vi "Omniax_MotorDrive_XYZR_20100915.vi"() -> ()   [LabVIEW 2009]
uses:
  <vilib>/Utility/file.llb/Read From Spreadsheet File (DBL).vi
  <vilib>/Utility/file.llb/Read From Spreadsheet File (string).vi
  <vilib>/Instr/_visa.llb/VISA Configure Serial Port (Instr).vi
  <vilib>/Utility/file.llb/Write To Spreadsheet File (string).vi
  <vilib>/Utility/file.llb/Write To Spreadsheet File (DBL).vi
panel:
  out "Scanning":bool
  out "HOMING REQ":bool
  out "Laser Shutter":bool
  in  "SHUTTER SYNC":bool
  in  "Laser Shutter":bool
  out "LOOP REQ":bool
  out "#th loop":dbl
  in  "# of loops":dbl
  in  "LOOP":bool
  out "OP":bool
  out "CL":bool
  out "Valve \nopend/closed":bool
  in  "OK Button":bool
  out "STATUS":string
  in  "Delete Button":bool
  in  "String":string
  in  "Add Button":bool
  in  "Set Button":bool
  in  "Preset positions":i32(ring) items=["ZERO", "Default", "CDOSE", "QMS", "test", "test2", "test3", "yag position", "Sample Long Edge  ", "SPUTTER POS"]
  out "Presets":i32[][](array[numeric])
  out "X MINPOS":i32=-94296
  out "X MAXPOS":i32=-34296
  out "Y MINPOS":i32=-94296
  out "Y MAXPOS":i32=-34296
  out "R MAXPOS":i32=-34296
  out "R MINPOS":i32=-94296
  out "Z MINPOS":i32=-94296
  out "Z MAXPOS":i32=-34296
  in  "HARDSTOP":bool
  in  "GO":bool
  out "XYZR VEL PV Array":i32[](array[numeric])
  out "XYZ in RANGE Array":bool[](array[boolean])
  out "STEP SP Array":i32[](array[numeric])
  out "RUNHOLDArray":i32[](array[numeric])
  out "ZCONSTArray":dbl[](array[numeric])
  out "RCONSTArray":dbl[](array[numeric])
  out "XCONSTArray":dbl[](array[numeric])
  out "YCONSTArray":dbl[](array[numeric])
  out "Error Array":errorcluster[](array[cluster])
  out "COM PORT Array":refnum<visa-resource-name>[](array[refnum])
  out "Z COM PORT":refnum<visa-resource-name>="COM6"
  in  "Tab Control 3":enum32{"Status", "Reset"}(tab)
  out "Y in Range":bool
  out "Y Scan":bool
  out "Y in Motion":bool
  out "Y Backlash corr":bool
  out "X  in Range":bool
  out "X Scan":bool
  out "X  in Motion":bool
  out "X Backlash corr":bool
  out "Z in Range":bool
  out "Z Scan":bool
  out "Z in Motion":bool
  out "Z Backlash corr":bool
  out "R in Range":bool
  out "R Scan":bool
  out "R in Motion":bool
  out "R Backlash corr":bool
  out "X Ready":bool
  out "Y Ready":bool
  out "Z Ready":bool
  out "R Ready":bool
  in  "Reset Y Position mm":dbl
  out "Reset Y Motor Steps":i32
  in  "Reset X Position mm":dbl
  out "Reset X Motor Steps":i32
  in  "Reset Z Position mm":dbl
  out "Reset Z Motor Steps":i32
  in  "Reset R Position deg":dbl
  out "Reset R Motor Steps":i32
  in  "Reset":bool
  in  "Tab Control 2":enum32{"mm", "step"}(tab)
  in  "X Scan Length SP mm":dbl
  in  "X Scan Velocity SP mm/sec":dbl
  in  "Y Scan Length SP mm":dbl
  in  "Y Scan Velocity SP mm/sec":dbl
  in  "Review Scan \nParameters":bool
  in  "Z Scan Length SP mm":dbl
  in  "Z Scan Velocity SP mm/sec":dbl
  in  "R Scan Length SP deg":dbl
  in  "R Scan Velocity SP deg/sec":dbl
  in  "Z as dominating length":bool
  in  "X Scan Velocity SP steps/sec":i32=1 min=1 max=102400 step=1
  in  "X Scan Length SP steps":i32 min=-2304000 max=2304000 step=100
  out "X Scan length MV mm":dbl
  out "X Scan velocity MV mm/sec":dbl format="%#_6f"
  in  "Y Scan Velocity SP steps/sec":i32=1 min=1 max=102400 step=1
  in  "Y Scan Length SP steps":i32 min=-2304000 max=2304000 step=100
  out "Y Scan length MV mm":dbl
  out "Y Scan velocity MV mm/sec":dbl format="%#_6f"
  in  "Z Scan Velocity SP steps/sec":i32=1 min=1 max=204800 step=1
  in  "Z Scan Length SP steps":i32 min=0 max=102400000 step=100
  out "Z Scan length MV mm":dbl
  out "Z Scan velocity MV mm/sec":dbl format="%#_6f"
  in  "R Scan Velocity SP steps/sec":i32=1 min=1 max=102400 step=1
  in  "R Scan Length SP steps":i32 min=-6144000 max=0 step=100
  out "R Scan length MV deg":dbl
  out "R Scan velocity MV deg/sec":dbl format="%#_6f"
  out "atan Y/Z":dbl
  in  "Tab Control":enum32{"mm", "step"}(tab)
  in  "X Position SP mm":dbl
  in  "X Velocity SP mm/sec":dbl
  in  "X Move Set":bool
  in  "Y Move Set":bool
  in  "Y Position SP mm":dbl
  in  "Y Velocity SP mm/sec":dbl
  in  "Z Position SP mm":dbl
  in  "Z Velocity SP mm/sec":dbl
  in  "Z Move Set":bool
  in  "R Position SP deg":dbl
  in  "R Velocity SP deg/sec":dbl
  in  "R Move Set":bool
  in  "X Velocity SP step/sec":i32 min=1 max=128000
  out "X Velocity MV mm/sec":dbl
  in  "Y Velocity SP step/sec":i32 min=1 max=128000
  out "Y Velocity MV mm/sec":dbl
  in  "Z Velocity SP step/sec":i32 min=1 max=204800
  out "Z Velocity MV mm/sec":dbl
  in  "R Velocity SP step/sec":i32 min=1 max=20000
  out "R Velocity MVdeg/sec":dbl
  in  "Y Step SP":i32=-20000 min=-2304000 max=2304000 step=500
  out "Y Position MV mm":dbl
  in  "X Step SP":i32=-20000 min=-2304000 max=2304000 step=500
  out "X Position MV mm":dbl
  in  "Z Step SP":i32=-20000 min=0 max=102400000 step=500
  out "Z Position MV mm":dbl
  in  "R Step SP":i32=-20000 min=-6144000 max=0 step=500
  out "R Position MV deg":dbl
  out "X Step PV":i32 max=2000
  out "Y Step PV":i32 max=2000
  out "Z Step PV":i32 max=2000
  out "R Step PV":i32 max=2000
  in  "Clear ZY":bool
  out "ZY Graph":cluster{dbl[], dbl[]}(graph)
  out "ZR Graph":cluster{"Y":dbl[], "Y":dbl[]}[](graph)
  out "XY Graph":cluster{"Y":dbl[], "Y":dbl[]}[](graph)
  out "X Scan Duration":dbl
  out "Y Scan Duration":dbl
  out "Z Scan Duration":dbl
  out "R Scan Duration":dbl
  out "R Backlash steps/sec":i32
  out "R Backlash":i32
  out "R Holding Current %":i32
  out "R Run Current %":i32
  out "R offset deg":dbl
  out "R deg/rev":dbl
  out "R steps/rev":u32
  out "R velocity PV step/sec":i32
  out "R COM PORT":refnum<visa-resource-name>="COM5"
  out "R Position deg PV":dbl
  out "Z Backlash steps/sec":i32
  out "Z Backlash":i32
  out "Z Holding Current %":i32
  out "Z Run Current %":i32
  out "Z offset mm":dbl
  out "Z mm/rev":dbl
  out "Z steps/rev":u32
  out "Z  velocity PV step/sec":i32
  out "Z Position mm PV":dbl
  out "X Position mm PV":dbl
  out "X velocity PV step/sec":i32
  in  "Set scan parameter":bool
  out "X Backlash steps/sec":i32
  out "X Backlash":i32
  out "X Holding Current %":i32
  out "X Run Current %":i32
  out "X offset mm":dbl
  out "X mm/rev":dbl
  out "X steps/rev":u32
  out "X COM PORT":refnum<visa-resource-name>="COM5"
  out "Y Backlash steps/sec":i32
  out "Y Backlash":i32
  out "Y Holding Current %":i32
  out "Y Run Current %":i32
  in  "Scan Cancel":bool
  out "Y Position mm PV":dbl
  out "Y offset mm":dbl
  out "Y mm/rev":dbl
  out "Y steps/rev":u32
  out "Y velocity PV step/sec":i32
  in  "Scan Go":bool
  in  "Stop":bool
  out "Y COM PORT":refnum<visa-resource-name>="COM5"
  # "MX"
  # "MY"
  # "MZ"
  # "MR"
  # "Indicators"
  # "L"
  # "M"
  # "B"
  # "S"
  # "R"
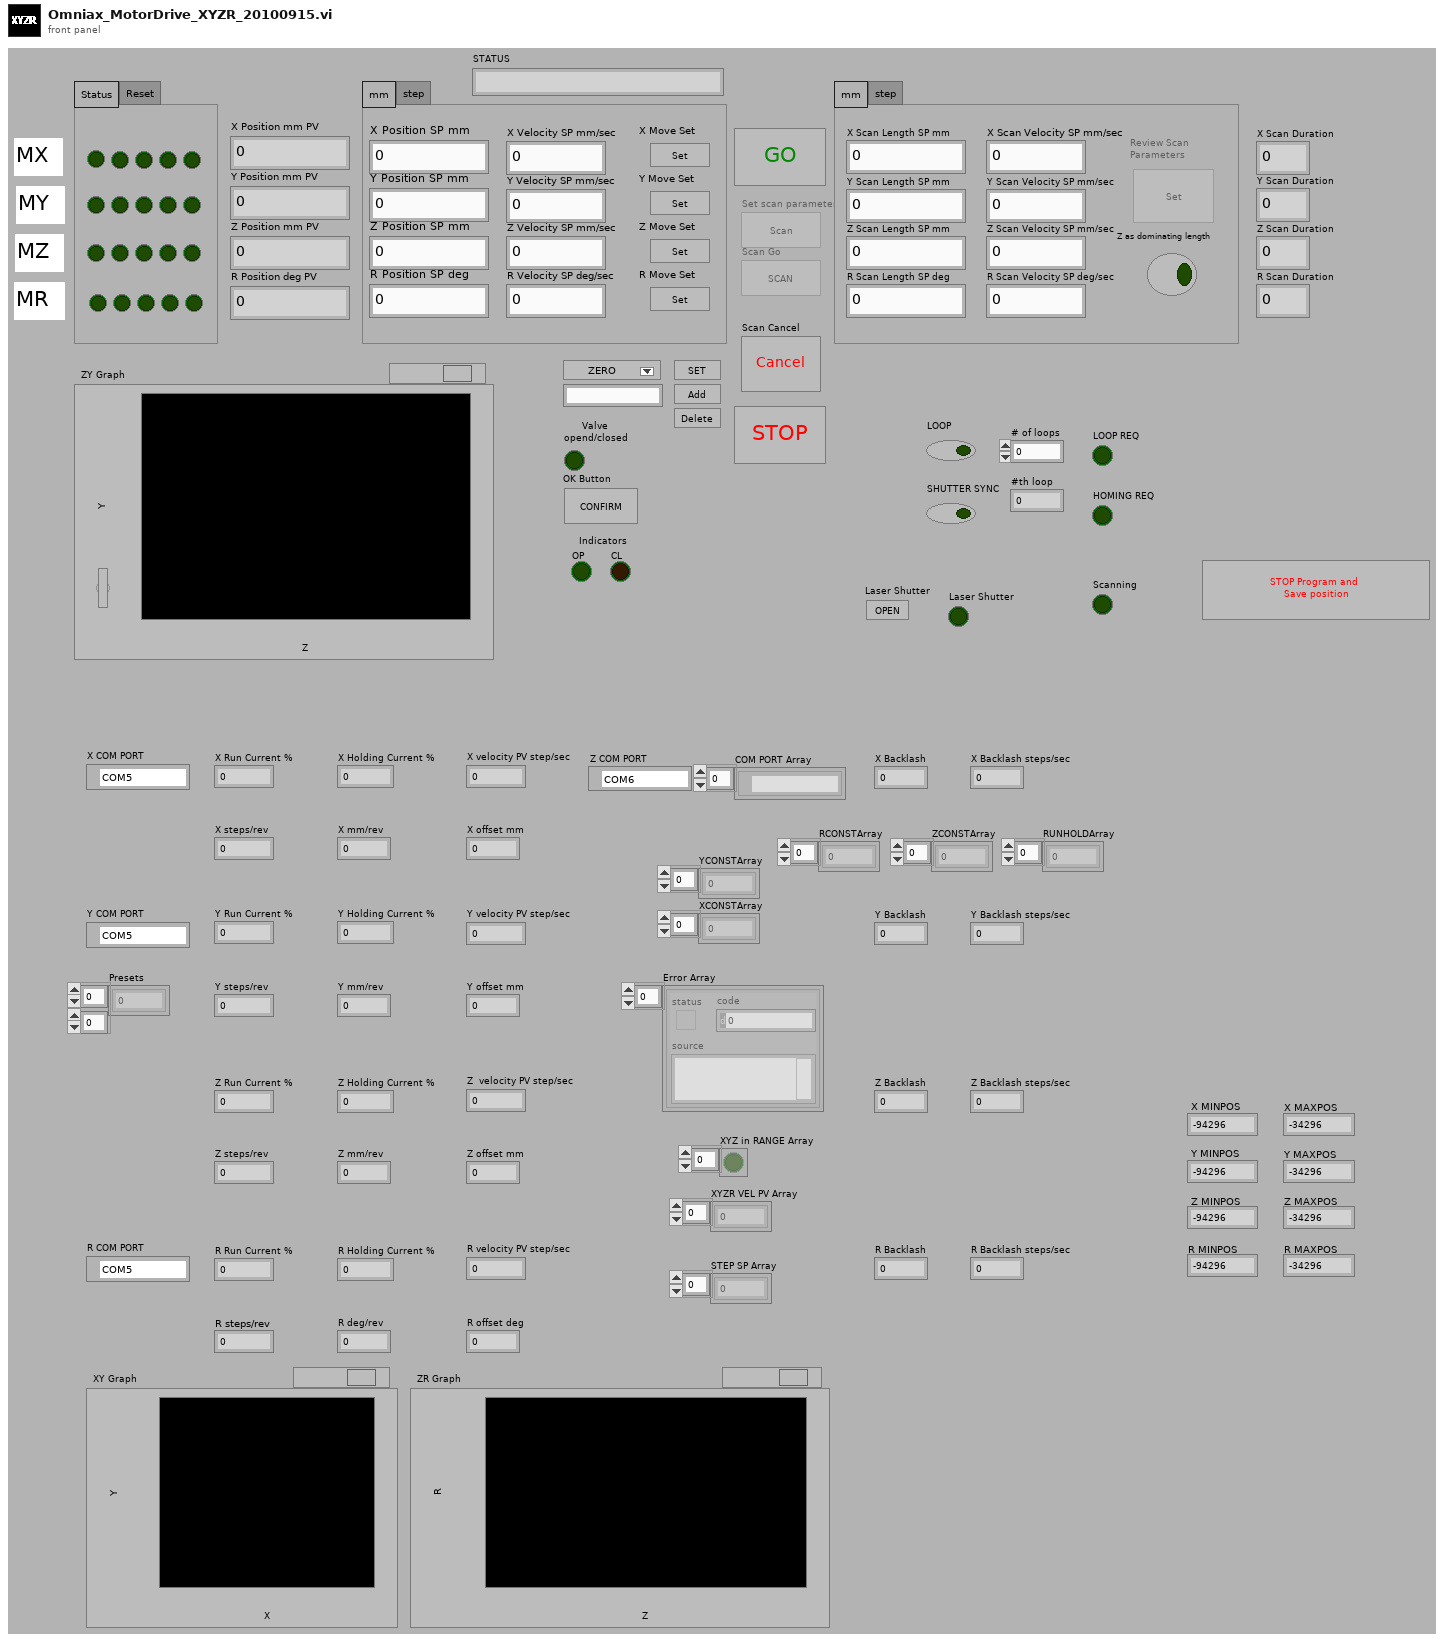
[diagram p1: front panel]
types:
  T1 = enum8{"Enabled", "Disabled", "Disabled and Grayed Out"}
  T2 = cluster{"[0]":i32, "[1]":i32, "[2]":i32, "[3]":i32, "[4]":i32, "[5]":i32, "[6]":i32, "[7]":i32, "[8]":i32}
  T3 = cluster{"XY Max Min array OUT[0]":dbl, "XY Max Min array OUT[1]":dbl, "XY Max Min array OUT[2]":dbl, "XY Max Min array OUT[3]":dbl, "XY Max Min array OUT[4]":dbl, "XY Max Min array OUT[5]":dbl, "XY Max Min array OUT[6]":dbl, "XY Max Min array OUT[7]":dbl, "XY Max Min array OUT[8]":dbl}
  T4 = cluster{"COM PORT Array OUT[0]":refnum<visa-resource-name>, "COM PORT Array OUT[1]":refnum<visa-resource-name>, "COM PORT Array OUT[2]":refnum<visa-resource-name>, "COM PORT Array OUT[3]":refnum<visa-resource-name>, "COM PORT Array OUT[4]":refnum<visa-resource-name>, "COM PORT Array OUT[5]":refnum<visa-resource-name>, "COM PORT Array OUT[6]":refnum<visa-resource-name>, "COM PORT Array OUT[7]":refnum<visa-resource-name>, "COM PORT Array OUT[8]":refnum<visa-resource-name>}
  T5 = cluster{"STEP SP Array OUT[0]":i32, "STEP SP Array OUT[1]":i32, "STEP SP Array OUT[2]":i32, "STEP SP Array OUT[3]":i32, "STEP SP Array OUT[4]":i32, "STEP SP Array OUT[5]":i32, "STEP SP Array OUT[6]":i32, "STEP SP Array OUT[7]":i32, "STEP SP Array OUT[8]":i32}
  T6 = cluster{"XYZ in RANGE Array OUT[0]":bool, "XYZ in RANGE Array OUT[1]":bool, "XYZ in RANGE Array OUT[2]":bool, "XYZ in RANGE Array OUT[3]":bool, "XYZ in RANGE Array OUT[4]":bool, "XYZ in RANGE Array OUT[5]":bool, "XYZ in RANGE Array OUT[6]":bool, "XYZ in RANGE Array OUT[7]":bool, "XYZ in RANGE Array OUT[8]":bool}
  T7 = cluster{"XYZR VEL PV Array OUT[0]":i32, "XYZR VEL PV Array OUT[1]":i32, "XYZR VEL PV Array OUT[2]":i32, "XYZR VEL PV Array OUT[3]":i32, "XYZR VEL PV Array OUT[4]":i32, "XYZR VEL PV Array OUT[5]":i32, "XYZR VEL PV Array OUT[6]":i32, "XYZR VEL PV Array OUT[7]":i32, "XYZR VEL PV Array OUT[8]":i32}
  T8 = cluster{"XYZR MAX MIN POS[0]":i32, "XYZR MAX MIN POS[1]":i32, "XYZR MAX MIN POS[2]":i32, "XYZR MAX MIN POS[3]":i32, "XYZR MAX MIN POS[4]":i32, "XYZR MAX MIN POS[5]":i32, "XYZR MAX MIN POS[6]":i32, "XYZR MAX MIN POS[7]":i32, "XYZR MAX MIN POS[8]":i32}
  T9 = cluster{"Error Array OUT[0]":errorcluster, "Error Array OUT[1]":errorcluster, "Error Array OUT[2]":errorcluster, "Error Array OUT[3]":errorcluster, "Error Array OUT[4]":errorcluster, "Error Array OUT[5]":errorcluster, "Error Array OUT[6]":errorcluster, "Error Array OUT[7]":errorcluster, "Error Array OUT[8]":errorcluster}
  T10 = enum16{"Stop", "Reset", "Run Current", "Holding Current", "Accel Rate", "Decel Rate", "Move to Relative Position", "Move to Absolute Position", "Echo Mode", "Print Parameter", "Send String", "Microstep Resolution", "Set Current Position", "Max Velocity"}
  T11 = cluster{"Presets[0]":i32, "Presets[1]":i32, "Presets[2]":i32, "Presets[3]":i32, "Presets[4]":i32, "Presets[5]":i32, "Presets[6]":i32, "Presets[7]":i32, "Presets[8]":i32}
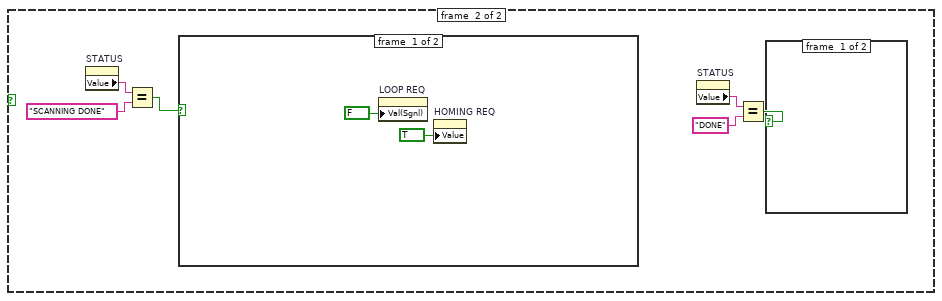
[diagram p4: hidden frame]
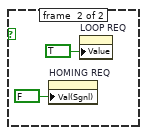
[diagram p5: hidden frame]
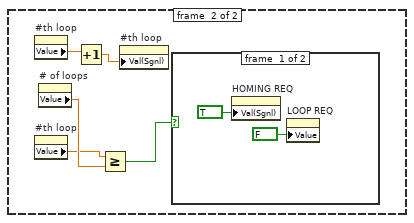
[diagram p6: hidden frame]
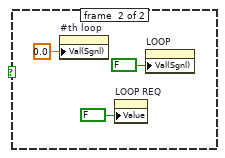
[diagram p7: hidden frame]
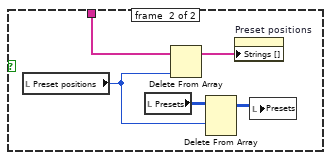
[diagram p8: hidden frame]
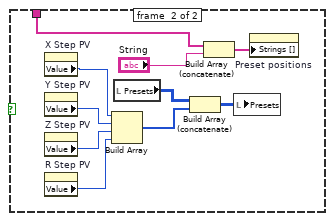
[diagram p9: hidden frame]
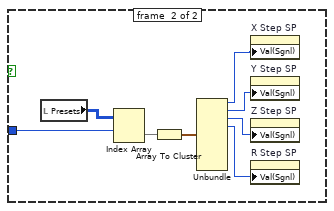
[diagram p10: hidden frame]
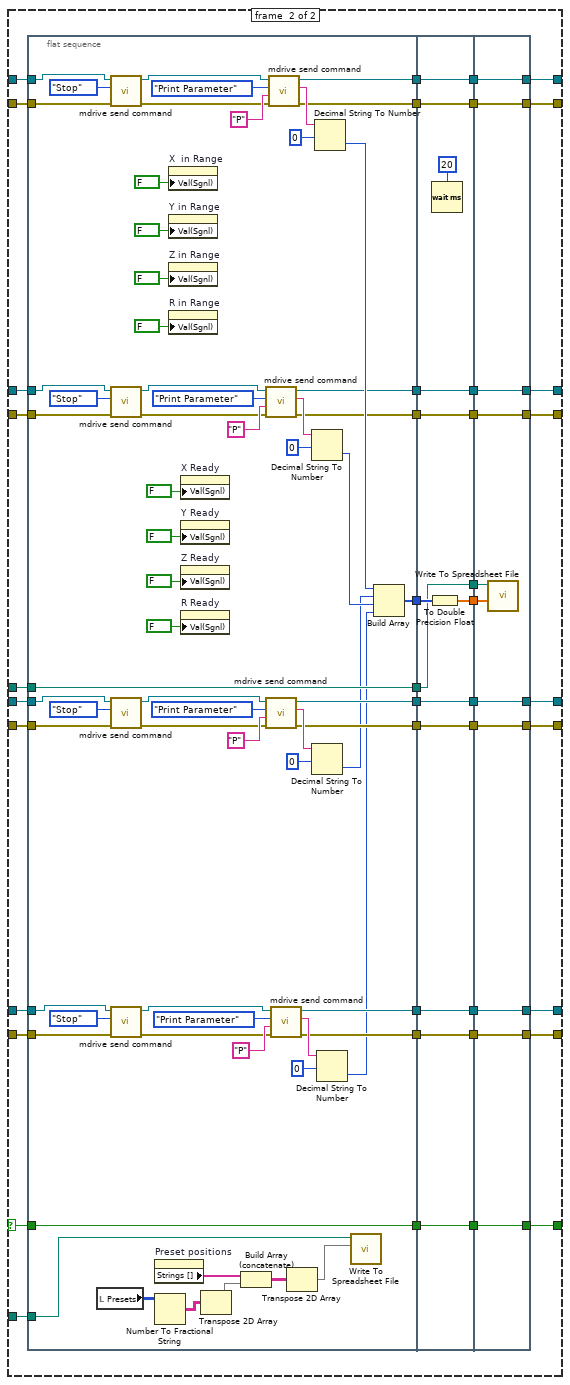
[diagram p11: hidden frame]
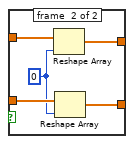
[diagram p12: hidden frame]
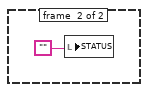
[diagram p14: hidden frame]
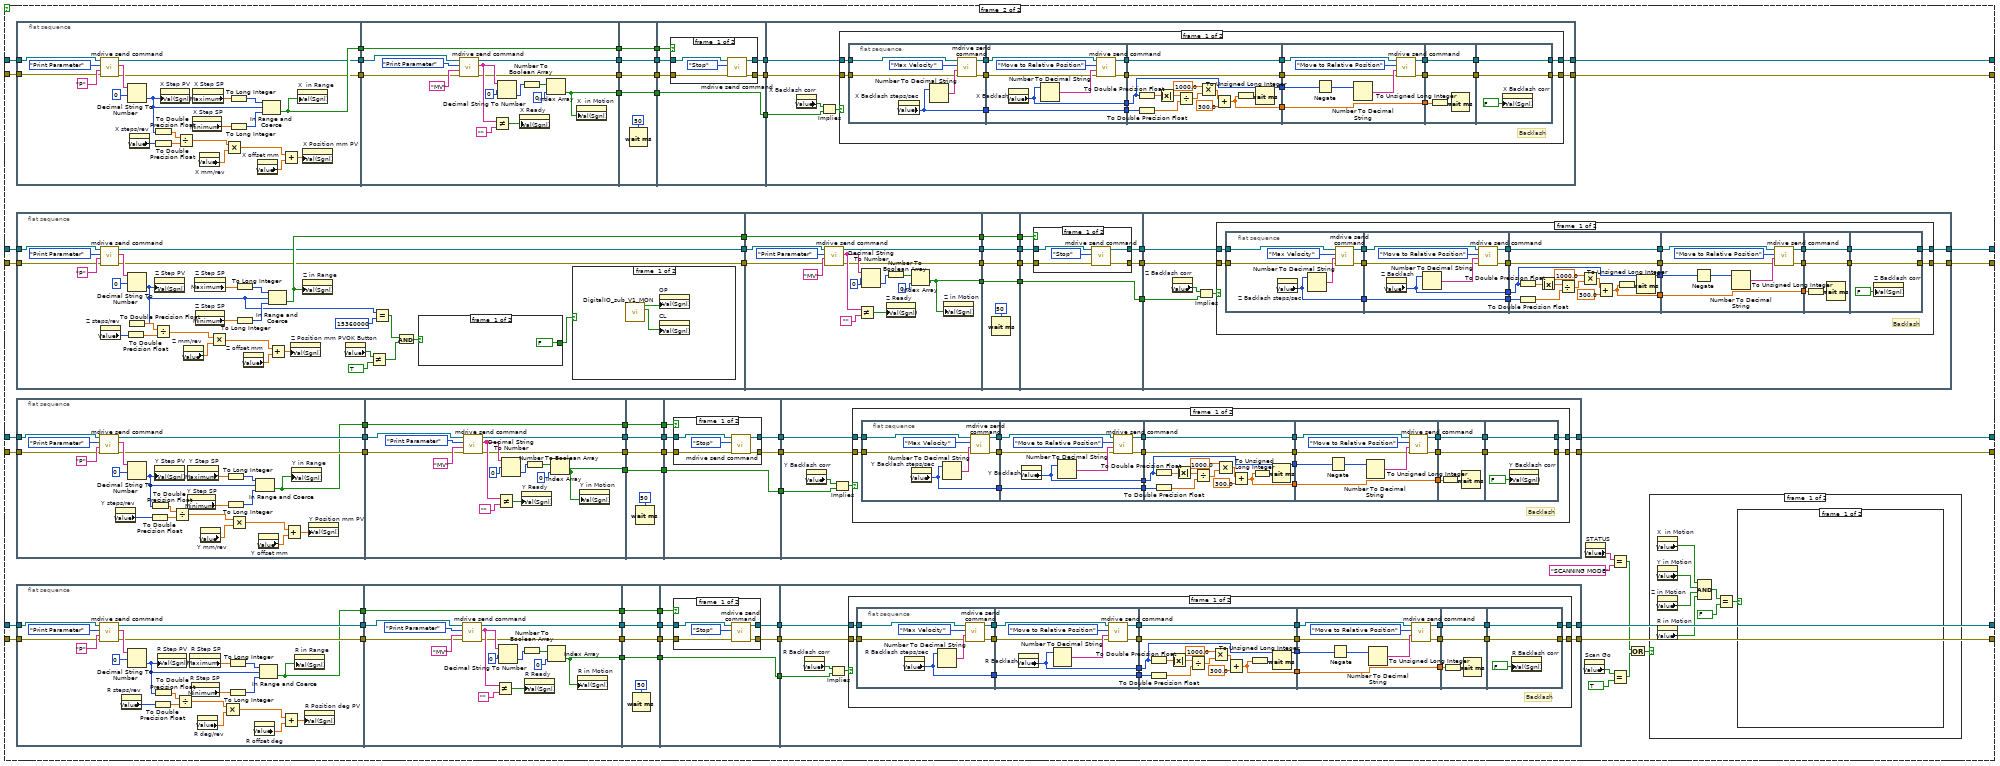
[diagram p15: hidden frame]
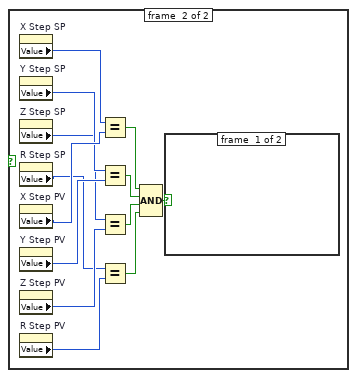
[diagram p16: hidden frame]
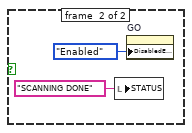
[diagram p17: hidden frame]
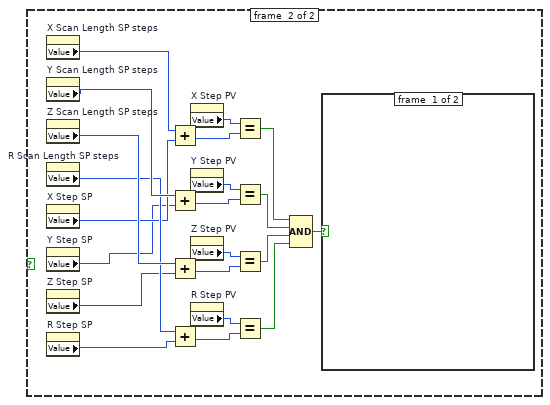
[diagram p18: hidden frame]
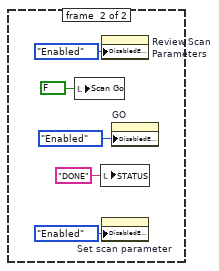
[diagram p19: hidden frame]
diagram:
  n1 = flat-sequence {
    tunnel: [w53] -> w36
    frame #0 {
      w51 = 0.2 ("MM/rev")
      w56 = u32 51200 ("step/rev")
      w58 = 128000 ("Value (Signaling)")
      w59 = 1.0 ("Data Entry Limits:Minimum")
      w52 = 0.0 ("offset")
      # "a=1000000"
      n2 = To Double Precision Float(number=w58) -> (double precision float=w50:dbl)
      n3 = To Double Precision Float(number=w56) -> (double precision float=w61:dbl)
      n4 = property on="X Velocity SP step/sec" class="DigNum (strict)"("Val(Sgnl)"=w58) -> ()  [unwired: 2 in, 2 out]
      n5 = property on="X Velocity SP step/sec" class="DigNum (strict)"("Minimum"=w59) -> ()  [unwired: 2 in, 2 out]
      n6 = Divide(x=w50, y=w61) -> (x/y=w60:dbl)
      n7 = property on="X Velocity SP step/sec" class="DigNum (strict)"("Maximum"=w50) -> ()  [unwired: 2 in, 2 out]
      n8 = Multiply(x=w60, y=w51) -> (x*y=w54:dbl)
      n9 = property on="X Velocity SP mm/sec" class="DigNum (strict)"("Val(Sgnl)"=w54) -> ()  [unwired: 2 in, 2 out]
      n10 = To Double Precision Float(number=w56) -> (double precision float=w55:dbl)
      n11 = To Double Precision Float(number=w58) -> (double precision float=w57:dbl)
      n12 = Build Array(w59, w57, w55, w54, w50, w51, w52) -> (w53:dbl[])
      "X offset mm" <- w52
      "X steps/rev" <- w56
      "X mm/rev" <- w51
    }
  }
  n13 = flat-sequence {
    tunnel: [w62] -> w35
    frame #0 {
      w71 = 1.0 ("Data Entry Limits:Minimum")
      w65 = 0.0 ("R offset deg")
      w66 = -3.0 ("R deg/rev")
      w69 = u32 51200 ("step/rev")
      w70 = 20000 ("Value (Signaling)")
      n14 = To Double Precision Float(number=w69) -> (double precision float=w72:dbl)
      n15 = To Double Precision Float(number=w70) -> (double precision float=w68:dbl)
      n16 = property on="R Velocity SP step/sec" class="DigNum (strict)"("Minimum"=w71) -> ()  [unwired: 2 in, 2 out]
      n17 = property on="R Velocity SP step/sec" class="DigNum (strict)"("Val(Sgnl)"=w70) -> ()  [unwired: 2 in, 2 out]
      n18 = Divide(x=w68, y=w72) -> (x/y=w74:dbl)
      n19 = property on="R Velocity SP step/sec" class="DigNum (strict)"("Maximum"=w68) -> ()  [unwired: 2 in, 2 out]
      n20 = Multiply(x=w74, y=w66) -> (x*y=w73:dbl)
      n21 = Absolute Value(x=w73) -> (abs(x)=w67:dbl)
      n22 = property on="R Velocity SP deg/sec" class="DigNum (strict)"("Val(Sgnl)"=w67) -> ()  [unwired: 2 in, 2 out]
      n23 = To Double Precision Float(number=w69) -> (double precision float=w63:dbl)
      n24 = To Double Precision Float(number=w70) -> (double precision float=w64:dbl)
      n25 = Build Array(w71, w64, w63, w68, w67, w66, w65) -> (w62:dbl[])
      "R offset deg" <- w65
      "R deg/rev" <- w66
      "R steps/rev" <- w69
    }
  }
  n26 = flat-sequence {
    tunnel: [w75] -> w34
    frame #0 {
      w77 = 0.2 ("Z mm/rev")
      w81 = u32 51200 ("step/rev")
      w83 = 204800 ("Value (Signaling)")
      w84 = 1.0 ("Data Entry Limits:Minimum")
      w76 = 0.0 ("Z offset mm")
      n27 = To Double Precision Float(number=w81) -> (double precision float=w86:dbl)
      n28 = To Double Precision Float(number=w83) -> (double precision float=w79:dbl)
      n29 = property on="Z Velocity SP step/sec" class="DigNum (strict)"("Minimum"=w84) -> ()  [unwired: 2 in, 2 out]
      n30 = property on="Z Velocity SP step/sec" class="DigNum (strict)"("Val(Sgnl)"=w83) -> ()  [unwired: 2 in, 2 out]
      n31 = Divide(x=w79, y=w86) -> (x/y=w85:dbl)
      n32 = property on="Z Velocity SP step/sec" class="DigNum (strict)"("Maximum"=w79) -> ()  [unwired: 2 in, 2 out]
      n33 = Multiply(x=w85, y=w77) -> (x*y=w78:dbl)
      n34 = property on="Z Velocity SP mm/sec" class="DigNum (strict)"("Val(Sgnl)"=w78) -> ()  [unwired: 2 in, 2 out]
      n35 = To Double Precision Float(number=w83) -> (double precision float=w82:dbl)
      n36 = To Double Precision Float(number=w81) -> (double precision float=w80:dbl)
      n37 = Build Array(w84, w82, w80, w79, w78, w77, w76) -> (w75:dbl[])
      "Z offset mm" <- w76
      "Z mm/rev" <- w77
      "Z steps/rev" <- w81
    }
  }
  n38 = flat-sequence {
    tunnel: [w90] -> w37
    frame #0 {
      w88 = 0.2 ("MM/rev")
      w93 = u32 51200 ("step/rev")
      w95 = 128000 ("Value (Signaling)")
      w96 = 1.0 ("Data Entry Limits:Minimum")
      w89 = 0.0 ("offset")
      n39 = To Double Precision Float(number=w95) -> (double precision float=w87:dbl)
      n40 = To Double Precision Float(number=w93) -> (double precision float=w98:dbl)
      n41 = property on="Y Velocity SP step/sec" class="DigNum (strict)"("Val(Sgnl)"=w95) -> ()  [unwired: 2 in, 2 out]
      n42 = property on="Y Velocity SP step/sec" class="DigNum (strict)"("Minimum"=w96) -> ()  [unwired: 2 in, 2 out]
      n43 = Divide(x=w87, y=w98) -> (x/y=w97:dbl)
      n44 = property on="Y Velocity SP step/sec" class="DigNum (strict)"("Maximum"=w87) -> ()  [unwired: 2 in, 2 out]
      n45 = Multiply(x=w97, y=w88) -> (x*y=w91:dbl)
      n46 = To Double Precision Float(number=w95) -> (double precision float=w94:dbl)
      n47 = property on="Y Velocity SP mm/sec" class="DigNum (strict)"("Val(Sgnl)"=w91) -> ()  [unwired: 2 in, 2 out]
      n48 = To Double Precision Float(number=w93) -> (double precision float=w92:dbl)
      n49 = Build Array(w96, w94, w92, w91, w87, w88, w89) -> (w90:dbl[])
      "Y offset mm" <- w89
      "Y steps/rev" <- w93
      "Y mm/rev" <- w88
    }
  }
  n50 = local read "Z  velocity PV step/sec"() -> (w17:i32)
  n51 = local read "R velocity PV step/sec"() -> (w19:i32)
  n52 = local read "X velocity PV step/sec"() -> (w20:i32)
  n53 = local read "Y velocity PV step/sec"() -> (w18:i32)
  n54 = local read "X  in Range"() -> (w24:bool)
  n55 = local read "R in Range"() -> (w21:bool)
  n56 = local read "Y in Range"() -> (w23:bool)
  n57 = local read "Z in Range"() -> (w22:bool)
  n58 = property on="LOOP REQ" class="Bool (strict)"("Value"=FALSE ("LOOP MODE")) -> ()  [unwired: 2 in, 2 out]
  n59 = Build Array(w20, w18, w17, w19) -> (→"XYZR VEL PV Array":i32[])
  n60 = Build Array(w24, w23, w22, w21) -> (→"XYZ in RANGE Array":bool[])
  n61 = flat-sequence {
    tunnel: [w99] -> w33
    frame #0 {
      w102 = 20 ("R Holding Current %")
      w101 = 100 ("R Run Current %")
      w104 = 20 ("Holding Current %")
      w103 = 40 ("Run Current %")
      w106 = 20 ("Holding Current %")
      w107 = 40 ("Run Current %")
      w105 = 40 ("Z Run Current %")
      w100 = 20 ("Z Holding Current %")
      n62 = Build Array(w107, w106, w105, w104, w103, w102, w101, w100) -> (w99:i32[])
      "Z Holding Current %" <- w100
      "Z Run Current %" <- w105
      "X Run Current %" <- w107
      "X Holding Current %" <- w106
      "Y Run Current %" <- w103
      "Y Holding Current %" <- w104
      "R Holding Current %" <- w102
      "R Run Current %" <- w101
    }
  }
  n63 = Build Array("X Step SP", "Y Step SP", "Z Step SP", "R Step SP", "X Velocity SP step/sec", "Y Velocity SP step/sec", "Z Velocity SP step/sec", "R Velocity SP step/sec") -> (→"STEP SP Array":i32[])
  n64 = flat-sequence {
    frame #0 {
      n65 = property on="Z Scan" class="Bool (strict)"("Val(Sgnl)"=FALSE ("Value (Signaling)")) -> ()  [unwired: 2 in, 2 out]
      n66 = property on="R Velocity SP deg/sec" class="DigNum (strict)"("Val(Sgnl)"=0.1 ("Value (Signaling)")) -> ()  [unwired: 2 in, 2 out]
      n67 = property on="Z Scan Velocity SP mm/sec" class="DigNum (strict)"("Val(Sgnl)"=0.1 ("Value (Signaling)")) -> ()  [unwired: 2 in, 2 out]
      n68 = property on="X Scan" class="Bool (strict)"("Val(Sgnl)"=FALSE ("Value (Signaling)")) -> ()  [unwired: 2 in, 2 out]
      n69 = property on="R Scan" class="Bool (strict)"("Val(Sgnl)"=FALSE ("Value (Signaling)")) -> ()  [unwired: 2 in, 2 out]
      n70 = property on="Y Scan Velocity SP mm/sec" class="DigNum (strict)"("Val(Sgnl)"=0.1 ("Value (Signaling)")) -> ()  [unwired: 2 in, 2 out]
      n71 = property on="Y Scan" class="Bool (strict)"("Val(Sgnl)"=FALSE ("Value (Signaling)")) -> ()  [unwired: 2 in, 2 out]
      n72 = property on="X Scan Velocity SP mm/sec" class="DigNum (strict)"("Val(Sgnl)"=0.1 ("Value (Signaling)")) -> ()  [unwired: 2 in, 2 out]
      n73 = property on="Scan Go" class="Bool (strict)"("DisabledEnum"=T1."Disabled and Grayed Out" ("Disabled")) -> ()  [unwired: 2 in, 2 out]
      n74 = property on="Z Scan Velocity SP steps/sec" class="DigNum (strict)"("Minimum"=1.0 ("Data Entry Limits:Maximum")) -> ()  [unwired: 2 in, 2 out]
      n75 = property on="Z Scan Velocity SP steps/sec" class="DigNum (strict)"("Maximum"=204800.0 ("Data Entry Limits:Maximum")) -> ()  [unwired: 2 in, 2 out]
    }
  }
  n76 = flat-sequence {
    frame #0 {
      n77 = property on="R Backlash corr" class="Bool (strict)"("Val(Sgnl)"=FALSE ("Value (Signaling)")) -> ()  [unwired: 2 in, 2 out]
      n78 = property on="Y Backlash corr" class="Bool (strict)"("Val(Sgnl)"=FALSE ("Value (Signaling)")) -> ()  [unwired: 2 in, 2 out]
      n79 = property on="Z Backlash corr" class="Bool (strict)"("Val(Sgnl)"=FALSE ("Value (Signaling)")) -> ()  [unwired: 2 in, 2 out]
      n80 = property on="X Backlash corr" class="Bool (strict)"("Val(Sgnl)"=FALSE ("Value (Signaling)")) -> ()  [unwired: 2 in, 2 out]
      "Z Backlash steps/sec" <- 25600 ("Z Backlash steps/sec")
      "Z Backlash" <- -12800 ("Z Backlash")
      "X Backlash steps/sec" <- 25600 ("Value (Signaling)")
      "X Backlash" <- 5120 ("Backlash2")
      "Y Backlash" <- -5120 ("Backlash2")
      "Y Backlash steps/sec" <- 25600 ("Value (Signaling)")
      "R Backlash steps/sec" <- 6400 ("R Backlash steps/sec")
      "R Backlash" <- -12800 ("R Backlash")
    }
  }
  n81 = flat-sequence {
    tunnel: [w225] -> w13
    tunnel: [w224] -> w12
    tunnel: [w223] -> w11
    tunnel: [w222] -> w10
    tunnel: [w221] -> w9
    tunnel: [w220] -> w8
    tunnel: [w219] -> w7
    tunnel: [w218] -> w6
    tunnel: [w215] -> w5
    tunnel: [w185] -> w4
    frame #0 {
      w185 = path "C:/Documents and Settings/b_ogasawara/Desktop/lv1/LV codes/IMS/PRESET.TXT"
      w183 = 0 ("element")
      w215 = path "C:/Documents and Settings/b_ogasawara/Desktop/lv1/LV codes/IMS/POS.TXT"
      w245 = refnum<visa-resource-name> "COM7" ("COM PORT")
      w246 = refnum<visa-resource-name> "COM5" ("COM PORT")
      w247 = refnum<visa-resource-name> "COM6" ("VISA resource name")
      w248 = refnum<visa-resource-name> "COM4" ("COM PORT")
      n82 = Build Array(w248, w247, w246, w245) -> (w243:refnum<visa-resource-name>[])
      n83 = for {
        N: 4 -> [_]
        tunnel: w243 -> [w251] mode=indexing
        tunnel: [w250] -> w241 mode=indexing
        tunnel: [w249] -> w242 mode=indexing
        w253 = u16 0 items=["None", "XON/XOFF", "RTS/CTS", "XON/XOFF & RTS/CTS", "DTR/DSR", "XON/XOFF & DTR/DSR"] ("flow control (0:none)")
        w254 = u16 10 items=["1.0"=10, "1.5"=15, "2.0"=20] ("stop bits (10: 1 bit)")
        # "Stop bits"
        n84 = call-poly "VISA Configure Serial Port"("VISA resource name"=w251, "timeout (10sec)"=u32 10000, "baud rate (9600)"=u32 9600, "data bits (8)"=u16 8, "parity (0:none)"=enum16{"None", "Odd", "Even", "Mark", "Space"}."None", "stop bits (10: 1 bit)"=w254, "flow control (0:none)"=w253) -> ("VISA resource name out"=w250:refnum<visa-resource-name>, "error out"=w249:errorcluster)  [unwired: 7 in]
      }
      "COM PORT Array" <- w241
      "Error Array" <- w242
      n85 = local write "STATUS"("INITIALIZING" ("STATUS")) -> ()
      n86 = call-poly <vilib>:"Read From Spreadsheet File.vi"("file path (dialog if empty)"=w215) -> ("first row"=w216:dbl[])  [unwired: 6 in, 4 out]
      n87 = call "DigitalIO_sub_V1_MON.vi"() -> ("CL"=w142:bool, "OP"=w143:bool)  [unwired: 8 in]
      n88 = To Long Integer(number=w216) -> (32bit integer=w182:i32[])
      n89 = property on="CL" class="Bool (strict)"("Val(Sgnl)"=w142) -> ()  [unwired: 2 in, 2 out]
      n90 = property on="OP" class="Bool (strict)"("Val(Sgnl)"=w143) -> ()  [unwired: 2 in, 2 out]
      n91 = Array To Cluster(array=w182) -> (cluster=w181:T2)
      n92 = property on="Z Step SP" class="DigNum (strict)"() -> ("Maximum"=w140:dbl)  [unwired: 2 in, 2 out]
      n93 = property on="R Step SP" class="DigNum (strict)"() -> ("Maximum"=w138:dbl)  [unwired: 2 in, 2 out]
      n94 = property on="R Step SP" class="DigNum (strict)"() -> ("Minimum"=w139:dbl)  [unwired: 2 in, 2 out]
      n95 = property on="Z Step SP" class="DigNum (strict)"() -> ("Minimum"=w141:dbl)  [unwired: 2 in, 2 out]
      n96 = Unbundle(w181) -> ("[0]"=w157:i32, "[1]"=w158:i32, "[2]"=w159:i32, "[3]"=w160:i32)  [unwired: 5 out]
      n97 = Build Array(w140, w141, w138, w139) -> (w137:dbl[])
      n98 = property on="Reset X Motor Steps" class="DigNum (strict)"("Val(Sgnl)"=w157) -> ()  [unwired: 2 in, 2 out]
      n99 = property on="Reset Y Motor Steps" class="DigNum (strict)"("Val(Sgnl)"=w158) -> ()  [unwired: 2 in, 2 out]
      n100 = property on="Reset Z Motor Steps" class="DigNum (strict)"("Val(Sgnl)"=w159) -> ()  [unwired: 2 in, 2 out]
      n101 = property on="Reset R Motor Steps" class="DigNum (strict)"("Val(Sgnl)"=w160) -> ()  [unwired: 2 in, 2 out]
      n102 = local read "XYZ in RANGE Array"() -> (w237:bool[])
      n103 = local read "XYZR VEL PV Array"() -> (w236:i32[])
      n104 = local read "RUNHOLDArray"() -> (w235:i32[])
      n105 = local read "STEP SP Array"() -> (w238:i32[])
      n106 = call-poly <vilib>:"Read From Spreadsheet File.vi"("file path (dialog if empty)"=w185) -> ("all rows"=w190:string[][])  [unwired: 6 in, 4 out]
      n107 = Transpose 2D Array(2D array=w190) -> (transposed array=w189:string[][])
      n108 = property on="R steps/rev" class="DigNum (strict)"() -> ("Value"=w153:u32)  [unwired: 2 in, 2 out]
      n109 = property on="X steps/rev" class="DigNum (strict)"() -> ("Value"=w156:u32)  [unwired: 2 in, 2 out]
      n110 = property on="Y steps/rev" class="DigNum (strict)"() -> ("Value"=w155:u32)  [unwired: 2 in, 2 out]
      n111 = property on="Z steps/rev" class="DigNum (strict)"() -> ("Value"=w154:u32)  [unwired: 2 in, 2 out]
      n112 = Delete From Array(array=w189, index (row)=0) -> (deleted portion=w184:string[], array with subset deleted=w187:string[][])  [unwired: 2 in]
      n113 = call "InitializeMotorsXYZR_V2.vi"("COM PORT Array IN"=w241, "STEP SP Array IN"=w238, "XYZ in RANGE Array IN"=w237, "XYZR VEL PV Array IN"=w236, "RUNHOLDArray IN"=w235, "Error Array IN"=w242, "ZR Max Min array"=w137) -> ("XY Max Min array OUT"=w136:dbl[], "COM PORT Array OUT"=w240:refnum<visa-resource-name>[], "STEP SP Array OUT"=w234:i32[], "XYZ in RANGE Array OUT"=w233:bool[], "XYZR VEL PV Array OUT"=w232:i32[], "XYZR MAX MIN POS"=w217:i32[], "Error Array OUT"=w239:errorcluster[])  [unwired: 6 in]
      n114 = Array To Cluster(array=w136) -> (cluster=w135:T3)
      n115 = Unbundle(w135) -> ("XY Max Min array OUT[0]"=w134:dbl, "XY Max Min array OUT[1]"=w132:dbl, "XY Max Min array OUT[2]"=w131:dbl, "XY Max Min array OUT[3]"=w133:dbl)  [unwired: 5 out]
      n116 = To Double Precision Float(number=w160) -> (double precision float=w166:dbl)
      n117 = To Double Precision Float(number=w153) -> (double precision float=w165:dbl)
      n118 = To Double Precision Float(number=w159) -> (double precision float=w170:dbl)
      n119 = To Double Precision Float(number=w154) -> (double precision float=w169:dbl)
      n120 = To Double Precision Float(number=w158) -> (double precision float=w174:dbl)
      n121 = To Double Precision Float(number=w155) -> (double precision float=w173:dbl)
      n122 = To Double Precision Float(number=w157) -> (double precision float=w178:dbl)
      n123 = To Double Precision Float(number=w156) -> (double precision float=w177:dbl)
      n124 = property on="R deg/rev" class="DigNum (strict)"() -> ("Value"=w149:dbl)  [unwired: 2 in, 2 out]
      n125 = property on="X Step SP" class="DigNum (strict)"("Maximum"=w134) -> ()  [unwired: 2 in, 2 out]
      n126 = property on="X Step SP" class="DigNum (strict)"("Minimum"=w132) -> ()  [unwired: 2 in, 2 out]
      n127 = property on="Y Step SP" class="DigNum (strict)"("Maximum"=w131) -> ()  [unwired: 2 in, 2 out]
      n128 = property on="Y Step SP" class="DigNum (strict)"("Minimum"=w133) -> ()  [unwired: 2 in, 2 out]
      n129 = property on="X mm/rev" class="DigNum (strict)"() -> ("Value"=w150:dbl)  [unwired: 2 in, 2 out]
      n130 = property on="Y mm/rev" class="DigNum (strict)"() -> ("Value"=w151:dbl)  [unwired: 2 in, 2 out]
      n131 = property on="Z mm/rev" class="DigNum (strict)"() -> ("Value"=w152:dbl)  [unwired: 2 in, 2 out]
      n132 = Transpose 2D Array(2D array=w187) -> (transposed array=w186:string[][])
      n133 = property on="Preset positions" class="Ring (strict)"("Strings []"=w184) -> ()  [unwired: 2 in, 2 out]
      n134 = Divide(x=w166, y=w165) -> (x/y=w168:dbl)
      n135 = Array To Cluster(array=w240) -> (cluster=w231:T4)
      n136 = Array To Cluster(array=w234) -> (cluster=w229:T5)
      n137 = Array To Cluster(array=w233) -> (cluster=w228:T6)
      n138 = Array To Cluster(array=w232) -> (cluster=w227:T7)
      n139 = Array To Cluster(array=w217) -> (cluster=w226:T8)
      n140 = Array To Cluster(array=w239) -> (cluster=w230:T9)
      n141 = Divide(x=w170, y=w169) -> (x/y=w172:dbl)
      n142 = Divide(x=w174, y=w173) -> (x/y=w176:dbl)
      n143 = Divide(x=w178, y=w177) -> (x/y=w180:dbl)
      n144 = property on="X offset mm" class="DigNum (strict)"() -> ("Value"=w145:dbl)  [unwired: 2 in, 2 out]
      n145 = property on="Y offset mm" class="DigNum (strict)"() -> ("Value"=w146:dbl)  [unwired: 2 in, 2 out]
      n146 = property on="Z offset mm" class="DigNum (strict)"() -> ("Value"=w147:dbl)  [unwired: 2 in, 2 out]
      n147 = property on="R offset deg" class="DigNum (strict)"() -> ("Value"=w148:dbl)  [unwired: 2 in, 2 out]
      n148 = Decimal String To Number(string=w186) -> (number=w188:i32[][])  [unwired: 2 in, 1 out]
      n149 = Multiply(x=w168, y=w149) -> (x*y=w167:dbl)
      n150 = Multiply(x=w172, y=w152) -> (x*y=w171:dbl)
      n151 = Multiply(x=w176, y=w151) -> (x*y=w175:dbl)
      n152 = Multiply(x=w180, y=w150) -> (x*y=w179:dbl)
      n153 = Add(x=w167, y=w148) -> (x+y=w164:dbl)
      n154 = Add(x=w171, y=w147) -> (x+y=w163:dbl)
      n155 = Add(x=w175, y=w146) -> (x+y=w162:dbl)
      n156 = Add(x=w179, y=w145) -> (x+y=w161:dbl)
      n157 = Unbundle(w231) -> ("COM PORT Array OUT[0]"=w225:refnum<visa-resource-name>, "COM PORT Array OUT[1]"=w224:refnum<visa-resource-name>, "COM PORT Array OUT[2]"=w223:refnum<visa-resource-name>, "COM PORT Array OUT[3]"=w222:refnum<visa-resource-name>)  [unwired: 5 out]
      n158 = Unbundle(w229) -> ("STEP SP Array OUT[0]"=w199:i32, "STEP SP Array OUT[1]"=w200:i32, "STEP SP Array OUT[2]"=w201:i32, "STEP SP Array OUT[3]"=w202:i32)  [unwired: 5 out]
      n159 = Unbundle(w228) -> ("XYZ in RANGE Array OUT[0]"=w214:bool, "XYZ in RANGE Array OUT[1]"=w213:bool, "XYZ in RANGE Array OUT[2]"=w212:bool, "XYZ in RANGE Array OUT[3]"=w211:bool)  [unwired: 5 out]
      n160 = Unbundle(w227) -> ("XYZR VEL PV Array OUT[0]"=w198:i32, "XYZR VEL PV Array OUT[1]"=w197:i32, "XYZR VEL PV Array OUT[2]"=w196:i32, "XYZR VEL PV Array OUT[3]"=w195:i32)  [unwired: 5 out]
      n161 = Unbundle(w226) -> ("XYZR MAX MIN POS[0]"=w210:i32, "XYZR MAX MIN POS[1]"=w209:i32, "XYZR MAX MIN POS[2]"=w208:i32, "XYZR MAX MIN POS[3]"=w207:i32, "XYZR MAX MIN POS[4]"=w206:i32, "XYZR MAX MIN POS[5]"=w205:i32, "XYZR MAX MIN POS[6]"=w204:i32, "XYZR MAX MIN POS[7]"=w203:i32)  [unwired: 1 out]
      n162 = Unbundle(w230) -> ("Error Array OUT[0]"=w221:errorcluster, "Error Array OUT[1]"=w220:errorcluster, "Error Array OUT[2]"=w219:errorcluster, "Error Array OUT[3]"=w218:errorcluster)  [unwired: 5 out]
      n163 = Initialize Array(w183, w183, 4 ("dimension size")) -> (w193:i32[][])
      n164 = property on="X velocity PV step/sec" class="DigNum (strict)"("Val(Sgnl)"=w198) -> ()  [unwired: 2 in, 2 out]
      n165 = property on="Y velocity PV step/sec" class="DigNum (strict)"("Val(Sgnl)"=w197) -> ()  [unwired: 2 in, 2 out]
      n166 = property on="Z  velocity PV step/sec" class="DigNum (strict)"("Val(Sgnl)"=w196) -> ()  [unwired: 2 in, 2 out]
      n167 = property on="R velocity PV step/sec" class="DigNum (strict)"("Val(Sgnl)"=w195) -> ()  [unwired: 2 in, 2 out]
      n168 = property on="X Step SP" class="DigNum (strict)"("Val(Sgnl)"=w199) -> ()  [unwired: 2 in, 2 out]
      n169 = property on="Y Step SP" class="DigNum (strict)"("Val(Sgnl)"=w200) -> ()  [unwired: 2 in, 2 out]
      n170 = property on="Z Step SP" class="DigNum (strict)"("Val(Sgnl)"=w201) -> ()  [unwired: 2 in, 2 out]
      n171 = property on="R Step SP" class="DigNum (strict)"("Val(Sgnl)"=w202) -> ()  [unwired: 2 in, 2 out]
      n172 = property on="X Position SP mm" class="DigNum (strict)"("Val(Sgnl)"=w161) -> ()  [unwired: 2 in, 2 out]
      n173 = property on="X Position mm PV" class="DigNum (strict)"("Val(Sgnl)"=w161) -> ()  [unwired: 2 in, 2 out]
      n174 = property on="Y Position SP mm" class="DigNum (strict)"("Val(Sgnl)"=w162) -> ()  [unwired: 2 in, 2 out]
      n175 = property on="Y Position mm PV" class="DigNum (strict)"("Val(Sgnl)"=w162) -> ()  [unwired: 2 in, 2 out]
      n176 = property on="Z Position SP mm" class="DigNum (strict)"("Val(Sgnl)"=w163) -> ()  [unwired: 2 in, 2 out]
      n177 = property on="Z Position mm PV" class="DigNum (strict)"("Val(Sgnl)"=w163) -> ()  [unwired: 2 in, 2 out]
      n178 = property on="R Position SP deg" class="DigNum (strict)"("Val(Sgnl)"=w164) -> ()  [unwired: 2 in, 2 out]
      n179 = property on="R Position deg PV" class="DigNum (strict)"("Val(Sgnl)"=w164) -> ()  [unwired: 2 in, 2 out]
      n180 = property on="X  in Range" class="Bool (strict)"("Val(Sgnl)"=w214) -> ()  [unwired: 2 in, 2 out]
      n181 = property on="Y in Range" class="Bool (strict)"("Val(Sgnl)"=w213) -> ()  [unwired: 2 in, 2 out]
      n182 = property on="Z in Range" class="Bool (strict)"("Val(Sgnl)"=w212) -> ()  [unwired: 2 in, 2 out]
      n183 = property on="R in Range" class="Bool (strict)"("Val(Sgnl)"=w211) -> ()  [unwired: 2 in, 2 out]
      n184 = Build Array (concatenate)(w193, w188) -> (→"Presets":i32[][])
      n185 = property on="X MAXPOS" class="DigNum (strict)"("Val(Sgnl)"=w210) -> ()  [unwired: 2 in, 2 out]
      n186 = property on="X MINPOS" class="DigNum (strict)"("Val(Sgnl)"=w209) -> ()  [unwired: 2 in, 2 out]
      n187 = property on="Y MAXPOS" class="DigNum (strict)"("Val(Sgnl)"=w208) -> ()  [unwired: 2 in, 2 out]
      n188 = property on="Y MINPOS" class="DigNum (strict)"("Val(Sgnl)"=w207) -> ()  [unwired: 2 in, 2 out]
      n189 = property on="Z MAXPOS" class="DigNum (strict)"("Val(Sgnl)"=w206) -> ()  [unwired: 2 in, 2 out]
      n190 = property on="Z MINPOS" class="DigNum (strict)"("Val(Sgnl)"=w205) -> ()  [unwired: 2 in, 2 out]
      n191 = property on="R MAXPOS" class="DigNum (strict)"("Val(Sgnl)"=w204) -> ()  [unwired: 2 in, 2 out]
      n192 = property on="R MINPOS" class="DigNum (strict)"("Val(Sgnl)"=w203) -> ()  [unwired: 2 in, 2 out]
      "X COM PORT" <- w248
      "Z COM PORT" <- w247
      "Y COM PORT" <- w246
      "R COM PORT" <- w245
    }
  }
  n193 = property on="Z Step SP" class="DigNum (strict)"("Maximum"=102400000.0 ("upper limit")) -> ()  [unwired: 2 in, 2 out]
  n194 = property on="Z Step SP" class="DigNum (strict)"("Minimum"=0.0 ("lower limit")) -> ()  [unwired: 2 in, 2 out]
  n195 = property on="R Step SP" class="DigNum (strict)"("Maximum"=0.0 ("Data Entry Limits:Maximum")) -> ()  [unwired: 2 in, 2 out]
  n196 = property on="R Step SP" class="DigNum (strict)"("Minimum"=-6144000.0 ("Data Entry Limits:Minimum")) -> ()  [unwired: 2 in, 2 out]
  n197 = while {
    tunnel: [w278] -> w40
    tunnel: [w281] -> w41
    tunnel: [w284] -> w49
    tunnel: [w277] -> w48
    tunnel: [w283] -> w43
    tunnel: [w282] -> w42
    tunnel: [w280] -> w39
    tunnel: [w279] -> w38
    tunnel: w13 -> [w300]
    tunnel: w12 -> [w298]
    tunnel: w11 -> [w296]
    tunnel: w10 -> [w294]
    tunnel: w9 -> [w299]
    tunnel: w8 -> [w297]
    tunnel: w7 -> [w295]
    tunnel: w6 -> [w293]
    tunnel: w5 -> [w274]
    tunnel: w4 -> [w273]
    shift-right: [w267] -> _
    shift-left: dbl[] [] -> [w265]
    shift-right: [w266] -> _
    shift-left: dbl[] [] -> [w264]
    stop <- w275 stop-if-true
    n198 = event shown="[0] Timeout" {
      selector: _ -> [_ _ _ _ _ _ _ _ _ _ _ _ _ _ _ _ _]
      dyn-events: _ -> [_ _ _ _ _ _ _ _ _ _ _ _ _ _ _ _ _]
      timeout: 100 -> [_ _ _ _ _ _ _ _ _ _ _ _ _ _ _ _ _]
      tunnel: [w524 w1261 w1297 w1614 w1740 w1784 w1862 w1952 w1981 w2009 w2039 w2068 w2192 w2363 w2433 w2667 w2716] -> w290
      tunnel: [w525 w1256 w1298 w1615 w1737 w1781 w1859 w1949 w1978 w2007 w2036 w2065 w2189 w2364 w2434 w2668 w2717] -> w289
      tunnel: [w543 w1258 w1306 w1605 w1735 w1779 w1857 w1947 w1976 w2005 w2034 w2063 w2216 w2357 w2426 w2672 w2711] -> w286
      tunnel: [w542 w1263 w1305 w1604 w1742 w1786 w1864 w1954 w1983 w2012 w2041 w2070 w2215 w2356 w2424 w2671 w2710] -> w285
      tunnel: [w527 w1257 w1302 w1603 w1736 w1780 w1858 w1948 w1977 w2006 w2035 w2064 w2176 w2353 w2432 w2670 w2715] -> w287
      tunnel: [w526 w1262 w1301 w1602 w1741 w1785 w1863 w1953 w1982 w2011 w2040 w2069 w2175 w2352 w2431 w2669 w2714] -> w288
      tunnel: [w521 w1259 w1294 w1613 w1738 w1782 w1860 w1950 w1979 w2008 w2037 w2066 w2162 w2349 w2429 w2666 w2713] -> w292
      tunnel: [w520 w1260 w1293 w1612 w1739 w1783 w1861 w1951 w1980 w2010 w2038 w2067 w2161 w2348 w2428 w2665 w2712] -> w291
      tunnel: w300 -> [w519 w1258 w1308 w1608 w1735 w1779 w1857 w1947 w1976 w2005 w2034 w2063 w2211 w2347 w2422 w2660 w2708]
      tunnel: w299 -> [w518 w1263 w1307 w1633 w1742 w1786 w1864 w1954 w1983 w2012 w2041 w2070 w2212 w2345 w2421 w2664 w2702]
      tunnel: w298 -> [w517 w1257 w1303 w1611 w1736 w1780 w1858 w1948 w1977 w2006 w2035 w2064 w2177 w2346 w2420 w2659 w2709]
      tunnel: w297 -> [w516 w1262 w1304 w1632 w1741 w1785 w1863 w1953 w1982 w2011 w2040 w2069 w2178 w2344 w2419 w2663 w2703]
      tunnel: w296 -> [w515 w1256 w1299 w1618 w1737 w1781 w1859 w1949 w1978 w2007 w2036 w2065 w2190 w2343 w2418 w2658 w2706]
      tunnel: w295 -> [w514 w1261 w1300 w1631 w1740 w1784 w1862 w1952 w1981 w2009 w2039 w2068 w2191 w2341 w2417 w2662 w2704]
      tunnel: w294 -> [w513 w1259 w1295 w1621 w1738 w1782 w1860 w1950 w1979 w2008 w2037 w2066 w2163 w2342 w2416 w2657 w2707]
      tunnel: w293 -> [w512 w1260 w1296 w1630 w1739 w1783 w1861 w1951 w1980 w2010 w2038 w2067 w2164 w2340 w2415 w2661 w2705]
      tunnel: [w495 _ _ _ _ _ _ _ _ _ _ _ _ _ _ _ _] -> w267
      tunnel: [w493 _ _ _ _ _ _ _ _ _ _ _ _ _ _ _ _] -> w266
      tunnel: w265 -> [w498 _ _ _ _ _ _ _ _ _ _ _ _ _ _ _ _]
      tunnel: w264 -> [w497 _ _ _ _ _ _ _ _ _ _ _ _ _ _ _ _]
      event #0 {
        n199 = event-data() -> ()  [unwired: 1 in, 2 out]
        n200 = property on="GO" class="Bool"() -> ("DisabledEnum"=w511:T1)  [unwired: 2 in, 2 out]
        n201 = property on="GO" class="Bool"() -> ("DisabledEnum"=w508:T1)  [unwired: 2 in, 2 out]
        n202 = property on="Scan Go" class="Bool (strict)"() -> ("DisabledEnum"=w505:T1)  [unwired: 2 in, 2 out]
        n203 = Equal?(x=w511, y=T1."Disabled and Grayed Out") -> (x = y?=w509:bool)
        n204 = case shown="True" w509 {
          tunnel: [w566 w613] -> w543
          tunnel: [w565 w612] -> w542
          tunnel: [w564 w611] -> w527
          tunnel: [w563 w610] -> w526
          tunnel: [w562 w609] -> w525
          tunnel: [w561 w608] -> w524
          tunnel: [w560 w607] -> w521
          tunnel: [w559 w606] -> w520
          tunnel: w519 -> [w574 w605]
          tunnel: w518 -> [w573 w604]
          tunnel: w517 -> [w572 w603]
          tunnel: w516 -> [w571 w602]
          tunnel: w515 -> [w570 w601]
          tunnel: w514 -> [w569 w600]
          tunnel: w513 -> [w568 w599]
          tunnel: w512 -> [w567 w598]
          frame #0 {
            n205 = call "DigitalIO_sub_V1_MON.vi"() -> ("CL"=w553:bool, "OP"=w554:bool)  [unwired: 8 in]
            n206 = property on="CL" class="Bool (strict)"("Val(Sgnl)"=w553) -> ()  [unwired: 2 in, 2 out]
            n207 = property on="OP" class="Bool (strict)"("Val(Sgnl)"=w554) -> ()  [unwired: 2 in, 2 out]
            n208 = call "mdrive send command.vi"("error in (no error)"=w567, "Extra"="MV", "Command"=T10."Print Parameter", "VISA resource name"=w568) -> ("error out"=w559:errorcluster, "read buffer"=w576:string, "VISA resource name out"=w560:refnum<visa-resource-name>)  [unwired: 3 in]
            n209 = call "mdrive send command.vi"("error in (no error)"=w569, "Extra"="MV", "Command"=T10."Print Parameter", "VISA resource name"=w570) -> ("error out"=w561:errorcluster, "read buffer"=w580:string, "VISA resource name out"=w562:refnum<visa-resource-name>)  [unwired: 3 in]
            n210 = call "mdrive send command.vi"("error in (no error)"=w571, "Extra"="MV", "Command"=T10."Print Parameter", "VISA resource name"=w572) -> ("error out"=w563:errorcluster, "read buffer"=w584:string, "VISA resource name out"=w564:refnum<visa-resource-name>)  [unwired: 3 in]
            n211 = call "mdrive send command.vi"("error in (no error)"=w573, "Extra"="MV", "Command"=T10."Print Parameter", "VISA resource name"=w574) -> ("error out"=w565:errorcluster, "read buffer"=w588:string, "VISA resource name out"=w566:refnum<visa-resource-name>)  [unwired: 3 in]
            n212 = Not Equal?(x=w576, y="") -> (x != y?=w555:bool)
            n213 = Not Equal?(x=w580, y="") -> (x != y?=w556:bool)
            n214 = Not Equal?(x=w584, y="") -> (x != y?=w557:bool)
            n215 = Not Equal?(x=w588, y="") -> (x != y?=w558:bool)
            n216 = property on="R Ready" class="Bool (strict)"("Val(Sgnl)"=w555) -> ()  [unwired: 2 in, 2 out]
            n217 = property on="Z Ready" class="Bool (strict)"("Val(Sgnl)"=w557) -> ()  [unwired: 2 in, 2 out]
            n218 = property on="Y Ready" class="Bool (strict)"("Val(Sgnl)"=w556) -> ()  [unwired: 2 in, 2 out]
            n219 = property on="X Ready" class="Bool (strict)"("Val(Sgnl)"=w558) -> ()  [unwired: 2 in, 2 out]
          }
          frame #1 {
            n220 = flat-sequence {
              tunnel: [w992] -> w655
              tunnel: [w983] -> w654
              tunnel: [w982] -> w653
              tunnel: w603 -> [w986]
              tunnel: w602 -> [w985]
              tunnel: [w1024] -> w652
              tunnel: [w1023] -> w651
              tunnel: [w1022] -> w650
              tunnel: [w1015] -> w649
              tunnel: w655 -> [w1022]
              tunnel: w654 -> [w1021]
              tunnel: w653 -> [w1020]
              tunnel: w652 -> [w1034]
              tunnel: [w1034] -> w648
              tunnel: w651 -> [w1033]
              tunnel: [w1033] -> w647
              tunnel: w650 -> [w1032]
              tunnel: [w1032] -> w646
              tunnel: w649 -> [w1031]
              tunnel: [w1031] -> w645
              tunnel: [w1038] -> w644
              tunnel: [w1039] -> w643
              tunnel: [w1035] -> w642
              tunnel: w645 -> [w1035]
              tunnel: w646 -> [w1036]
              tunnel: w647 -> [w1040]
              tunnel: w648 -> [w1037]
              tunnel: w644 -> [w1051]
              tunnel: w643 -> [w1052]
              tunnel: w642 -> [w1054]
              tunnel: [w1050] -> w610
              tunnel: [w1049] -> w611
              frame #0 {
                n221 = call "mdrive send command.vi"("error in (no error)"=w985, "Extra"="P", "Command"=T10."Print Parameter", "VISA resource name"=w986) -> ("error out"=w982:errorcluster, "read buffer"=w1002:string, "VISA resource name out"=w983:refnum<visa-resource-name>)  [unwired: 3 in]
                n222 = property on="Z steps/rev" class="DigNum (strict)"() -> ("Value"=w991:u32)  [unwired: 2 in, 2 out]
                n223 = To Double Precision Float(number=w991) -> (double precision float=w998:dbl)
                n224 = Decimal String To Number(string=w1002, offset=0) -> (number=w981:i32)  [unwired: 1 in, 1 out]
                n225 = To Double Precision Float(number=w981) -> (double precision float=w996:dbl)
                n226 = Divide(x=w996, y=w998) -> (x/y=w997:dbl)
                n227 = property on="Z Step PV" class="DigNum (strict)"("Val(Sgnl)"=w981) -> ()  [unwired: 2 in, 2 out]
                n228 = property on="Z mm/rev" class="DigNum (strict)"() -> ("Value"=w990:dbl)  [unwired: 2 in, 2 out]
                n229 = property on="Z Step SP" class="DigNum (strict)"() -> ("Maximum"=w993:dbl)  [unwired: 2 in, 2 out]
                n230 = property on="Z Step SP" class="DigNum (strict)"() -> ("Minimum"=w987:dbl)  [unwired: 2 in, 2 out]
                n231 = Multiply(x=w997, y=w990) -> (x*y=w984:dbl)
                n232 = To Long Integer(number=w993) -> (32bit integer=w999:i32)
                n233 = To Long Integer(number=w987) -> (32bit integer=w1000:i32)
                n234 = property on="Z offset mm" class="DigNum (strict)"() -> ("Value"=w989:dbl)  [unwired: 2 in, 2 out]
                n235 = In Range and Coerce(upper limit=w999, x=w981, lower limit=w1000) -> (In Range?=w992:bool)  [unwired: 1 out]
                n236 = Add(x=w984, y=w989) -> (x+y=w988:dbl)
                n237 = property on="Z Position mm PV" class="DigNum (strict)"("Val(Sgnl)"=w988) -> ()  [unwired: 2 in, 2 out]
                n238 = property on="Z in Range" class="Bool (strict)"("Val(Sgnl)"=w992) -> ()  [unwired: 2 in, 2 out]
                n239 = property on="OK Button" class="Bool (strict)"() -> ("Value"=w978:bool)  [unwired: 2 in, 2 out]
                n240 = Not Equal?(x=w978, y=TRUE) -> (x != y?=w976:bool)
                n241 = Equal?(x=w981, y=15360000) -> (x = y?=w975:bool)
                n242 = And(x=w975, y=w976) -> (x .and. y?=w974:bool)
                n243 = case shown="True" w974 {
                  tunnel: [FALSE ("true") w1013] -> w979
                  frame #0 {
                  }
                  frame #1 {
                    n244 = One Button Dialog(message="HAVE YOU OPEND THE VALVE???\nTHEN REWRITE YOUR POSITION\n AND PRESS GO!") -> (true=w1013:bool)  [unwired: 1 in]
                  }
                }
                n245 = case shown="True" w979 {
                  frame #0 {
                    n246 = call "DigitalIO_sub_V1_MON.vi"() -> ("CL"=w1003:bool, "OP"=w1004:bool)  [unwired: 8 in]
                    n247 = property on="OP" class="Bool (strict)"("Val(Sgnl)"=w1004) -> ()  [unwired: 2 in, 2 out]
                    n248 = property on="CL" class="Bool (strict)"("Val(Sgnl)"=w1003) -> ()  [unwired: 2 in, 2 out]
                  }
                  frame #1 {
                    n249 = while {
                      stop <- w1011 stop-if-true
                      n250 = property on="OK Button" class="Bool (strict)"() -> ("Value"=w1005:bool)  [unwired: 2 in, 2 out]
                      n251 = call "ValveConrtoller.vi"("OK Button"=w1005) -> ("OUTGOING SIGNAL"=w1006:bool, "CL"=w1007:bool, "OP"=w1008:bool, "VALVE\nopend/closed"=w1009:bool)  [unwired: 3 in]
                      n252 = property on="Valve \nopend/closed" class="Bool (strict)"("Val(Sgnl)"=w1009) -> ()  [unwired: 2 in, 2 out]
                      n253 = property on="CL" class="Bool (strict)"("Val(Sgnl)"=w1007) -> ()  [unwired: 2 in, 2 out]
                      n254 = Equal?(x=w1006, y=TRUE) -> (x = y?=w1011:bool)
                      n255 = property on="OP" class="Bool (strict)"("Val(Sgnl)"=w1008) -> ()  [unwired: 2 in, 2 out]
                    }
                  }
                }
              }
              frame #1 {
                n256 = call "mdrive send command.vi"("error in (no error)"=w1020, "Extra"="MV", "Command"=T10."Print Parameter", "VISA resource name"=w1021) -> ("error out"=w1023:errorcluster, "read buffer"=w1026:string, "VISA resource name out"=w1024:refnum<visa-resource-name>)  [unwired: 3 in]
                n257 = Not Equal?(x=w1026, y="") -> (x != y?=w1019:bool)
                n258 = Decimal String To Number(string=w1026, offset=0 ("offset (0)")) -> (number=w1016:i32)  [unwired: 1 in, 1 out]
                n259 = property on="Z Ready" class="Bool (strict)"("Val(Sgnl)"=w1019) -> ()  [unwired: 2 in, 2 out]
                n260 = Number To Boolean Array(number=w1016) -> (Boolean array=w1018:bool[])
                n261 = Index Array(array=w1018, index=0) -> (element=w1015:bool)
                n262 = property on="Z in Motion" class="Bool (strict)"("Val(Sgnl)"=w1015) -> ()  [unwired: 2 in, 2 out]
              }
              frame #2 {
                n263 = Wait (ms)(milliseconds to wait=u32 50) -> ()  [unwired: 1 out]
              }
              frame #3 {
                n264 = case shown="False" w1036 {
                  tunnel: w1037 -> [w1043 w1047]
                  tunnel: [w1044 w1047] -> w1038
                  tunnel: [w1045 w1046] -> w1039
                  tunnel: w1040 -> [w1042 w1046]
                  frame #0 {
                    n265 = call "mdrive send command.vi"("error in (no error)"=w1042, "Command"=T10."Stop", "VISA resource name"=w1043) -> ("error out"=w1045:errorcluster, "VISA resource name out"=w1044:refnum<visa-resource-name>)  [unwired: 4 in, 1 out]
                  }
                  frame #1 {
                  }
                }
              }
              frame #4 {
                n266 = property on="Z Backlash corr" class="Bool (strict)"() -> ("Value"=w1048:bool)  [unwired: 2 in, 2 out]
                n267 = Implies(1:w1054, 2:w1048) -> (0:w1053:bool)
                n268 = case shown="False" w1053 {
                  tunnel: w1052 -> [w1062 w1119]
                  tunnel: w1051 -> [w1061 w1120]
                  tunnel: [w1056 w1119] -> w1050
                  tunnel: [w1060 w1120] -> w1049
                  frame #0 {
                    # "Backlash"
                    n269 = flat-sequence {
                      tunnel: [w1075] -> w1074
                      tunnel: [w1079] -> w1073
                      tunnel: [w1078] -> w1072
                      tunnel: w1062 -> [w1077]
                      tunnel: w1061 -> [w1076]
                      tunnel: w1074 -> [w1087]
                      tunnel: [w1087] -> w1071
                      tunnel: w1073 -> [w1086]
                      tunnel: w1072 -> [w1085]
                      tunnel: [w1084] -> w1070
                      tunnel: [w1083] -> w1069
                      tunnel: [w1082] -> w1059
                      tunnel: w1071 -> [w1101]
                      tunnel: w1070 -> [w1092]
                      tunnel: w1069 -> [w1100]
                      tunnel: [w1092] -> w1068
                      tunnel: [w1100] -> w1067
                      tunnel: [w1091] -> w1064
                      tunnel: [w1099] -> w1063
                      tunnel: w1059 -> [w1099]
                      tunnel: w1068 -> [w1104]
                      tunnel: w1067 -> [w1105]
                      tunnel: [w1103] -> w1066
                      tunnel: [w1111] -> w1065
                      tunnel: w1064 -> [w1111]
                      tunnel: w1063 -> [w1107]
                      tunnel: [w1106] -> w1057
                      tunnel: w1066 -> [w1114]
                      tunnel: w1065 -> [w1113]
                      tunnel: [w1115] -> w1058
                      tunnel: w1057 -> [w1115]
                      tunnel: [w1114] -> w1055
                      tunnel: [w1118] -> w1060
                      tunnel: w1058 -> [w1118]
                      tunnel: [w1117] -> w1056
                      tunnel: w1055 -> [w1117]
                      frame #0 {
                        n270 = property on="Z Backlash steps/sec" class="DigNum (strict)"() -> ("Value"=w1075:i32)  [unwired: 2 in, 2 out]
                        n271 = Number To Decimal String(number=w1075) -> (decimal integer string=w1080:string)  [unwired: 1 in]
                        n272 = call "mdrive send command.vi"("error in (no error)"=w1077, "Extra"=w1080, "Command"=T10."Max Velocity", "VISA resource name"=w1076) -> ("error out"=w1078:errorcluster, "VISA resource name out"=w1079:refnum<visa-resource-name>)  [unwired: 3 in, 1 out]
                      }
                      frame #1 {
                        n273 = property on="Z Backlash" class="DigNum (strict)"() -> ("Value"=w1082:i32)  [unwired: 2 in, 2 out]
                        n274 = Number To Decimal String(number=w1082) -> (decimal integer string=w1088:string)  [unwired: 1 in]
                        n275 = call "mdrive send command.vi"("error in (no error)"=w1085, "Extra"=w1088, "Command"=T10."Move to Relative Position", "VISA resource name"=w1086) -> ("error out"=w1084:errorcluster, "VISA resource name out"=w1083:refnum<visa-resource-name>)  [unwired: 3 in, 1 out]
                      }
                      frame #2 {
                        n276 = To Double Precision Float(number=w1099) -> (double precision float=w1097:dbl)
                        n277 = To Double Precision Float(number=w1101) -> (double precision float=w1102:dbl)
                        n278 = Absolute Value(x=w1097) -> (abs(x)=w1098:dbl)
                        n279 = Divide(x=w1098, y=w1102) -> (x/y=w1095:dbl)
                        n280 = Multiply(x=1000.0, y=w1095) -> (x*y=w1093:dbl)
                        n281 = Add(x=w1093, y=300.0) -> (x+y=w1091:dbl)
                        n282 = To Unsigned Long Integer(number=w1091) -> (unsigned 32bit integer=w1090:u32)
                        n283 = Wait (ms)(milliseconds to wait=w1090) -> ()  [unwired: 1 out]
                      }
                      frame #3 {
                        n284 = Negate(x=w1107) -> (-x=w1108:i32)
                        n285 = Number To Decimal String(number=w1108) -> (decimal integer string=w1109:string)  [unwired: 1 in]
                        n286 = call "mdrive send command.vi"("error in (no error)"=w1104, "Extra"=w1109, "Command"=T10."Move to Relative Position", "VISA resource name"=w1105) -> ("error out"=w1103:errorcluster, "VISA resource name out"=w1106:refnum<visa-resource-name>)  [unwired: 3 in, 1 out]
                      }
                      frame #4 {
                        n287 = To Unsigned Long Integer(number=w1113) -> (unsigned 32bit integer=w1112:u32)
                        n288 = Wait (ms)(milliseconds to wait=w1112) -> ()  [unwired: 1 out]
                      }
                      frame #5 {
                        n289 = property on="Z Backlash corr" class="Bool (strict)"("Val(Sgnl)"=FALSE ("Value (Signaling)")) -> ()  [unwired: 2 in, 2 out]
                      }
                    }
                  }
                  frame #1 {
                  }
                }
              }
            }
            n290 = flat-sequence {
              tunnel: [w855] -> w641
              tunnel: [w857] -> w640
              tunnel: [w856] -> w639
              tunnel: w601 -> [w848]
              tunnel: w600 -> [w847]
              tunnel: [w877] -> w638
              tunnel: [w876] -> w637
              tunnel: [w875] -> w636
              tunnel: [w868] -> w635
              tunnel: w641 -> [w875]
              tunnel: w640 -> [w874]
              tunnel: w639 -> [w873]
              tunnel: w638 -> [w887]
              tunnel: [w887] -> w634
              tunnel: w637 -> [w886]
              tunnel: [w886] -> w633
              tunnel: w636 -> [w885]
              tunnel: [w885] -> w632
              tunnel: w635 -> [w884]
              tunnel: [w884] -> w631
              tunnel: [w891] -> w630
              tunnel: [w892] -> w629
              tunnel: [w888] -> w628
              tunnel: w631 -> [w888]
              tunnel: w632 -> [w889]
              tunnel: w633 -> [w893]
              tunnel: w634 -> [w890]
              tunnel: w630 -> [w904]
              tunnel: w629 -> [w905]
              tunnel: w628 -> [w907]
              tunnel: [w903] -> w608
              tunnel: [w902] -> w609
              frame #0 {
                n291 = call "mdrive send command.vi"("error in (no error)"=w847, "Extra"="P", "Command"=T10."Print Parameter", "VISA resource name"=w848) -> ("error out"=w856:errorcluster, "read buffer"=w867:string, "VISA resource name out"=w857:refnum<visa-resource-name>)  [unwired: 3 in]
                n292 = property on="Y steps/rev" class="DigNum (strict)"() -> ("Value"=w851:u32)  [unwired: 2 in, 2 out]
                n293 = Decimal String To Number(string=w867, offset=0) -> (number=w846:i32)  [unwired: 1 in, 1 out]
                n294 = To Double Precision Float(number=w851) -> (double precision float=w863:dbl)
                n295 = To Double Precision Float(number=w846) -> (double precision float=w860:dbl)
                n296 = property on="Y Step PV" class="DigNum (strict)"("Val(Sgnl)"=w846) -> ()  [unwired: 2 in, 2 out]
                n297 = Divide(x=w860, y=w863) -> (x/y=w862:dbl)
                n298 = property on="Y Step SP" class="DigNum (strict)"() -> ("Maximum"=w850:dbl)  [unwired: 2 in, 2 out]
                n299 = property on="Y Step SP" class="DigNum (strict)"() -> ("Minimum"=w849:dbl)  [unwired: 2 in, 2 out]
                n300 = property on="Y mm/rev" class="DigNum (strict)"() -> ("Value"=w852:dbl)  [unwired: 2 in, 2 out]
                n301 = To Long Integer(number=w850) -> (32bit integer=w864:i32)
                n302 = To Long Integer(number=w849) -> (32bit integer=w865:i32)
                n303 = Multiply(x=w862, y=w852) -> (x*y=w861:dbl)
                n304 = In Range and Coerce(upper limit=w864, x=w846, lower limit=w865) -> (In Range?=w855:bool)  [unwired: 1 out]
                n305 = property on="Y offset mm" class="DigNum (strict)"() -> ("Value"=w853:dbl)  [unwired: 2 in, 2 out]
                n306 = Add(x=w861, y=w853) -> (x+y=w854:dbl)
                n307 = property on="Y in Range" class="Bool (strict)"("Val(Sgnl)"=w855) -> ()  [unwired: 2 in, 2 out]
                n308 = property on="Y Position mm PV" class="DigNum (strict)"("Val(Sgnl)"=w854) -> ()  [unwired: 2 in, 2 out]
              }
              frame #1 {
                n309 = call "mdrive send command.vi"("error in (no error)"=w873, "Extra"="MV", "Command"=T10."Print Parameter", "VISA resource name"=w874) -> ("error out"=w876:errorcluster, "read buffer"=w879:string, "VISA resource name out"=w877:refnum<visa-resource-name>)  [unwired: 3 in]
                n310 = Not Equal?(x=w879, y="") -> (x != y?=w872:bool)
                n311 = Decimal String To Number(string=w879, offset=0 ("offset (0)")) -> (number=w869:i32)  [unwired: 1 in, 1 out]
                n312 = property on="Y Ready" class="Bool (strict)"("Val(Sgnl)"=w872) -> ()  [unwired: 2 in, 2 out]
                n313 = Number To Boolean Array(number=w869) -> (Boolean array=w871:bool[])
                n314 = Index Array(array=w871, index=0) -> (element=w868:bool)
                n315 = property on="Y in Motion" class="Bool (strict)"("Val(Sgnl)"=w868) -> ()  [unwired: 2 in, 2 out]
              }
              frame #2 {
                n316 = Wait (ms)(milliseconds to wait=u32 50) -> ()  [unwired: 1 out]
              }
              frame #3 {
                n317 = case shown="True" w889 {
                  tunnel: w890 -> [w896 w899]
                  tunnel: [w897 w899] -> w891
                  tunnel: [w898 w900] -> w892
                  tunnel: w893 -> [w895 w900]
                  frame #0 {
                    n318 = call "mdrive send command.vi"("error in (no error)"=w895, "Command"=T10."Stop", "VISA resource name"=w896) -> ("error out"=w898:errorcluster, "VISA resource name out"=w897:refnum<visa-resource-name>)  [unwired: 4 in, 1 out]
                  }
                  frame #1 {
                  }
                }
              }
              frame #4 {
                n319 = property on="Y Backlash corr" class="Bool (strict)"() -> ("Value"=w901:bool)  [unwired: 2 in, 2 out]
                n320 = Implies(1:w907, 2:w901) -> (0:w906:bool)
                n321 = case shown="False" w906 {
                  tunnel: w905 -> [w915 w972]
                  tunnel: w904 -> [w914 w973]
                  tunnel: [w909 w972] -> w903
                  tunnel: [w913 w973] -> w902
                  frame #0 {
                    # "Backlash"
                    n322 = flat-sequence {
                      tunnel: [w928] -> w927
                      tunnel: [w932] -> w926
                      tunnel: [w931] -> w925
                      tunnel: w915 -> [w930]
                      tunnel: w914 -> [w929]
                      tunnel: w927 -> [w940]
                      tunnel: [w940] -> w924
                      tunnel: w926 -> [w939]
                      tunnel: w925 -> [w938]
                      tunnel: [w937] -> w923
                      tunnel: [w936] -> w922
                      tunnel: [w935] -> w912
                      tunnel: w924 -> [w954]
                      tunnel: w923 -> [w945]
                      tunnel: w922 -> [w953]
                      tunnel: [w945] -> w921
                      tunnel: [w953] -> w920
                      tunnel: [w944] -> w917
                      tunnel: [w952] -> w916
                      tunnel: w912 -> [w952]
                      tunnel: w921 -> [w957]
                      tunnel: w920 -> [w958]
                      tunnel: [w956] -> w919
                      tunnel: [w964] -> w918
                      tunnel: w917 -> [w964]
                      tunnel: w916 -> [w960]
                      tunnel: [w959] -> w910
                      tunnel: w919 -> [w967]
                      tunnel: w918 -> [w966]
                      tunnel: [w968] -> w911
                      tunnel: w910 -> [w968]
                      tunnel: [w967] -> w908
                      tunnel: [w971] -> w913
                      tunnel: w911 -> [w971]
                      tunnel: [w970] -> w909
                      tunnel: w908 -> [w970]
                      frame #0 {
                        n323 = property on="Y Backlash steps/sec" class="DigNum (strict)"() -> ("Value"=w928:i32)  [unwired: 2 in, 2 out]
                        n324 = Number To Decimal String(number=w928) -> (decimal integer string=w933:string)  [unwired: 1 in]
                        n325 = call "mdrive send command.vi"("error in (no error)"=w930, "Extra"=w933, "Command"=T10."Max Velocity", "VISA resource name"=w929) -> ("error out"=w931:errorcluster, "VISA resource name out"=w932:refnum<visa-resource-name>)  [unwired: 3 in, 1 out]
                      }
                      frame #1 {
                        n326 = property on="Y Backlash" class="DigNum (strict)"() -> ("Value"=w935:i32)  [unwired: 2 in, 2 out]
                        n327 = Number To Decimal String(number=w935) -> (decimal integer string=w941:string)  [unwired: 1 in]
                        n328 = call "mdrive send command.vi"("error in (no error)"=w938, "Extra"=w941, "Command"=T10."Move to Relative Position", "VISA resource name"=w939) -> ("error out"=w937:errorcluster, "VISA resource name out"=w936:refnum<visa-resource-name>)  [unwired: 3 in, 1 out]
                      }
                      frame #2 {
                        n329 = To Double Precision Float(number=w952) -> (double precision float=w950:dbl)
                        n330 = To Double Precision Float(number=w954) -> (double precision float=w955:dbl)
                        n331 = Absolute Value(x=w950) -> (abs(x)=w951:dbl)
                        n332 = Divide(x=w951, y=w955) -> (x/y=w948:dbl)
                        n333 = Multiply(x=1000.0, y=w948) -> (x*y=w946:dbl)
                        n334 = Add(x=w946, y=300.0) -> (x+y=w944:dbl)
                        n335 = To Unsigned Long Integer(number=w944) -> (unsigned 32bit integer=w943:u32)
                        n336 = Wait (ms)(milliseconds to wait=w943) -> ()  [unwired: 1 out]
                      }
                      frame #3 {
                        n337 = Negate(x=w960) -> (-x=w961:i32)
                        n338 = Number To Decimal String(number=w961) -> (decimal integer string=w962:string)  [unwired: 1 in]
                        n339 = call "mdrive send command.vi"("error in (no error)"=w957, "Extra"=w962, "Command"=T10."Move to Relative Position", "VISA resource name"=w958) -> ("error out"=w956:errorcluster, "VISA resource name out"=w959:refnum<visa-resource-name>)  [unwired: 3 in, 1 out]
                      }
                      frame #4 {
                        n340 = To Unsigned Long Integer(number=w966) -> (unsigned 32bit integer=w965:u32)
                        n341 = Wait (ms)(milliseconds to wait=w965) -> ()  [unwired: 1 out]
                      }
                      frame #5 {
                        n342 = property on="Y Backlash corr" class="Bool (strict)"("Val(Sgnl)"=FALSE ("Value (Signaling)")) -> ()  [unwired: 2 in, 2 out]
                      }
                    }
                  }
                  frame #1 {
                  }
                }
              }
            }
            n343 = flat-sequence {
              tunnel: [w727] -> w627
              tunnel: [w729] -> w626
              tunnel: [w728] -> w625
              tunnel: w599 -> [w720]
              tunnel: w598 -> [w719]
              tunnel: [w749] -> w624
              tunnel: [w748] -> w623
              tunnel: [w747] -> w622
              tunnel: [w740] -> w621
              tunnel: w627 -> [w747]
              tunnel: w626 -> [w746]
              tunnel: w625 -> [w745]
              tunnel: w624 -> [w759]
              tunnel: [w759] -> w620
              tunnel: w623 -> [w758]
              tunnel: [w758] -> w619
              tunnel: w622 -> [w757]
              tunnel: [w757] -> w618
              tunnel: w621 -> [w756]
              tunnel: [w756] -> w617
              tunnel: [w763] -> w616
              tunnel: [w764] -> w615
              tunnel: [w760] -> w614
              tunnel: w617 -> [w760]
              tunnel: w618 -> [w761]
              tunnel: w619 -> [w765]
              tunnel: w620 -> [w762]
              tunnel: w616 -> [w776]
              tunnel: w615 -> [w777]
              tunnel: w614 -> [w779]
              tunnel: [w775] -> w606
              tunnel: [w774] -> w607
              frame #0 {
                n344 = call "mdrive send command.vi"("error in (no error)"=w719, "Extra"="P", "Command"=T10."Print Parameter", "VISA resource name"=w720) -> ("error out"=w728:errorcluster, "read buffer"=w739:string, "VISA resource name out"=w729:refnum<visa-resource-name>)  [unwired: 3 in]
                n345 = property on="R steps/rev" class="DigNum (strict)"() -> ("Value"=w721:u32)  [unwired: 2 in, 2 out]
                n346 = Decimal String To Number(string=w739, offset=0) -> (number=w718:i32)  [unwired: 1 in, 1 out]
                n347 = To Double Precision Float(number=w721) -> (double precision float=w735:dbl)
                n348 = To Double Precision Float(number=w718) -> (double precision float=w732:dbl)
                n349 = property on="R Step PV" class="DigNum (strict)"("Val(Sgnl)"=w718) -> ()  [unwired: 2 in, 2 out]
                n350 = Divide(x=w732, y=w735) -> (x/y=w734:dbl)
                n351 = property on="R Step SP" class="DigNum (strict)"() -> ("Maximum"=w722:dbl)  [unwired: 2 in, 2 out]
                n352 = property on="R Step SP" class="DigNum (strict)"() -> ("Minimum"=w723:dbl)  [unwired: 2 in, 2 out]
                n353 = property on="R deg/rev" class="DigNum (strict)"() -> ("Value"=w724:dbl)  [unwired: 2 in, 2 out]
                n354 = Multiply(x=w734, y=w724) -> (x*y=w733:dbl)
                n355 = To Long Integer(number=w722) -> (32bit integer=w736:i32)
                n356 = To Long Integer(number=w723) -> (32bit integer=w737:i32)
                n357 = property on="R offset deg" class="DigNum (strict)"() -> ("Value"=w725:dbl)  [unwired: 2 in, 2 out]
                n358 = In Range and Coerce(upper limit=w736, x=w718, lower limit=w737) -> (In Range?=w727:bool)  [unwired: 1 out]
                n359 = Add(x=w733, y=w725) -> (x+y=w726:dbl)
                n360 = property on="R in Range" class="Bool (strict)"("Val(Sgnl)"=w727) -> ()  [unwired: 2 in, 2 out]
                n361 = property on="R Position deg PV" class="DigNum (strict)"("Val(Sgnl)"=w726) -> ()  [unwired: 2 in, 2 out]
              }
              frame #1 {
                n362 = call "mdrive send command.vi"("error in (no error)"=w745, "Extra"="MV", "Command"=T10."Print Parameter", "VISA resource name"=w746) -> ("error out"=w748:errorcluster, "read buffer"=w751:string, "VISA resource name out"=w749:refnum<visa-resource-name>)  [unwired: 3 in]
                n363 = Not Equal?(x=w751, y="") -> (x != y?=w744:bool)
                n364 = Decimal String To Number(string=w751, offset=0 ("offset (0)")) -> (number=w741:i32)  [unwired: 1 in, 1 out]
                n365 = Number To Boolean Array(number=w741) -> (Boolean array=w743:bool[])
                n366 = property on="R Ready" class="Bool (strict)"("Val(Sgnl)"=w744) -> ()  [unwired: 2 in, 2 out]
                n367 = Index Array(array=w743, index=0) -> (element=w740:bool)
                n368 = property on="R in Motion" class="Bool (strict)"("Val(Sgnl)"=w740) -> ()  [unwired: 2 in, 2 out]
              }
              frame #2 {
                n369 = Wait (ms)(milliseconds to wait=u32 50) -> ()  [unwired: 1 out]
              }
              frame #3 {
                n370 = case shown="True" w761 {
                  tunnel: w762 -> [w768 w772]
                  tunnel: [w769 w772] -> w763
                  tunnel: [w770 w771] -> w764
                  tunnel: w765 -> [w767 w771]
                  frame #0 {
                    n371 = call "mdrive send command.vi"("error in (no error)"=w767, "Command"=T10."Stop", "VISA resource name"=w768) -> ("error out"=w770:errorcluster, "VISA resource name out"=w769:refnum<visa-resource-name>)  [unwired: 4 in, 1 out]
                  }
                  frame #1 {
                  }
                }
              }
              frame #4 {
                n372 = property on="R Backlash corr" class="Bool (strict)"() -> ("Value"=w773:bool)  [unwired: 2 in, 2 out]
                n373 = Implies(1:w779, 2:w773) -> (0:w778:bool)
                n374 = case shown="False" w778 {
                  tunnel: w777 -> [w787 w844]
                  tunnel: w776 -> [w786 w845]
                  tunnel: [w781 w844] -> w775
                  tunnel: [w785 w845] -> w774
                  frame #0 {
                    # "Backlash"
                    n375 = flat-sequence {
                      tunnel: [w800] -> w799
                      tunnel: [w804] -> w798
                      tunnel: [w803] -> w797
                      tunnel: w787 -> [w802]
                      tunnel: w786 -> [w801]
                      tunnel: w799 -> [w812]
                      tunnel: [w812] -> w796
                      tunnel: w798 -> [w811]
                      tunnel: w797 -> [w810]
                      tunnel: [w809] -> w795
                      tunnel: [w808] -> w794
                      tunnel: [w807] -> w784
                      tunnel: w796 -> [w826]
                      tunnel: w795 -> [w817]
                      tunnel: w794 -> [w825]
                      tunnel: [w817] -> w793
                      tunnel: [w825] -> w792
                      tunnel: [w816] -> w789
                      tunnel: [w824] -> w788
                      tunnel: w784 -> [w824]
                      tunnel: w793 -> [w829]
                      tunnel: w792 -> [w830]
                      tunnel: [w828] -> w791
                      tunnel: [w836] -> w790
                      tunnel: w789 -> [w836]
                      tunnel: w788 -> [w832]
                      tunnel: [w831] -> w782
                      tunnel: w791 -> [w839]
                      tunnel: w790 -> [w838]
                      tunnel: [w840] -> w783
                      tunnel: w782 -> [w840]
                      tunnel: [w839] -> w780
                      tunnel: [w843] -> w785
                      tunnel: w783 -> [w843]
                      tunnel: [w842] -> w781
                      tunnel: w780 -> [w842]
                      frame #0 {
                        n376 = property on="R Backlash steps/sec" class="DigNum (strict)"() -> ("Value"=w800:i32)  [unwired: 2 in, 2 out]
                        n377 = Number To Decimal String(number=w800) -> (decimal integer string=w805:string)  [unwired: 1 in]
                        n378 = call "mdrive send command.vi"("error in (no error)"=w802, "Extra"=w805, "Command"=T10."Max Velocity", "VISA resource name"=w801) -> ("error out"=w803:errorcluster, "VISA resource name out"=w804:refnum<visa-resource-name>)  [unwired: 3 in, 1 out]
                      }
                      frame #1 {
                        n379 = property on="R Backlash" class="DigNum (strict)"() -> ("Value"=w807:i32)  [unwired: 2 in, 2 out]
                        n380 = Number To Decimal String(number=w807) -> (decimal integer string=w813:string)  [unwired: 1 in]
                        n381 = call "mdrive send command.vi"("error in (no error)"=w810, "Extra"=w813, "Command"=T10."Move to Relative Position", "VISA resource name"=w811) -> ("error out"=w809:errorcluster, "VISA resource name out"=w808:refnum<visa-resource-name>)  [unwired: 3 in, 1 out]
                      }
                      frame #2 {
                        n382 = To Double Precision Float(number=w824) -> (double precision float=w822:dbl)
                        n383 = To Double Precision Float(number=w826) -> (double precision float=w827:dbl)
                        n384 = Absolute Value(x=w822) -> (abs(x)=w823:dbl)
                        n385 = Divide(x=w823, y=w827) -> (x/y=w820:dbl)
                        n386 = Multiply(x=1000.0, y=w820) -> (x*y=w818:dbl)
                        n387 = Add(x=w818, y=300.0) -> (x+y=w816:dbl)
                        n388 = To Unsigned Long Integer(number=w816) -> (unsigned 32bit integer=w815:u32)
                        n389 = Wait (ms)(milliseconds to wait=w815) -> ()  [unwired: 1 out]
                      }
                      frame #3 {
                        n390 = Negate(x=w832) -> (-x=w833:i32)
                        n391 = Number To Decimal String(number=w833) -> (decimal integer string=w834:string)  [unwired: 1 in]
                        n392 = call "mdrive send command.vi"("error in (no error)"=w829, "Extra"=w834, "Command"=T10."Move to Relative Position", "VISA resource name"=w830) -> ("error out"=w828:errorcluster, "VISA resource name out"=w831:refnum<visa-resource-name>)  [unwired: 3 in, 1 out]
                      }
                      frame #4 {
                        n393 = To Unsigned Long Integer(number=w838) -> (unsigned 32bit integer=w837:u32)
                        n394 = Wait (ms)(milliseconds to wait=w837) -> ()  [unwired: 1 out]
                      }
                      frame #5 {
                        n395 = property on="R Backlash corr" class="Bool (strict)"("Val(Sgnl)"=FALSE ("Value (Signaling)")) -> ()  [unwired: 2 in, 2 out]
                      }
                    }
                  }
                  frame #1 {
                  }
                }
              }
            }
            n396 = flat-sequence {
              tunnel: [w1126] -> w669
              tunnel: [w1125] -> w668
              tunnel: [w1124] -> w667
              tunnel: w605 -> [w1123]
              tunnel: w604 -> [w1122]
              tunnel: [w1148] -> w666
              tunnel: [w1147] -> w665
              tunnel: [w1145] -> w664
              tunnel: [w1146] -> w663
              tunnel: w669 -> [w1145]
              tunnel: w668 -> [w1144]
              tunnel: w667 -> [w1143]
              tunnel: w666 -> [w1162]
              tunnel: [w1162] -> w662
              tunnel: w665 -> [w1161]
              tunnel: [w1161] -> w661
              tunnel: w664 -> [w1160]
              tunnel: [w1160] -> w660
              tunnel: w663 -> [w1159]
              tunnel: [w1159] -> w659
              tunnel: [w1166] -> w658
              tunnel: [w1167] -> w657
              tunnel: [w1163] -> w656
              tunnel: w659 -> [w1163]
              tunnel: w660 -> [w1164]
              tunnel: w661 -> [w1168]
              tunnel: w662 -> [w1165]
              tunnel: w658 -> [w1178]
              tunnel: w657 -> [w1179]
              tunnel: w656 -> [w1181]
              tunnel: [w1177] -> w612
              tunnel: [w1176] -> w613
              frame #0 {
                n397 = call "mdrive send command.vi"("error in (no error)"=w1122, "Extra"="P", "Command"=T10."Print Parameter", "VISA resource name"=w1123) -> ("error out"=w1124:errorcluster, "read buffer"=w1142:string, "VISA resource name out"=w1125:refnum<visa-resource-name>)  [unwired: 3 in]
                n398 = Decimal String To Number(string=w1142, offset=0) -> (number=w1121:i32)  [unwired: 1 in, 1 out]
                n399 = property on="X steps/rev" class="DigNum (strict)"() -> ("Value"=w1135:u32)  [unwired: 2 in, 2 out]
                n400 = To Double Precision Float(number=w1121) -> (double precision float=w1130:dbl)
                n401 = To Double Precision Float(number=w1135) -> (double precision float=w1136:dbl)
                n402 = property on="X Step PV" class="DigNum (strict)"("Val(Sgnl)"=w1121) -> ()  [unwired: 2 in, 2 out]
                n403 = Divide(x=w1130, y=w1136) -> (x/y=w1134:dbl)
                n404 = property on="X Step SP" class="DigNum (strict)"() -> ("Maximum"=w1138:dbl)  [unwired: 2 in, 2 out]
                n405 = property on="X Step SP" class="DigNum (strict)"() -> ("Minimum"=w1140:dbl)  [unwired: 2 in, 2 out]
                n406 = property on="X mm/rev" class="DigNum (strict)"() -> ("Value"=w1133:dbl)  [unwired: 2 in, 2 out]
                n407 = Multiply(x=w1134, y=w1133) -> (x*y=w1132:dbl)
                n408 = To Long Integer(number=w1138) -> (32bit integer=w1137:i32)
                n409 = To Long Integer(number=w1140) -> (32bit integer=w1139:i32)
                n410 = property on="X offset mm" class="DigNum (strict)"() -> ("Value"=w1131:dbl)  [unwired: 2 in, 2 out]
                n411 = In Range and Coerce(upper limit=w1137, x=w1121, lower limit=w1139) -> (In Range?=w1126:bool)  [unwired: 1 out]
                n412 = Add(x=w1132, y=w1131) -> (x+y=w1129:dbl)
                n413 = property on="X  in Range" class="Bool (strict)"("Val(Sgnl)"=w1126) -> ()  [unwired: 2 in, 2 out]
                n414 = property on="X Position mm PV" class="DigNum (strict)"("Val(Sgnl)"=w1129) -> ()  [unwired: 2 in, 2 out]
              }
              frame #1 {
                n415 = call "mdrive send command.vi"("error in (no error)"=w1143, "Extra"="MV", "Command"=T10."Print Parameter", "VISA resource name"=w1144) -> ("error out"=w1147:errorcluster, "read buffer"=w1151:string, "VISA resource name out"=w1148:refnum<visa-resource-name>)  [unwired: 3 in]
                n416 = Not Equal?(x=w1151, y="") -> (x != y?=w1149:bool)
                n417 = Decimal String To Number(string=w1151, offset=0 ("offset (0)")) -> (number=w1154:i32)  [unwired: 1 in, 1 out]
                n418 = property on="X Ready" class="Bool (strict)"("Val(Sgnl)"=w1149) -> ()  [unwired: 2 in, 2 out]
                n419 = Number To Boolean Array(number=w1154) -> (Boolean array=w1153:bool[])
                n420 = Index Array(array=w1153, index=0) -> (element=w1146:bool)
                n421 = property on="X  in Motion" class="Bool (strict)"("Val(Sgnl)"=w1146) -> ()  [unwired: 2 in, 2 out]
              }
              frame #2 {
                n422 = Wait (ms)(milliseconds to wait=u32 50) -> ()  [unwired: 1 out]
              }
              frame #3 {
                n423 = case shown="True" w1164 {
                  tunnel: w1165 -> [w1171 w1175]
                  tunnel: [w1172 w1175] -> w1166
                  tunnel: [w1173 w1174] -> w1167
                  tunnel: w1168 -> [w1170 w1174]
                  frame #0 {
                    n424 = call "mdrive send command.vi"("error in (no error)"=w1170, "Command"=T10."Stop", "VISA resource name"=w1171) -> ("error out"=w1173:errorcluster, "VISA resource name out"=w1172:refnum<visa-resource-name>)  [unwired: 4 in, 1 out]
                  }
                  frame #1 {
                  }
                }
              }
              frame #4 {
                n425 = property on="X Backlash corr" class="Bool (strict)"() -> ("Value"=w1182:bool)  [unwired: 2 in, 2 out]
                n426 = Implies(1:w1181, 2:w1182) -> (0:w1180:bool)
                n427 = case shown="False" w1180 {
                  tunnel: w1179 -> [w1190 w1247]
                  tunnel: w1178 -> [w1189 w1248]
                  tunnel: [w1184 w1247] -> w1177
                  tunnel: [w1188 w1248] -> w1176
                  frame #0 {
                    # "Backlash"
                    n428 = flat-sequence {
                      tunnel: [w1205] -> w1202
                      tunnel: [w1207] -> w1201
                      tunnel: [w1206] -> w1200
                      tunnel: w1190 -> [w1204]
                      tunnel: w1189 -> [w1203]
                      tunnel: w1202 -> [w1215]
                      tunnel: [w1215] -> w1199
                      tunnel: w1201 -> [w1214]
                      tunnel: w1200 -> [w1213]
                      tunnel: [w1212] -> w1198
                      tunnel: [w1211] -> w1197
                      tunnel: [w1210] -> w1187
                      tunnel: w1199 -> [w1229]
                      tunnel: w1198 -> [w1220]
                      tunnel: w1197 -> [w1228]
                      tunnel: [w1220] -> w1196
                      tunnel: [w1228] -> w1195
                      tunnel: [w1219] -> w1192
                      tunnel: [w1227] -> w1191
                      tunnel: w1187 -> [w1227]
                      tunnel: w1196 -> [w1232]
                      tunnel: w1195 -> [w1233]
                      tunnel: [w1231] -> w1194
                      tunnel: [w1239] -> w1193
                      tunnel: w1192 -> [w1239]
                      tunnel: w1191 -> [w1235]
                      tunnel: [w1234] -> w1185
                      tunnel: w1194 -> [w1242]
                      tunnel: w1193 -> [w1241]
                      tunnel: [w1243] -> w1186
                      tunnel: w1185 -> [w1243]
                      tunnel: [w1242] -> w1183
                      tunnel: [w1246] -> w1188
                      tunnel: w1186 -> [w1246]
                      tunnel: [w1244] -> w1184
                      tunnel: w1183 -> [w1244]
                      frame #0 {
                        n429 = property on="X Backlash steps/sec" class="DigNum (strict)"() -> ("Value"=w1205:i32)  [unwired: 2 in, 2 out]
                        n430 = Number To Decimal String(number=w1205) -> (decimal integer string=w1208:string)  [unwired: 1 in]
                        n431 = call "mdrive send command.vi"("error in (no error)"=w1204, "Extra"=w1208, "Command"=T10."Max Velocity", "VISA resource name"=w1203) -> ("error out"=w1206:errorcluster, "VISA resource name out"=w1207:refnum<visa-resource-name>)  [unwired: 3 in, 1 out]
                      }
                      frame #1 {
                        n432 = property on="X Backlash" class="DigNum (strict)"() -> ("Value"=w1210:i32)  [unwired: 2 in, 2 out]
                        n433 = Number To Decimal String(number=w1210) -> (decimal integer string=w1216:string)  [unwired: 1 in]
                        n434 = call "mdrive send command.vi"("error in (no error)"=w1213, "Extra"=w1216, "Command"=T10."Move to Relative Position", "VISA resource name"=w1214) -> ("error out"=w1212:errorcluster, "VISA resource name out"=w1211:refnum<visa-resource-name>)  [unwired: 3 in, 1 out]
                      }
                      frame #2 {
                        n435 = To Double Precision Float(number=w1227) -> (double precision float=w1225:dbl)
                        n436 = To Double Precision Float(number=w1229) -> (double precision float=w1230:dbl)
                        n437 = Absolute Value(x=w1225) -> (abs(x)=w1226:dbl)
                        n438 = Divide(x=w1226, y=w1230) -> (x/y=w1223:dbl)
                        n439 = Multiply(x=1000.0, y=w1223) -> (x*y=w1221:dbl)
                        n440 = Add(x=w1221, y=300.0) -> (x+y=w1219:dbl)
                        n441 = To Unsigned Long Integer(number=w1219) -> (unsigned 32bit integer=w1218:u32)
                        n442 = Wait (ms)(milliseconds to wait=w1218) -> ()  [unwired: 1 out]
                      }
                      frame #3 {
                        n443 = Negate(x=w1235) -> (-x=w1236:i32)
                        n444 = Number To Decimal String(number=w1236) -> (decimal integer string=w1237:string)  [unwired: 1 in]
                        n445 = call "mdrive send command.vi"("error in (no error)"=w1232, "Extra"=w1237, "Command"=T10."Move to Relative Position", "VISA resource name"=w1233) -> ("error out"=w1231:errorcluster, "VISA resource name out"=w1234:refnum<visa-resource-name>)  [unwired: 3 in, 1 out]
                      }
                      frame #4 {
                        n446 = To Unsigned Long Integer(number=w1241) -> (unsigned 32bit integer=w1240:u32)
                        n447 = Wait (ms)(milliseconds to wait=w1240) -> ()  [unwired: 1 out]
                      }
                      frame #5 {
                        n448 = property on="X Backlash corr" class="Bool (strict)"("Val(Sgnl)"=FALSE ("Value (Signaling)")) -> ()  [unwired: 2 in, 2 out]
                      }
                    }
                  }
                  frame #1 {
                  }
                }
              }
            }
            n449 = property on="Scan Go" class="Bool (strict)"() -> ("Value"=w597:bool)  [unwired: 2 in, 2 out]
            n450 = property on="STATUS" class="Str"() -> ("Value"=w595:string)  [unwired: 2 in, 2 out]
            n451 = Equal?(x=w595, y="SCANNING MODE" ("STATUS")) -> (x = y?=w593:bool)
            n452 = Equal?(x=w597, y=TRUE) -> (x = y?=w592:bool)
            n453 = Or(x=w593, y=w592) -> (x .or. y?=w591:bool)
            n454 = case shown="False" w591 {
              frame #0 {
                n455 = property on="X  in Motion" class="Bool (strict)"() -> ("Value"=w674:bool)  [unwired: 2 in, 2 out]
                n456 = property on="Y in Motion" class="Bool (strict)"() -> ("Value"=w673:bool)  [unwired: 2 in, 2 out]
                n457 = property on="Z in Motion" class="Bool (strict)"() -> ("Value"=w676:bool)  [unwired: 2 in, 2 out]
                n458 = property on="R in Motion" class="Bool (strict)"() -> ("Value"=w675:bool)  [unwired: 2 in, 2 out]
                n459 = Compound Arithmetic op=AND(w674, w673, w676, w675) -> (w671:bool)
                n460 = Equal?(x=w671, y=FALSE) -> (x = y?=w672:bool)
                n461 = case shown="True" w672 {
                  frame #0 {
                  }
                  frame #1 {
                    n462 = property on="X Step SP" class="DigNum (strict)"() -> ("Value"=w684:i32)  [unwired: 2 in, 2 out]
                    n463 = property on="Y Step SP" class="DigNum (strict)"() -> ("Value"=w682:i32)  [unwired: 2 in, 2 out]
                    n464 = property on="Z Step SP" class="DigNum (strict)"() -> ("Value"=w680:i32)  [unwired: 2 in, 2 out]
                    n465 = property on="R Step SP" class="DigNum (strict)"() -> ("Value"=w677:i32)  [unwired: 2 in, 2 out]
                    n466 = property on="X Step PV" class="DigNum (strict)"() -> ("Value"=w683:i32)  [unwired: 2 in, 2 out]
                    n467 = property on="Y Step PV" class="DigNum (strict)"() -> ("Value"=w681:i32)  [unwired: 2 in, 2 out]
                    n468 = property on="Z Step PV" class="DigNum (strict)"() -> ("Value"=w679:i32)  [unwired: 2 in, 2 out]
                    n469 = property on="R Step PV" class="DigNum (strict)"() -> ("Value"=w678:i32)  [unwired: 2 in, 2 out]
                    n470 = Equal?(x=w684, y=w683) -> (x = y?=w689:bool)
                    n471 = Equal?(x=w682, y=w681) -> (x = y?=w688:bool)
                    n472 = Equal?(x=w680, y=w679) -> (x = y?=w686:bool)
                    n473 = Equal?(x=w677, y=w678) -> (x = y?=w687:bool)
                    n474 = Compound Arithmetic op=AND(w689, w688, w686, w687) -> (w685:bool)
                    n475 = case shown="True" w685 {
                      frame #0 {
                      }
                      frame #1 {
                        n476 = local write "STATUS"("SCANNING DONE" ("STATUS")) -> ()
                        n477 = property on="GO" class="Bool"("DisabledEnum"=T1."Enabled" ("Disabled")) -> ()  [unwired: 2 in, 2 out]
                      }
                    }
                  }
                }
              }
              frame #1 {
                n478 = property on="X Scan Length SP steps" class="DigNum (strict)"() -> ("Value"=w703:i32)  [unwired: 2 in, 2 out]
                n479 = property on="Y Scan Length SP steps" class="DigNum (strict)"() -> ("Value"=w702:i32)  [unwired: 2 in, 2 out]
                n480 = property on="Z Scan Length SP steps" class="DigNum (strict)"() -> ("Value"=w701:i32)  [unwired: 2 in, 2 out]
                n481 = property on="R Scan Length SP steps" class="DigNum (strict)"() -> ("Value"=w700:i32)  [unwired: 2 in, 2 out]
                n482 = property on="X Step SP" class="DigNum (strict)"() -> ("Value"=w699:i32)  [unwired: 2 in, 2 out]
                n483 = property on="Y Step SP" class="DigNum (strict)"() -> ("Value"=w698:i32)  [unwired: 2 in, 2 out]
                n484 = property on="Z Step SP" class="DigNum (strict)"() -> ("Value"=w697:i32)  [unwired: 2 in, 2 out]
                n485 = property on="R Step SP" class="DigNum (strict)"() -> ("Value"=w696:i32)  [unwired: 2 in, 2 out]
                n486 = Add(x=w703, y=w699) -> (x+y=w712:i32)
                n487 = Add(x=w702, y=w698) -> (x+y=w711:i32)
                n488 = Add(x=w701, y=w697) -> (x+y=w710:i32)
                n489 = Add(x=w700, y=w696) -> (x+y=w709:i32)
                n490 = property on="X Step PV" class="DigNum (strict)"() -> ("Value"=w695:i32)  [unwired: 2 in, 2 out]
                n491 = property on="Y Step PV" class="DigNum (strict)"() -> ("Value"=w694:i32)  [unwired: 2 in, 2 out]
                n492 = property on="Z Step PV" class="DigNum (strict)"() -> ("Value"=w693:i32)  [unwired: 2 in, 2 out]
                n493 = property on="R Step PV" class="DigNum (strict)"() -> ("Value"=w692:i32)  [unwired: 2 in, 2 out]
                n494 = Equal?(x=w695, y=w712) -> (x = y?=w708:bool)
                n495 = Equal?(x=w694, y=w711) -> (x = y?=w707:bool)
                n496 = Equal?(x=w693, y=w710) -> (x = y?=w705:bool)
                n497 = Equal?(x=w692, y=w709) -> (x = y?=w706:bool)
                n498 = Compound Arithmetic op=AND(w708, w707, w705, w706) -> (w704:bool)
                n499 = case shown="True" w704 {
                  frame #0 {
                  }
                  frame #1 {
                    n500 = local write "Scan Go"(FALSE ("Scan Go")) -> ()
                    n501 = local write "STATUS"("DONE" ("STATUS")) -> ()
                    n502 = property on="Review Scan \nParameters" class="Bool"("DisabledEnum"=T1."Enabled" ("Disabled")) -> ()  [unwired: 2 in, 2 out]
                    n503 = property on="Set scan parameter" class="Bool"("DisabledEnum"=T1."Enabled" ("Disabled")) -> ()  [unwired: 2 in, 2 out]
                    n504 = property on="GO" class="Bool"("DisabledEnum"=T1."Enabled" ("Disabled")) -> ()  [unwired: 2 in, 2 out]
                  }
                }
              }
            }
          }
        }
        n505 = Equal?(x=w505, y=T1."Disabled and Grayed Out") -> (x = y?=w502:bool)
        n506 = Equal?(x=w508, y=T1."Enabled") -> (x = y?=w506:bool)
        n507 = And(x=w506, y=w502) -> (x .and. y?=w503:bool)
        n508 = case shown="False" w502 {
          frame #0 {
            n509 = local write "STATUS"("SCANNING MODE" ("STATUS")) -> ()
          }
          frame #1 {
          }
        }
        n510 = case shown="False" w503 {
          frame #0 {
          }
          frame #1 {
            n511 = local write "STATUS"("") -> ()
          }
        }
        n512 = property on="Z Position mm PV" class="DigNum (strict)"() -> ("Value"=w501:dbl)  [unwired: 2 in, 2 out]
        n513 = property on="R Position deg PV" class="DigNum (strict)"() -> ("Value"=w539:dbl)  [unwired: 2 in, 2 out]
        n514 = call "Build XY Graph2"("Reset"=TRUE, "Y Input"=w539, "X Input"=w501) -> ("XY Graph"=→"ZR Graph":cluster{"Y":dbl[], "Y":dbl[]}[])  [unwired: 7 in, 1 out]
        n515 = property on="Y Position mm PV" class="DigNum (strict)"() -> ("Value"=w500:dbl)  [unwired: 2 in, 2 out]
        n516 = property on="X Position mm PV" class="DigNum (strict)"() -> ("Value"=w538:dbl)  [unwired: 2 in, 2 out]
        n517 = call "Build XY Graph"("Reset"=TRUE, "Y Input"=w500, "X Input"=w538) -> ("XY Graph"=→"XY Graph":cluster{"Y":dbl[], "Y":dbl[]}[])  [unwired: 7 in, 1 out]
        n518 = Build Array (concatenate)(w498, w501) -> (w496:dbl[])
        n519 = Build Array (concatenate)(w497, w500) -> (w494:dbl[])
        n520 = Bundle(w496, w494) -> (→"ZY Graph":cluster{dbl[], dbl[]})  [unwired: 1 in]
        n521 = property on="Y Scan Length SP steps" class="DigNum (strict)"() -> ("Value"=w528:i32)  [unwired: 2 in, 2 out]
        n522 = property on="Z Scan Length SP steps" class="DigNum (strict)"() -> ("Value"=w529:i32)  [unwired: 2 in, 2 out]
        n523 = To Double Precision Float(number=w529) -> (double precision float=w522:dbl)
        n524 = To Double Precision Float(number=w528) -> (double precision float=w523:dbl)
        n525 = Divide(x=w523, y=w522) -> (x/y=w530:dbl)
        n526 = Inverse Tangent(1:w530) -> (0:w531:dbl)
        n527 = property on="Clear ZY" class="Bool (strict)"() -> ("Value"=w492:bool)  [unwired: 2 in, 2 out]
        n528 = Divide(x=w531, y=6.283185307179586) -> (x/y=w532:dbl)
        n529 = Multiply(x=360.0, y=w532) -> (x*y=w535:dbl)
        n530 = case shown="False" w492 {
          tunnel: w496 -> [w545 w550]
          tunnel: [w545 w549] -> w495
          tunnel: w494 -> [w544 w548]
          tunnel: [w544 w547] -> w493
          frame #0 {
          }
          frame #1 {
            w546 = 0 ("dimension size")
            n531 = Reshape Array(w550, w546) -> (w549:dbl[])
            n532 = Reshape Array(w548, w546) -> (w547:dbl[])
          }
        }
        n533 = property on="atan Y/Z" class="DigNum (strict)"("Val(Sgnl)"=w535) -> ()  [unwired: 2 in, 2 out]
      }
      event #1 {
        n534 = event-data() -> ()  [unwired: 1 in, 5 out]
        n535 = property on="OK Button" class="Bool (strict)"() -> ("Value"=w1249:bool)  [unwired: 2 in, 2 out]
        n536 = property on="Z Step PV" class="DigNum (strict)"() -> ("Value"=w1254:i32)  [unwired: 2 in, 2 out]
        n537 = Greater?(x=w1254, y=15360000) -> (0:w1251:bool)
        n538 = Equal?(x=w1249, y=TRUE) -> (x = y?=w1252:bool)
        n539 = And(x=w1252, y=w1251) -> (x .and. y?=w1250:bool)
        n540 = case shown="False" w1250 {
          frame #0 {
            n541 = property on="Z Step PV" class="DigNum (strict)"() -> ("Value"=w1270:i32)  [unwired: 2 in, 2 out]
            n542 = property on="OK Button" class="Bool (strict)"() -> ("Value"=w1265:bool)  [unwired: 2 in, 2 out]
            n543 = Greater?(x=w1270, y=15360000) -> (0:w1268:bool)
            n544 = Equal?(x=w1265, y=FALSE) -> (x = y?=w1267:bool)
            n545 = And(x=w1267, y=w1268) -> (x .and. y?=w1266:bool)
            n546 = case shown="True" w1266 {
              frame #0 {
              }
              frame #1 {
                n547 = One Button Dialog(message="YOU CAN'T CLOSE THE VALVE\nWHEN YOU ARE IN THE THIS\nPOSITION!!") -> (true=w1272:bool)  [unwired: 1 in]
                n548 = property on="OK Button" class="Bool (strict)"("Val(Sgnl)"=w1272) -> ()  [unwired: 2 in, 2 out]
              }
            }
          }
          frame #1 {
            n549 = flat-sequence {
              frame #0 {
                n550 = local read "OK Button"() -> (w1275:bool)
                n551 = call "DigitalIO_sub_V1_CNTL.vi"("OK Button"=w1275) -> ("Boolean"=w1274:bool)  [unwired: 2 in]
                n552 = property on="Valve \nopend/closed" class="Bool (strict)"("Val(Sgnl)"=w1274) -> ()  [unwired: 2 in, 2 out]
              }
              frame #1 {
                n553 = call "DigitalIO_sub_V1_MON.vi"() -> ("CL"=w1277:bool, "OP"=w1276:bool)  [unwired: 8 in]
                n554 = property on="OP" class="Bool (strict)"("Val(Sgnl)"=w1276) -> ()  [unwired: 2 in, 2 out]
                n555 = property on="CL" class="Bool (strict)"("Val(Sgnl)"=w1277) -> ()  [unwired: 2 in, 2 out]
              }
              frame #2 {
                n556 = Wait (ms)(milliseconds to wait=u32 100) -> ()  [unwired: 1 out]
              }
            }
          }
        }
        n557 = local write "STATUS"("VALVE CHANGED" ("STATUS")) -> ()
      }
      event #2 {
        n558 = event-data() -> ()  [unwired: 1 in, 7 out]
        n559 = property on="X Position mm PV" class="DigNum (strict)"() -> ("Value"=w1291:dbl)  [unwired: 2 in, 2 out]
        n560 = property on="X Position SP mm" class="DigNum (strict)"() -> ("Value"=w1290:dbl)  [unwired: 2 in, 2 out]
        n561 = property on="Z Position mm PV" class="DigNum (strict)"() -> ("Value"=w1287:dbl)  [unwired: 2 in, 2 out]
        n562 = property on="Z Position SP mm" class="DigNum (strict)"() -> ("Value"=w1279:dbl)  [unwired: 2 in, 2 out]
        n563 = property on="R Position SP deg" class="DigNum (strict)"() -> ("Value"=w1282:dbl)  [unwired: 2 in, 2 out]
        n564 = property on="R Position deg PV" class="DigNum (strict)"() -> ("Value"=w1281:dbl)  [unwired: 2 in, 2 out]
        n565 = property on="Y Position mm PV" class="DigNum (strict)"() -> ("Value"=w1285:dbl)  [unwired: 2 in, 2 out]
        n566 = property on="Y Position SP mm" class="DigNum (strict)"() -> ("Value"=w1284:dbl)  [unwired: 2 in, 2 out]
        n567 = Not Equal?(x=w1291, y=w1290) -> (x != y?=w1289:bool)
        n568 = Not Equal?(x=w1287, y=w1279) -> (x != y?=w1288:bool)
        n569 = Not Equal?(x=w1285, y=w1284) -> (x != y?=w1286:bool)
        n570 = Not Equal?(x=w1282, y=w1281) -> (x != y?=w1283:bool)
        n571 = case shown="True" w1288 {
          tunnel: w1304 -> [w1449 w1456]
          tunnel: w1303 -> [w1450 w1455]
          tunnel: [w1450 w1454] -> w1302
          tunnel: [w1449 w1453] -> w1301
          frame #0 {
          }
          frame #1 {
            n572 = flat-sequence {
              tunnel: w1455 -> [w1478]
              tunnel: w1456 -> [w1479]
              tunnel: [w1479] -> w1452
              tunnel: [w1478] -> w1451
              tunnel: [w1494] -> w1470
              tunnel: [w1493] -> w1469
              tunnel: [w1481] -> w1468
              tunnel: w1452 -> [w1494]
              tunnel: w1451 -> [w1493]
              tunnel: [w1497] -> w1467
              tunnel: [w1496] -> w1466
              tunnel: [w1495] -> w1465
              tunnel: w1468 -> [w1495]
              tunnel: w1469 -> [w1496]
              tunnel: w1470 -> [w1497]
              tunnel: [w1513] -> w1464
              tunnel: [w1512] -> w1463
              tunnel: w1467 -> [w1511]
              tunnel: w1466 -> [w1510]
              tunnel: [w1509] -> w1462
              tunnel: w1465 -> [w1509]
              tunnel: w1464 -> [w1520]
              tunnel: [w1520] -> w1461
              tunnel: w1463 -> [w1519]
              tunnel: [w1519] -> w1460
              tunnel: w1462 -> [w1518]
              tunnel: [w1518] -> w1459
              tunnel: [w1525] -> w1458
              tunnel: [w1524] -> w1457
              tunnel: w1461 -> [w1523]
              tunnel: w1460 -> [w1522]
              tunnel: w1459 -> [w1521]
              tunnel: [w1529] -> w1453
              tunnel: [w1530] -> w1454
              tunnel: w1458 -> [w1530]
              tunnel: w1457 -> [w1529]
              frame #0 {
                n573 = property on="Z Position SP mm" class="DigNum (strict)"() -> ("Value"=w1473:dbl)  [unwired: 2 in, 2 out]
                n574 = property on="Z Position mm PV" class="DigNum (strict)"() -> ("Value"=w1471:dbl)  [unwired: 2 in, 2 out]
                n575 = Greater?(x=w1473, y=60.0) -> (0:w1476:bool)
                n576 = Less?(x=w1471, y=60.0) -> (x < y?=w1475:bool)
                n577 = And(x=w1475, y=w1476) -> (x .and. y?=w1477:bool)
                n578 = case shown="True" w1477 {
                  frame #0 {
                  }
                  frame #1 {
                    n579 = property on="Z Position SP mm" class="DigNum (strict)"("Val(Sgnl)"=60.0 ("Value (Signaling)")) -> ()  [unwired: 2 in, 2 out]
                  }
                }
              }
              frame #1 {
                n580 = property on="Z Position SP mm" class="DigNum (strict)"() -> ("Value"=w1487:dbl)  [unwired: 2 in, 2 out]
                n581 = property on="Z offset mm" class="DigNum (strict)"() -> ("Value"=w1488:dbl)  [unwired: 2 in, 2 out]
                n582 = property on="Z mm/rev" class="DigNum (strict)"() -> ("Value"=w1489:dbl)  [unwired: 2 in, 2 out]
                n583 = property on="Z steps/rev" class="DigNum (strict)"() -> ("Value"=w1490:u32)  [unwired: 2 in, 2 out]
                n584 = To Double Precision Float(number=w1490) -> (double precision float=w1486:dbl)
                n585 = Subtract(x=w1487, y=w1488) -> (x-y=w1483:dbl)
                n586 = Divide(x=w1483, y=w1489) -> (x/y=w1482:dbl)
                n587 = property on="Z Step SP" class="DigNum (strict)"() -> ("Maximum"=w1492:dbl)  [unwired: 2 in, 2 out]
                n588 = property on="Z Step SP" class="DigNum (strict)"() -> ("Minimum"=w1491:dbl)  [unwired: 2 in, 2 out]
                n589 = Multiply(x=w1482, y=w1486) -> (x*y=w1484:dbl)
                n590 = In Range and Coerce(upper limit=w1492, x=w1484, lower limit=w1491) -> (coerced(x)=w1485:dbl)  [unwired: 1 out]
                n591 = To Long Integer(number=w1485) -> (32bit integer=w1481:i32)
                n592 = property on="Z Step SP" class="DigNum (strict)"("Val(Sgnl)"=w1481) -> ()  [unwired: 2 in, 2 out]
              }
              frame #2 {
                n593 = property on="Z Step SP" class="DigNum (strict)"() -> ("Value"=w1506:i32)  [unwired: 2 in, 2 out]
                n594 = property on="Z Step PV" class="DigNum (strict)"() -> ("Value"=w1505:i32)  [unwired: 2 in, 2 out]
                n595 = property on="Z Backlash" class="DigNum (strict)"() -> ("Value"=w1498:i32)  [unwired: 2 in, 2 out]
                n596 = Subtract(x=w1506, y=w1505) -> (x-y=w1504:i32)
                n597 = Sign(1:w1498) -> (0:w1502:i32)
                n598 = Sign(1:w1504) -> (0:w1503:i32)
                n599 = Multiply(x=w1503, y=w1502) -> (x*y=w1501:i32)
                n600 = Equal?(x=w1501, y=1) -> (x = y?=w1499:bool)
                n601 = case shown="False" w1499 {
                  frame #0 {
                    n602 = property on="Z Backlash corr" class="Bool (strict)"("Val(Sgnl)"=FALSE ("Value (Signaling)")) -> ()  [unwired: 2 in, 2 out]
                  }
                  frame #1 {
                    n603 = property on="Z Backlash corr" class="Bool (strict)"("Val(Sgnl)"=TRUE ("Value (Signaling)")) -> ()  [unwired: 2 in, 2 out]
                  }
                }
              }
              frame #3 {
                # "Velocity Setting"
                n604 = property on="Z Velocity SP step/sec" class="DigNum (strict)"() -> ("Value"=w1514:i32)  [unwired: 2 in, 2 out]
                n605 = Number To Decimal String(number=w1514) -> (decimal integer string=w1515:string)  [unwired: 1 in]
                n606 = call "mdrive send command.vi"("error in (no error)"=w1511, "Extra"=w1515, "Command"=T10."Max Velocity", "VISA resource name"=w1510) -> ("error out"=w1512:errorcluster, "VISA resource name out"=w1513:refnum<visa-resource-name>)  [unwired: 3 in, 1 out]
              }
              frame #4 {
                n607 = Wait (ms)(milliseconds to wait=u32 50) -> ()  [unwired: 1 out]
              }
              frame #5 {
                # "Move to Abs Position"
                n608 = Number To Decimal String(number=w1521) -> (decimal integer string=w1527:string)  [unwired: 1 in]
                n609 = call "mdrive send command.vi"("error in (no error)"=w1522, "Extra"=w1527, "Command"=T10."Move to Absolute Position", "VISA resource name"=w1523) -> ("error out"=w1524:errorcluster, "VISA resource name out"=w1525:refnum<visa-resource-name>)  [unwired: 3 in, 1 out]
              }
              frame #6 {
                n610 = Wait (ms)(milliseconds to wait=u32 50) -> ()  [unwired: 1 out]
              }
            }
          }
        }
        n611 = case shown="True" w1289 {
          tunnel: w1308 -> [w1532 w1536]
          tunnel: w1307 -> [w1531 w1535]
          tunnel: [w1532 w1534] -> w1306
          tunnel: [w1531 w1533] -> w1305
          frame #0 {
          }
          frame #1 {
            n612 = flat-sequence {
              tunnel: w1535 -> [w1563]
              tunnel: w1536 -> [w1564]
              tunnel: [w1564] -> w1550
              tunnel: [w1563] -> w1549
              tunnel: [w1552] -> w1548
              tunnel: [w1567] -> w1547
              tunnel: [w1566] -> w1546
              tunnel: [w1565] -> w1545
              tunnel: w1548 -> [w1565]
              tunnel: w1549 -> [w1566]
              tunnel: w1550 -> [w1567]
              tunnel: [w1583] -> w1544
              tunnel: [w1582] -> w1543
              tunnel: w1547 -> [w1581]
              tunnel: w1546 -> [w1580]
              tunnel: w1545 -> [w1579]
              tunnel: [w1579] -> w1542
              tunnel: w1544 -> [w1590]
              tunnel: [w1590] -> w1541
              tunnel: w1543 -> [w1589]
              tunnel: [w1589] -> w1540
              tunnel: [w1587] -> w1539
              tunnel: w1542 -> [w1587]
              tunnel: [w1595] -> w1538
              tunnel: [w1594] -> w1537
              tunnel: w1541 -> [w1593]
              tunnel: w1540 -> [w1592]
              tunnel: w1539 -> [w1591]
              tunnel: [w1599] -> w1533
              tunnel: [w1600] -> w1534
              tunnel: w1538 -> [w1600]
              tunnel: w1537 -> [w1599]
              frame #0 {
                n613 = property on="X Position SP mm" class="DigNum (strict)"() -> ("Value"=w1560:dbl)  [unwired: 2 in, 2 out]
                n614 = property on="X offset mm" class="DigNum (strict)"() -> ("Value"=w1561:dbl)  [unwired: 2 in, 2 out]
                n615 = property on="X mm/rev" class="DigNum (strict)"() -> ("Value"=w1551:dbl)  [unwired: 2 in, 2 out]
                n616 = property on="X steps/rev" class="DigNum (strict)"() -> ("Value"=w1562:u32)  [unwired: 2 in, 2 out]
                n617 = To Double Precision Float(number=w1562) -> (double precision float=w1557:dbl)
                n618 = Subtract(x=w1560, y=w1561) -> (x-y=w1554:dbl)
                n619 = Divide(x=w1554, y=w1551) -> (x/y=w1553:dbl)
                n620 = Multiply(x=w1553, y=w1557) -> (x*y=w1555:dbl)
                n621 = property on="X Step SP" class="DigNum (strict)"() -> ("Maximum"=w1559:dbl)  [unwired: 2 in, 2 out]
                n622 = property on="X Step SP" class="DigNum (strict)"() -> ("Minimum"=w1558:dbl)  [unwired: 2 in, 2 out]
                n623 = In Range and Coerce(upper limit=w1559, x=w1555, lower limit=w1558) -> (coerced(x)=w1556:dbl)  [unwired: 1 out]
                n624 = To Long Integer(number=w1556) -> (32bit integer=w1552:i32)
                n625 = property on="X Step SP" class="DigNum (strict)"("Val(Sgnl)"=w1552) -> ()  [unwired: 2 in, 2 out]
              }
              frame #1 {
                n626 = property on="X Step SP" class="DigNum (strict)"() -> ("Value"=w1576:i32)  [unwired: 2 in, 2 out]
                n627 = property on="X Step PV" class="DigNum (strict)"() -> ("Value"=w1575:i32)  [unwired: 2 in, 2 out]
                n628 = property on="X Backlash" class="DigNum (strict)"() -> ("Value"=w1568:i32)  [unwired: 2 in, 2 out]
                n629 = Sign(1:w1568) -> (0:w1572:i32)
                n630 = Subtract(x=w1576, y=w1575) -> (x-y=w1574:i32)
                n631 = Sign(1:w1574) -> (0:w1573:i32)
                n632 = Multiply(x=w1573, y=w1572) -> (x*y=w1571:i32)
                n633 = Equal?(x=w1571, y=1) -> (x = y?=w1569:bool)
                n634 = case shown="False" w1569 {
                  frame #0 {
                    n635 = property on="X Backlash corr" class="Bool (strict)"("Val(Sgnl)"=FALSE ("Value (Signaling)")) -> ()  [unwired: 2 in, 2 out]
                  }
                  frame #1 {
                    n636 = property on="X Backlash corr" class="Bool (strict)"("Val(Sgnl)"=TRUE ("Value (Signaling)")) -> ()  [unwired: 2 in, 2 out]
                  }
                }
              }
              frame #2 {
                # "Velocity Setting"
                n637 = property on="X Velocity SP step/sec" class="DigNum (strict)"() -> ("Value"=w1584:i32)  [unwired: 2 in, 2 out]
                n638 = Number To Decimal String(number=w1584) -> (decimal integer string=w1585:string)  [unwired: 1 in]
                n639 = call "mdrive send command.vi"("error in (no error)"=w1580, "Extra"=w1585, "Command"=T10."Max Velocity", "VISA resource name"=w1581) -> ("error out"=w1582:errorcluster, "VISA resource name out"=w1583:refnum<visa-resource-name>)  [unwired: 3 in, 1 out]
              }
              frame #3 {
                n640 = Wait (ms)(milliseconds to wait=u32 50) -> ()  [unwired: 1 out]
              }
              frame #4 {
                # "Move to Abs Position"
                n641 = Number To Decimal String(number=w1591) -> (decimal integer string=w1597:string)  [unwired: 1 in]
                n642 = call "mdrive send command.vi"("error in (no error)"=w1592, "Extra"=w1597, "Command"=T10."Move to Absolute Position", "VISA resource name"=w1593) -> ("error out"=w1594:errorcluster, "VISA resource name out"=w1595:refnum<visa-resource-name>)  [unwired: 3 in, 1 out]
              }
              frame #5 {
                n643 = Wait (ms)(milliseconds to wait=u32 50) -> ()  [unwired: 1 out]
              }
            }
          }
        }
        n644 = case shown="True" w1286 {
          tunnel: w1300 -> [w1379 w1384]
          tunnel: w1299 -> [w1380 w1383]
          tunnel: [w1380 w1382] -> w1298
          tunnel: [w1379 w1381] -> w1297
          frame #0 {
          }
          frame #1 {
            n645 = flat-sequence {
              tunnel: [w1412] -> w1398
              tunnel: [w1411] -> w1397
              tunnel: [w1399] -> w1396
              tunnel: w1383 -> [w1411]
              tunnel: w1384 -> [w1412]
              tunnel: [w1415] -> w1395
              tunnel: [w1414] -> w1394
              tunnel: [w1413] -> w1393
              tunnel: w1396 -> [w1413]
              tunnel: w1397 -> [w1414]
              tunnel: w1398 -> [w1415]
              tunnel: [w1431] -> w1392
              tunnel: [w1430] -> w1391
              tunnel: w1395 -> [w1429]
              tunnel: w1394 -> [w1428]
              tunnel: [w1427] -> w1390
              tunnel: w1393 -> [w1427]
              tunnel: w1392 -> [w1438]
              tunnel: [w1438] -> w1389
              tunnel: w1391 -> [w1437]
              tunnel: [w1437] -> w1388
              tunnel: [w1435] -> w1387
              tunnel: w1390 -> [w1435]
              tunnel: [w1443] -> w1386
              tunnel: [w1442] -> w1385
              tunnel: w1389 -> [w1441]
              tunnel: w1388 -> [w1440]
              tunnel: w1387 -> [w1439]
              tunnel: [w1446] -> w1381
              tunnel: [w1448] -> w1382
              tunnel: w1386 -> [w1448]
              tunnel: w1385 -> [w1446]
              frame #0 {
                n646 = property on="Y Position SP mm" class="DigNum (strict)"() -> ("Value"=w1405:dbl)  [unwired: 2 in, 2 out]
                n647 = property on="Y offset mm" class="DigNum (strict)"() -> ("Value"=w1406:dbl)  [unwired: 2 in, 2 out]
                n648 = property on="Y mm/rev" class="DigNum (strict)"() -> ("Value"=w1407:dbl)  [unwired: 2 in, 2 out]
                n649 = property on="Y steps/rev" class="DigNum (strict)"() -> ("Value"=w1408:u32)  [unwired: 2 in, 2 out]
                n650 = To Double Precision Float(number=w1408) -> (double precision float=w1404:dbl)
                n651 = Subtract(x=w1405, y=w1406) -> (x-y=w1401:dbl)
                n652 = Divide(x=w1401, y=w1407) -> (x/y=w1400:dbl)
                n653 = Multiply(x=w1400, y=w1404) -> (x*y=w1402:dbl)
                n654 = property on="Y Step SP" class="DigNum (strict)"() -> ("Maximum"=w1409:dbl)  [unwired: 2 in, 2 out]
                n655 = property on="Y Step SP" class="DigNum (strict)"() -> ("Minimum"=w1410:dbl)  [unwired: 2 in, 2 out]
                n656 = In Range and Coerce(upper limit=w1409, x=w1402, lower limit=w1410) -> (coerced(x)=w1403:dbl)  [unwired: 1 out]
                n657 = To Long Integer(number=w1403) -> (32bit integer=w1399:i32)
                n658 = property on="Y Step SP" class="DigNum (strict)"("Val(Sgnl)"=w1399) -> ()  [unwired: 2 in, 2 out]
              }
              frame #1 {
                n659 = property on="Y Step SP" class="DigNum (strict)"() -> ("Value"=w1424:i32)  [unwired: 2 in, 2 out]
                n660 = property on="Y Step PV" class="DigNum (strict)"() -> ("Value"=w1423:i32)  [unwired: 2 in, 2 out]
                n661 = property on="Y Backlash" class="DigNum (strict)"() -> ("Value"=w1416:i32)  [unwired: 2 in, 2 out]
                n662 = Subtract(x=w1424, y=w1423) -> (x-y=w1422:i32)
                n663 = Sign(1:w1416) -> (0:w1420:i32)
                n664 = Sign(1:w1422) -> (0:w1421:i32)
                n665 = Multiply(x=w1421, y=w1420) -> (x*y=w1419:i32)
                n666 = Equal?(x=w1419, y=1) -> (x = y?=w1417:bool)
                n667 = case shown="False" w1417 {
                  frame #0 {
                    n668 = property on="Y Backlash corr" class="Bool (strict)"("Val(Sgnl)"=FALSE ("Value (Signaling)")) -> ()  [unwired: 2 in, 2 out]
                  }
                  frame #1 {
                    n669 = property on="Y Backlash corr" class="Bool (strict)"("Val(Sgnl)"=TRUE ("Value (Signaling)")) -> ()  [unwired: 2 in, 2 out]
                  }
                }
              }
              frame #2 {
                # "Velocity Setting"
                n670 = property on="Y Velocity SP step/sec" class="DigNum (strict)"() -> ("Value"=w1432:i32)  [unwired: 2 in, 2 out]
                n671 = Number To Decimal String(number=w1432) -> (decimal integer string=w1433:string)  [unwired: 1 in]
                n672 = call "mdrive send command.vi"("error in (no error)"=w1429, "Extra"=w1433, "Command"=T10."Max Velocity", "VISA resource name"=w1428) -> ("error out"=w1430:errorcluster, "VISA resource name out"=w1431:refnum<visa-resource-name>)  [unwired: 3 in, 1 out]
              }
              frame #3 {
                n673 = Wait (ms)(milliseconds to wait=u32 50) -> ()  [unwired: 1 out]
              }
              frame #4 {
                # "Move to Abs Position"
                n674 = Number To Decimal String(number=w1439) -> (decimal integer string=w1445:string)  [unwired: 1 in]
                n675 = call "mdrive send command.vi"("error in (no error)"=w1440, "Extra"=w1445, "Command"=T10."Move to Absolute Position", "VISA resource name"=w1441) -> ("error out"=w1442:errorcluster, "VISA resource name out"=w1443:refnum<visa-resource-name>)  [unwired: 3 in, 1 out]
              }
              frame #5 {
                n676 = Wait (ms)(milliseconds to wait=u32 25) -> ()  [unwired: 1 out]
              }
            }
          }
        }
        n677 = case shown="True" w1283 {
          tunnel: w1296 -> [w1309 w1314]
          tunnel: w1295 -> [w1310 w1313]
          tunnel: [w1310 w1312] -> w1294
          tunnel: [w1309 w1311] -> w1293
          frame #0 {
          }
          frame #1 {
            n678 = flat-sequence {
              tunnel: w1313 -> [w1341]
              tunnel: w1314 -> [w1342]
              tunnel: [w1342] -> w1328
              tunnel: [w1341] -> w1327
              tunnel: [w1329] -> w1326
              tunnel: [w1345] -> w1325
              tunnel: [w1344] -> w1324
              tunnel: [w1343] -> w1323
              tunnel: w1326 -> [w1343]
              tunnel: w1327 -> [w1344]
              tunnel: w1328 -> [w1345]
              tunnel: [w1361] -> w1322
              tunnel: [w1360] -> w1321
              tunnel: w1325 -> [w1359]
              tunnel: w1324 -> [w1358]
              tunnel: [w1357] -> w1320
              tunnel: w1323 -> [w1357]
              tunnel: w1322 -> [w1368]
              tunnel: [w1368] -> w1319
              tunnel: w1321 -> [w1367]
              tunnel: [w1367] -> w1318
              tunnel: w1320 -> [w1366]
              tunnel: [w1366] -> w1317
              tunnel: [w1373] -> w1316
              tunnel: [w1372] -> w1315
              tunnel: w1319 -> [w1371]
              tunnel: w1318 -> [w1370]
              tunnel: w1317 -> [w1369]
              tunnel: [w1378] -> w1312
              tunnel: w1316 -> [w1378]
              tunnel: w1315 -> [w1377]
              tunnel: [w1377] -> w1311
              frame #0 {
                n679 = property on="R Position SP deg" class="DigNum (strict)"() -> ("Value"=w1339:dbl)  [unwired: 2 in, 2 out]
                n680 = property on="R offset deg" class="DigNum (strict)"() -> ("Value"=w1338:dbl)  [unwired: 2 in, 2 out]
                n681 = property on="R deg/rev" class="DigNum (strict)"() -> ("Value"=w1340:dbl)  [unwired: 2 in, 2 out]
                n682 = property on="R steps/rev" class="DigNum (strict)"() -> ("Value"=w1337:u32)  [unwired: 2 in, 2 out]
                n683 = To Double Precision Float(number=w1337) -> (double precision float=w1334:dbl)
                n684 = Subtract(x=w1339, y=w1338) -> (x-y=w1331:dbl)
                n685 = Divide(x=w1331, y=w1340) -> (x/y=w1330:dbl)
                n686 = Multiply(x=w1330, y=w1334) -> (x*y=w1332:dbl)
                n687 = property on="R Step SP" class="DigNum (strict)"() -> ("Maximum"=w1335:dbl)  [unwired: 2 in, 2 out]
                n688 = property on="R Step SP" class="DigNum (strict)"() -> ("Minimum"=w1336:dbl)  [unwired: 2 in, 2 out]
                n689 = In Range and Coerce(upper limit=w1335, x=w1332, lower limit=w1336) -> (coerced(x)=w1333:dbl)  [unwired: 1 out]
                n690 = To Long Integer(number=w1333) -> (32bit integer=w1329:i32)
                n691 = property on="R Step SP" class="DigNum (strict)"("Val(Sgnl)"=w1329) -> ()  [unwired: 2 in, 2 out]
              }
              frame #1 {
                n692 = property on="R Step SP" class="DigNum (strict)"() -> ("Value"=w1354:i32)  [unwired: 2 in, 2 out]
                n693 = property on="R Step PV" class="DigNum (strict)"() -> ("Value"=w1353:i32)  [unwired: 2 in, 2 out]
                n694 = property on="R Backlash" class="DigNum (strict)"() -> ("Value"=w1346:i32)  [unwired: 2 in, 2 out]
                n695 = Subtract(x=w1354, y=w1353) -> (x-y=w1352:i32)
                n696 = Sign(1:w1346) -> (0:w1350:i32)
                n697 = Sign(1:w1352) -> (0:w1351:i32)
                n698 = Multiply(x=w1351, y=w1350) -> (x*y=w1349:i32)
                n699 = Equal?(x=w1349, y=1) -> (x = y?=w1347:bool)
                n700 = case shown="False" w1347 {
                  frame #0 {
                    n701 = property on="R Backlash corr" class="Bool (strict)"("Val(Sgnl)"=FALSE ("Value (Signaling)")) -> ()  [unwired: 2 in, 2 out]
                  }
                  frame #1 {
                    n702 = property on="R Backlash corr" class="Bool (strict)"("Val(Sgnl)"=TRUE ("Value (Signaling)")) -> ()  [unwired: 2 in, 2 out]
                  }
                }
              }
              frame #2 {
                # "Velocity Setting"
                n703 = property on="R Velocity SP step/sec" class="DigNum (strict)"() -> ("Value"=w1362:i32)  [unwired: 2 in, 2 out]
                n704 = Number To Decimal String(number=w1362) -> (decimal integer string=w1363:string)  [unwired: 1 in]
                n705 = call "mdrive send command.vi"("error in (no error)"=w1359, "Extra"=w1363, "Command"=T10."Max Velocity", "VISA resource name"=w1358) -> ("error out"=w1360:errorcluster, "VISA resource name out"=w1361:refnum<visa-resource-name>)  [unwired: 3 in, 1 out]
              }
              frame #3 {
                n706 = Wait (ms)(milliseconds to wait=u32 50) -> ()  [unwired: 1 out]
              }
              frame #4 {
                # "Move to Abs Position"
                n707 = Number To Decimal String(number=w1369) -> (decimal integer string=w1375:string)  [unwired: 1 in]
                n708 = call "mdrive send command.vi"("error in (no error)"=w1370, "Extra"=w1375, "Command"=T10."Move to Absolute Position", "VISA resource name"=w1371) -> ("error out"=w1372:errorcluster, "VISA resource name out"=w1373:refnum<visa-resource-name>)  [unwired: 3 in, 1 out]
              }
              frame #5 {
                n709 = Wait (ms)(milliseconds to wait=u32 25) -> ()  [unwired: 1 out]
              }
            }
          }
        }
        n710 = property on="GO" class="Bool"("DisabledEnum"=T1."Disabled and Grayed Out" ("Disabled")) -> ()  [unwired: 2 in, 2 out]
        n711 = local write "STATUS"("MOVING" ("STATUS")) -> ()
      }
      event #3 {
        n712 = event-data() -> ()  [unwired: 1 in, 7 out]
        n713 = flat-sequence {
          tunnel: w1632 -> [w1687]
          tunnel: [w1686] -> w1626
          tunnel: w1611 -> [w1685]
          tunnel: [w1684] -> w1609
          tunnel: [w1691] -> w1627
          tunnel: w1626 -> [w1691]
          tunnel: [w1690] -> w1610
          tunnel: w1609 -> [w1690]
          tunnel: w1627 -> [w1708]
          tunnel: w1610 -> [w1705]
          tunnel: [w1704] -> w1603
          tunnel: [w1703] -> w1602
          frame #0 {
            n714 = call "mdrive send command.vi"("error in (no error)"=w1687, "Command"=T10."Stop", "VISA resource name"=w1685) -> ("error out"=w1686:errorcluster, "VISA resource name out"=w1684:refnum<visa-resource-name>)  [unwired: 4 in, 1 out]
          }
          frame #1 {
            n715 = Wait (ms)(milliseconds to wait=u32 50) -> ()  [unwired: 1 out]
          }
          frame #2 {
            n716 = call "mdrive send command.vi"("error in (no error)"=w1708, "Extra"="P", "Command"=T10."Print Parameter", "VISA resource name"=w1705) -> ("error out"=w1703:errorcluster, "read buffer"=w1698:string, "VISA resource name out"=w1704:refnum<visa-resource-name>)  [unwired: 3 in]
            n717 = property on="Z steps/rev" class="DigNum (strict)"() -> ("Value"=w1694:u32)  [unwired: 2 in, 2 out]
            n718 = Decimal String To Number(string=w1698, offset=0) -> (number=w1696:i32)  [unwired: 1 in, 1 out]
            n719 = property on="Z mm/rev" class="DigNum (strict)"() -> ("Value"=w1693:dbl)  [unwired: 2 in, 2 out]
            n720 = property on="Z Step PV" class="DigNum (strict)"("Val(Sgnl)"=w1696) -> ()  [unwired: 2 in, 2 out]
            n721 = To Double Precision Float(number=w1696) -> (double precision float=w1700:dbl)
            n722 = To Double Precision Float(number=w1694) -> (double precision float=w1699:dbl)
            n723 = property on="Z offset mm" class="DigNum (strict)"() -> ("Value"=w1692:dbl)  [unwired: 2 in, 2 out]
            n724 = Divide(x=w1700, y=w1699) -> (x/y=w1702:dbl)
            n725 = Multiply(x=w1702, y=w1693) -> (x*y=w1701:dbl)
            n726 = Add(x=w1701, y=w1692) -> (x+y=w1695:dbl)
            n727 = property on="Z Position mm PV" class="DigNum (strict)"("Val(Sgnl)"=w1695) -> ()  [unwired: 2 in, 2 out]
          }
        }
        n728 = flat-sequence {
          tunnel: w1633 -> [w1662]
          tunnel: [w1661] -> w1628
          tunnel: w1608 -> [w1660]
          tunnel: [w1659] -> w1606
          tunnel: [w1666] -> w1629
          tunnel: w1628 -> [w1666]
          tunnel: [w1665] -> w1607
          tunnel: w1606 -> [w1665]
          tunnel: w1629 -> [w1683]
          tunnel: w1607 -> [w1680]
          tunnel: [w1679] -> w1605
          tunnel: [w1678] -> w1604
          frame #0 {
            n729 = call "mdrive send command.vi"("error in (no error)"=w1662, "Command"=T10."Stop", "VISA resource name"=w1660) -> ("error out"=w1661:errorcluster, "VISA resource name out"=w1659:refnum<visa-resource-name>)  [unwired: 4 in, 1 out]
          }
          frame #1 {
            n730 = Wait (ms)(milliseconds to wait=u32 50) -> ()  [unwired: 1 out]
          }
          frame #2 {
            n731 = call "mdrive send command.vi"("error in (no error)"=w1683, "Extra"="P", "Command"=T10."Print Parameter", "VISA resource name"=w1680) -> ("error out"=w1678:errorcluster, "read buffer"=w1673:string, "VISA resource name out"=w1679:refnum<visa-resource-name>)  [unwired: 3 in]
            n732 = property on="X steps/rev" class="DigNum (strict)"() -> ("Value"=w1669:u32)  [unwired: 2 in, 2 out]
            n733 = Decimal String To Number(string=w1673, offset=0) -> (number=w1671:i32)  [unwired: 1 in, 1 out]
            n734 = property on="X mm/rev" class="DigNum (strict)"() -> ("Value"=w1668:dbl)  [unwired: 2 in, 2 out]
            n735 = property on="X Step PV" class="DigNum (strict)"("Val(Sgnl)"=w1671) -> ()  [unwired: 2 in, 2 out]
            n736 = To Double Precision Float(number=w1671) -> (double precision float=w1675:dbl)
            n737 = To Double Precision Float(number=w1669) -> (double precision float=w1674:dbl)
            n738 = property on="X offset mm" class="DigNum (strict)"() -> ("Value"=w1667:dbl)  [unwired: 2 in, 2 out]
            n739 = Divide(x=w1675, y=w1674) -> (x/y=w1677:dbl)
            n740 = Multiply(x=w1677, y=w1668) -> (x*y=w1676:dbl)
            n741 = Add(x=w1676, y=w1667) -> (x+y=w1670:dbl)
            n742 = property on="X Position mm PV" class="DigNum (strict)"("Val(Sgnl)"=w1670) -> ()  [unwired: 2 in, 2 out]
          }
        }
        n743 = flat-sequence {
          tunnel: w1631 -> [w1712]
          tunnel: [w1711] -> w1624
          tunnel: w1618 -> [w1710]
          tunnel: [w1709] -> w1616
          tunnel: [w1716] -> w1625
          tunnel: w1624 -> [w1716]
          tunnel: [w1715] -> w1617
          tunnel: w1616 -> [w1715]
          tunnel: w1625 -> [w1733]
          tunnel: w1617 -> [w1730]
          tunnel: [w1729] -> w1615
          tunnel: [w1728] -> w1614
          frame #0 {
            n744 = call "mdrive send command.vi"("error in (no error)"=w1712, "Command"=T10."Stop", "VISA resource name"=w1710) -> ("error out"=w1711:errorcluster, "VISA resource name out"=w1709:refnum<visa-resource-name>)  [unwired: 4 in, 1 out]
          }
          frame #1 {
            n745 = Wait (ms)(milliseconds to wait=u32 50) -> ()  [unwired: 1 out]
          }
          frame #2 {
            n746 = call "mdrive send command.vi"("error in (no error)"=w1733, "Extra"="P", "Command"=T10."Print Parameter", "VISA resource name"=w1730) -> ("error out"=w1728:errorcluster, "read buffer"=w1723:string, "VISA resource name out"=w1729:refnum<visa-resource-name>)  [unwired: 3 in]
            n747 = property on="Y steps/rev" class="DigNum (strict)"() -> ("Value"=w1719:u32)  [unwired: 2 in, 2 out]
            n748 = Decimal String To Number(string=w1723, offset=0) -> (number=w1720:i32)  [unwired: 1 in, 1 out]
            n749 = property on="Y mm/rev" class="DigNum (strict)"() -> ("Value"=w1718:dbl)  [unwired: 2 in, 2 out]
            n750 = To Double Precision Float(number=w1720) -> (double precision float=w1725:dbl)
            n751 = To Double Precision Float(number=w1719) -> (double precision float=w1724:dbl)
            n752 = property on="Y offset mm" class="DigNum (strict)"() -> ("Value"=w1717:dbl)  [unwired: 2 in, 2 out]
            n753 = Divide(x=w1725, y=w1724) -> (x/y=w1727:dbl)
            n754 = property on="Y Step PV" class="DigNum (strict)"("Val(Sgnl)"=w1720) -> ()  [unwired: 2 in, 2 out]
            n755 = Multiply(x=w1727, y=w1718) -> (x*y=w1726:dbl)
            n756 = Add(x=w1726, y=w1717) -> (x+y=w1721:dbl)
            n757 = property on="Y Position mm PV" class="DigNum (strict)"("Val(Sgnl)"=w1721) -> ()  [unwired: 2 in, 2 out]
          }
        }
        n758 = flat-sequence {
          tunnel: w1630 -> [w1637]
          tunnel: [w1636] -> w1622
          tunnel: w1621 -> [w1635]
          tunnel: [w1634] -> w1619
          tunnel: [w1641] -> w1623
          tunnel: w1622 -> [w1641]
          tunnel: [w1640] -> w1620
          tunnel: w1619 -> [w1640]
          tunnel: w1623 -> [w1658]
          tunnel: w1620 -> [w1655]
          tunnel: [w1654] -> w1613
          tunnel: [w1653] -> w1612
          frame #0 {
            n759 = call "mdrive send command.vi"("error in (no error)"=w1637, "Command"=T10."Stop", "VISA resource name"=w1635) -> ("error out"=w1636:errorcluster, "VISA resource name out"=w1634:refnum<visa-resource-name>)  [unwired: 4 in, 1 out]
          }
          frame #1 {
            n760 = Wait (ms)(milliseconds to wait=u32 50) -> ()  [unwired: 1 out]
          }
          frame #2 {
            n761 = call "mdrive send command.vi"("error in (no error)"=w1658, "Extra"="P", "Command"=T10."Print Parameter", "VISA resource name"=w1655) -> ("error out"=w1653:errorcluster, "read buffer"=w1648:string, "VISA resource name out"=w1654:refnum<visa-resource-name>)  [unwired: 3 in]
            n762 = property on="R steps/rev" class="DigNum (strict)"() -> ("Value"=w1646:u32)  [unwired: 2 in, 2 out]
            n763 = Decimal String To Number(string=w1648, offset=0) -> (number=w1645:i32)  [unwired: 1 in, 1 out]
            n764 = property on="R deg/rev" class="DigNum (strict)"() -> ("Value"=w1644:dbl)  [unwired: 2 in, 2 out]
            n765 = property on="R Step PV" class="DigNum (strict)"("Val(Sgnl)"=w1645) -> ()  [unwired: 2 in, 2 out]
            n766 = To Double Precision Float(number=w1645) -> (double precision float=w1650:dbl)
            n767 = To Double Precision Float(number=w1646) -> (double precision float=w1649:dbl)
            n768 = property on="R offset deg" class="DigNum (strict)"() -> ("Value"=w1643:dbl)  [unwired: 2 in, 2 out]
            n769 = Divide(x=w1650, y=w1649) -> (x/y=w1652:dbl)
            n770 = Multiply(x=w1652, y=w1644) -> (x*y=w1651:dbl)
            n771 = Add(x=w1651, y=w1643) -> (x+y=w1642:dbl)
            n772 = property on="R Position deg PV" class="DigNum (strict)"("Val(Sgnl)"=w1642) -> ()  [unwired: 2 in, 2 out]
          }
        }
        n773 = property on="GO" class="Bool"("DisabledEnum"=T1."Enabled" ("Disabled")) -> ()  [unwired: 2 in, 2 out]
      }
      event #4 {
        n774 = event-data() -> ()  [unwired: 1 in, 5 out]
        n775 = local write "STATUS"("RESSETTING" ("STATUS")) -> ()
        n776 = property on="R offset deg" class="DigNum (strict)"() -> ("Value"=w1743:dbl)  [unwired: 2 in, 2 out]
        n777 = property on="Reset Z Position mm" class="DigNum (strict)"() -> ("Value"=w1760:dbl)  [unwired: 2 in, 2 out]
        n778 = property on="Z offset mm" class="DigNum (strict)"() -> ("Value"=w1752:dbl)  [unwired: 2 in, 2 out]
        n779 = property on="Reset R Position deg" class="DigNum (strict)"() -> ("Value"=w1751:dbl)  [unwired: 2 in, 2 out]
        n780 = property on="Reset X Position mm" class="DigNum (strict)"() -> ("Value"=w1769:dbl)  [unwired: 2 in, 2 out]
        n781 = property on="X offset mm" class="DigNum (strict)"() -> ("Value"=w1761:dbl)  [unwired: 2 in, 2 out]
        n782 = property on="Reset Y Position mm" class="DigNum (strict)"() -> ("Value"=w1778:dbl)  [unwired: 2 in, 2 out]
        n783 = property on="Y offset mm" class="DigNum (strict)"() -> ("Value"=w1770:dbl)  [unwired: 2 in, 2 out]
        n784 = Subtract(x=w1760, y=w1752) -> (x-y=w1759:dbl)
        n785 = Subtract(x=w1751, y=w1743) -> (x-y=w1750:dbl)
        n786 = Subtract(x=w1769, y=w1761) -> (x-y=w1768:dbl)
        n787 = Subtract(x=w1778, y=w1770) -> (x-y=w1777:dbl)
        n788 = property on="X mm/rev" class="DigNum (strict)"() -> ("Value"=w1762:dbl)  [unwired: 2 in, 2 out]
        n789 = property on="R deg/rev" class="DigNum (strict)"() -> ("Value"=w1744:dbl)  [unwired: 2 in, 2 out]
        n790 = property on="Y mm/rev" class="DigNum (strict)"() -> ("Value"=w1771:dbl)  [unwired: 2 in, 2 out]
        n791 = property on="Z mm/rev" class="DigNum (strict)"() -> ("Value"=w1753:dbl)  [unwired: 2 in, 2 out]
        n792 = Divide(x=w1750, y=w1744) -> (x/y=w1749:dbl)
        n793 = Divide(x=w1768, y=w1762) -> (x/y=w1767:dbl)
        n794 = Divide(x=w1777, y=w1771) -> (x/y=w1776:dbl)
        n795 = Divide(x=w1759, y=w1753) -> (x/y=w1758:dbl)
        n796 = property on="R steps/rev" class="DigNum (strict)"() -> ("Value"=w1745:u32)  [unwired: 2 in, 2 out]
        n797 = property on="Z steps/rev" class="DigNum (strict)"() -> ("Value"=w1754:u32)  [unwired: 2 in, 2 out]
        n798 = property on="X steps/rev" class="DigNum (strict)"() -> ("Value"=w1763:u32)  [unwired: 2 in, 2 out]
        n799 = property on="Y steps/rev" class="DigNum (strict)"() -> ("Value"=w1772:u32)  [unwired: 2 in, 2 out]
        n800 = To Double Precision Float(number=w1754) -> (double precision float=w1757:dbl)
        n801 = To Double Precision Float(number=w1745) -> (double precision float=w1748:dbl)
        n802 = To Double Precision Float(number=w1763) -> (double precision float=w1766:dbl)
        n803 = To Double Precision Float(number=w1772) -> (double precision float=w1775:dbl)
        n804 = Multiply(x=w1758, y=w1757) -> (x*y=w1756:dbl)
        n805 = Multiply(x=w1749, y=w1748) -> (x*y=w1747:dbl)
        n806 = Multiply(x=w1767, y=w1766) -> (x*y=w1765:dbl)
        n807 = Multiply(x=w1776, y=w1775) -> (x*y=w1774:dbl)
        n808 = To Long Integer(number=w1756) -> (32bit integer=w1755:i32)
        n809 = To Long Integer(number=w1747) -> (32bit integer=w1746:i32)
        n810 = To Long Integer(number=w1765) -> (32bit integer=w1764:i32)
        n811 = To Long Integer(number=w1774) -> (32bit integer=w1773:i32)
        n812 = property on="Reset Z Motor Steps" class="DigNum (strict)"("Val(Sgnl)"=w1755) -> ()  [unwired: 2 in, 2 out]
        n813 = property on="Reset R Motor Steps" class="DigNum (strict)"("Val(Sgnl)"=w1746) -> ()  [unwired: 2 in, 2 out]
        n814 = property on="Reset X Motor Steps" class="DigNum (strict)"("Val(Sgnl)"=w1764) -> ()  [unwired: 2 in, 2 out]
        n815 = property on="Reset Y Motor Steps" class="DigNum (strict)"("Val(Sgnl)"=w1773) -> ()  [unwired: 2 in, 2 out]
      }
      event #5 {
        n816 = event-data() -> ()  [unwired: 1 in, 5 out]
        n817 = property on="Y steps/rev" class="DigNum (strict)"() -> ("Value"=w1842:u32)  [unwired: 2 in, 2 out]
        n818 = property on="Y Step SP" class="DigNum (strict)"() -> ("Value"=w1819:i32)  [unwired: 2 in, 2 out]
        n819 = property on="Y steps/rev" class="DigNum (strict)"() -> ("Value"=w1817:u32)  [unwired: 2 in, 2 out]
        n820 = property on="Y Velocity SP step/sec" class="DigNum (strict)"() -> ("Value"=w1844:i32)  [unwired: 2 in, 2 out]
        n821 = property on="Y mm/rev" class="DigNum (strict)"() -> ("Value"=w1788:dbl)  [unwired: 2 in, 2 out]
        n822 = property on="Y offset mm" class="DigNum (strict)"() -> ("Value"=w1816:dbl)  [unwired: 2 in, 2 out]
        n823 = To Double Precision Float(number=w1819) -> (double precision float=w1820:dbl)
        n824 = To Double Precision Float(number=w1817) -> (double precision float=w1823:dbl)
        n825 = To Double Precision Float(number=w1844) -> (double precision float=w1845:dbl)
        n826 = To Double Precision Float(number=w1842) -> (double precision float=w1847:dbl)
        n827 = Divide(x=w1820, y=w1823) -> (x/y=w1822:dbl)
        n828 = Divide(x=w1845, y=w1847) -> (x/y=w1846:dbl)
        n829 = Multiply(x=w1822, y=w1788) -> (x*y=w1821:dbl)
        n830 = Multiply(x=w1846, y=w1788) -> (x*y=w1843:dbl)
        n831 = Add(x=w1821, y=w1816) -> (x+y=w1818:dbl)
        n832 = property on="Y Velocity MV mm/sec" class="DigNum (strict)"("Val(Sgnl)"=w1843) -> ()  [unwired: 2 in, 2 out]
        n833 = property on="Y Position MV mm" class="DigNum (strict)"("Val(Sgnl)"=w1818) -> ()  [unwired: 2 in, 2 out]
        n834 = property on="Z steps/rev" class="DigNum (strict)"() -> ("Value"=w1830:u32)  [unwired: 2 in, 2 out]
        n835 = property on="Z Step SP" class="DigNum (strict)"() -> ("Value"=w1803:i32)  [unwired: 2 in, 2 out]
        n836 = property on="Z steps/rev" class="DigNum (strict)"() -> ("Value"=w1801:u32)  [unwired: 2 in, 2 out]
        n837 = property on="Z Velocity SP step/sec" class="DigNum (strict)"() -> ("Value"=w1832:i32)  [unwired: 2 in, 2 out]
        n838 = property on="Z mm/rev" class="DigNum (strict)"() -> ("Value"=w1790:dbl)  [unwired: 2 in, 2 out]
        n839 = property on="Z offset mm" class="DigNum (strict)"() -> ("Value"=w1800:dbl)  [unwired: 2 in, 2 out]
        n840 = To Double Precision Float(number=w1832) -> (double precision float=w1833:dbl)
        n841 = To Double Precision Float(number=w1830) -> (double precision float=w1835:dbl)
        n842 = To Double Precision Float(number=w1803) -> (double precision float=w1804:dbl)
        n843 = To Double Precision Float(number=w1801) -> (double precision float=w1807:dbl)
        n844 = Divide(x=w1804, y=w1807) -> (x/y=w1806:dbl)
        n845 = Divide(x=w1833, y=w1835) -> (x/y=w1834:dbl)
        n846 = Multiply(x=w1806, y=w1790) -> (x*y=w1805:dbl)
        n847 = Multiply(x=w1834, y=w1790) -> (x*y=w1831:dbl)
        n848 = Add(x=w1805, y=w1800) -> (x+y=w1802:dbl)
        n849 = property on="Z Velocity MV mm/sec" class="DigNum (strict)"("Val(Sgnl)"=w1831) -> ()  [unwired: 2 in, 2 out]
        n850 = property on="Z Position MV mm" class="DigNum (strict)"("Val(Sgnl)"=w1802) -> ()  [unwired: 2 in, 2 out]
        n851 = property on="X Velocity SP step/sec" class="DigNum (strict)"() -> ("Value"=w1838:i32)  [unwired: 2 in, 2 out]
        n852 = property on="X steps/rev" class="DigNum (strict)"() -> ("Value"=w1836:u32)  [unwired: 2 in, 2 out]
        n853 = property on="X Step SP" class="DigNum (strict)"() -> ("Value"=w1811:i32)  [unwired: 2 in, 2 out]
        n854 = property on="X steps/rev" class="DigNum (strict)"() -> ("Value"=w1809:u32)  [unwired: 2 in, 2 out]
        n855 = property on="X offset mm" class="DigNum (strict)"() -> ("Value"=w1808:dbl)  [unwired: 2 in, 2 out]
        n856 = property on="X mm/rev" class="DigNum (strict)"() -> ("Value"=w1789:dbl)  [unwired: 2 in, 2 out]
        n857 = To Double Precision Float(number=w1811) -> (double precision float=w1812:dbl)
        n858 = To Double Precision Float(number=w1809) -> (double precision float=w1815:dbl)
        n859 = To Double Precision Float(number=w1838) -> (double precision float=w1839:dbl)
        n860 = To Double Precision Float(number=w1836) -> (double precision float=w1841:dbl)
        n861 = Divide(x=w1812, y=w1815) -> (x/y=w1814:dbl)
        n862 = Divide(x=w1839, y=w1841) -> (x/y=w1840:dbl)
        n863 = Multiply(x=w1814, y=w1789) -> (x*y=w1813:dbl)
        n864 = Add(x=w1813, y=w1808) -> (x+y=w1810:dbl)
        n865 = Multiply(x=w1840, y=w1789) -> (x*y=w1837:dbl)
        n866 = property on="X Velocity MV mm/sec" class="DigNum (strict)"("Val(Sgnl)"=w1837) -> ()  [unwired: 2 in, 2 out]
        n867 = property on="X Position MV mm" class="DigNum (strict)"("Val(Sgnl)"=w1810) -> ()  [unwired: 2 in, 2 out]
        n868 = property on="R steps/rev" class="DigNum (strict)"() -> ("Value"=w1824:u32)  [unwired: 2 in, 2 out]
        n869 = property on="R Step SP" class="DigNum (strict)"() -> ("Value"=w1795:i32)  [unwired: 2 in, 2 out]
        n870 = property on="R steps/rev" class="DigNum (strict)"() -> ("Value"=w1793:u32)  [unwired: 2 in, 2 out]
        n871 = property on="R deg/rev" class="DigNum (strict)"() -> ("Value"=w1791:dbl)  [unwired: 2 in, 2 out]
        n872 = property on="R offset deg" class="DigNum (strict)"() -> ("Value"=w1792:dbl)  [unwired: 2 in, 2 out]
        n873 = property on="R Velocity SP step/sec" class="DigNum (strict)"() -> ("Value"=w1826:i32)  [unwired: 2 in, 2 out]
        n874 = To Double Precision Float(number=w1795) -> (double precision float=w1796:dbl)
        n875 = To Double Precision Float(number=w1793) -> (double precision float=w1799:dbl)
        n876 = To Double Precision Float(number=w1824) -> (double precision float=w1829:dbl)
        n877 = To Double Precision Float(number=w1826) -> (double precision float=w1827:dbl)
        n878 = Divide(x=w1796, y=w1799) -> (x/y=w1798:dbl)
        n879 = Divide(x=w1827, y=w1829) -> (x/y=w1828:dbl)
        n880 = Multiply(x=w1798, y=w1791) -> (x*y=w1797:dbl)
        n881 = Multiply(x=w1828, y=w1791) -> (x*y=w1825:dbl)
        n882 = Add(x=w1797, y=w1792) -> (x+y=w1794:dbl)
        n883 = Absolute Value(x=w1825) -> (abs(x)=w1787:dbl)
        n884 = property on="R Position MV deg" class="DigNum (strict)"("Val(Sgnl)"=w1794) -> ()  [unwired: 2 in, 2 out]
        n885 = property on="R Velocity MVdeg/sec" class="DigNum (strict)"("Val(Sgnl)"=w1787) -> ()  [unwired: 2 in, 2 out]
      }
      event #6 {
        n886 = event-data() -> ()  [unwired: 1 in, 5 out]
        n887 = property on="R Step PV" class="DigNum (strict)"() -> ("Value"=w1888:i32)  [unwired: 2 in, 2 out]
        n888 = property on="R Step SP" class="DigNum (strict)"() -> ("Maximum"=w1896:dbl)  [unwired: 2 in, 2 out]
        n889 = property on="R Step SP" class="DigNum (strict)"() -> ("Minimum"=w1893:dbl)  [unwired: 2 in, 2 out]
        n890 = property on="X Step PV" class="DigNum (strict)"() -> ("Value"=w1928:i32)  [unwired: 2 in, 2 out]
        n891 = property on="Z Step PV" class="DigNum (strict)"() -> ("Value"=w1902:i32)  [unwired: 2 in, 2 out]
        n892 = property on="Z Step SP" class="DigNum (strict)"() -> ("Minimum"=w1909:dbl)  [unwired: 2 in, 2 out]
        n893 = property on="Z Step SP" class="DigNum (strict)"() -> ("Maximum"=w1908:dbl)  [unwired: 2 in, 2 out]
        n894 = property on="X Step SP" class="DigNum (strict)"() -> ("Maximum"=w1932:dbl)  [unwired: 2 in, 2 out]
        n895 = property on="Y Step SP" class="DigNum (strict)"() -> ("Minimum"=w1922:dbl)  [unwired: 2 in, 2 out]
        n896 = property on="Y Step SP" class="DigNum (strict)"() -> ("Maximum"=w1921:dbl)  [unwired: 2 in, 2 out]
        n897 = property on="X Step SP" class="DigNum (strict)"() -> ("Minimum"=w1933:dbl)  [unwired: 2 in, 2 out]
        n898 = property on="Y Step PV" class="DigNum (strict)"() -> ("Value"=w1915:i32)  [unwired: 2 in, 2 out]
        n899 = To Double Precision Float(number=w1888) -> (double precision float=w1879:dbl)
        n900 = To Double Precision Float(number=w1928) -> (double precision float=w1882:dbl)
        n901 = To Double Precision Float(number=w1902) -> (double precision float=w1880:dbl)
        n902 = To Double Precision Float(number=w1915) -> (double precision float=w1881:dbl)
        n903 = Subtract(x=w1893, y=w1879) -> (x-y=w1894:dbl)
        n904 = Subtract(x=w1896, y=w1879) -> (x-y=w1895:dbl)
        n905 = Subtract(x=w1922, y=w1881) -> (x-y=w1923:dbl)
        n906 = Subtract(x=w1921, y=w1881) -> (x-y=w1920:dbl)
        n907 = Subtract(x=w1933, y=w1882) -> (x-y=w1934:dbl)
        n908 = Subtract(x=w1932, y=w1882) -> (x-y=w1931:dbl)
        n909 = Subtract(x=w1909, y=w1880) -> (x-y=w1910:dbl)
        n910 = Subtract(x=w1908, y=w1880) -> (x-y=w1907:dbl)
        n911 = property on="R Scan Length SP steps" class="DigNum (strict)"("Minimum"=w1894) -> ()  [unwired: 2 in, 2 out]
        n912 = property on="R Scan Length SP steps" class="DigNum (strict)"("Maximum"=w1895) -> ()  [unwired: 2 in, 2 out]
        n913 = property on="Y Scan Length SP steps" class="DigNum (strict)"("Minimum"=w1923) -> ()  [unwired: 2 in, 2 out]
        n914 = property on="Y Scan Length SP steps" class="DigNum (strict)"("Maximum"=w1920) -> ()  [unwired: 2 in, 2 out]
        n915 = property on="X Scan Length SP steps" class="DigNum (strict)"("Minimum"=w1934) -> ()  [unwired: 2 in, 2 out]
        n916 = property on="X Scan Length SP steps" class="DigNum (strict)"("Maximum"=w1931) -> ()  [unwired: 2 in, 2 out]
        n917 = property on="Z Scan Length SP steps" class="DigNum (strict)"("Minimum"=w1910) -> ()  [unwired: 2 in, 2 out]
        n918 = property on="Z Scan Length SP steps" class="DigNum (strict)"("Maximum"=w1907) -> ()  [unwired: 2 in, 2 out]
        n919 = property on="X steps/rev" class="DigNum (strict)"() -> ("Value"=w1929:u32)  [unwired: 2 in, 2 out]
        n920 = property on="X Scan Length SP steps" class="DigNum (strict)"() -> ("Value"=w1926:i32)  [unwired: 2 in, 2 out]
        n921 = property on="X Scan Velocity SP steps/sec" class="DigNum (strict)"() -> ("Value"=w1930:i32)  [unwired: 2 in, 2 out]
        n922 = property on="Y steps/rev" class="DigNum (strict)"() -> ("Value"=w1917:u32)  [unwired: 2 in, 2 out]
        n923 = property on="R Scan Length SP steps" class="DigNum (strict)"() -> ("Value"=w1891:i32)  [unwired: 2 in, 2 out]
        n924 = property on="R steps/rev" class="DigNum (strict)"() -> ("Value"=w1890:u32)  [unwired: 2 in, 2 out]
        n925 = property on="R Scan Velocity SP steps/sec" class="DigNum (strict)"() -> ("Value"=w1886:i32)  [unwired: 2 in, 2 out]
        n926 = property on="Y Scan Length SP steps" class="DigNum (strict)"() -> ("Value"=w1918:i32)  [unwired: 2 in, 2 out]
        n927 = property on="Y Scan Velocity SP steps/sec" class="DigNum (strict)"() -> ("Value"=w1914:i32)  [unwired: 2 in, 2 out]
        n928 = property on="Z Scan Length SP steps" class="DigNum (strict)"() -> ("Value"=w1905:i32)  [unwired: 2 in, 2 out]
        n929 = property on="Z steps/rev" class="DigNum (strict)"() -> ("Value"=w1904:u32)  [unwired: 2 in, 2 out]
        n930 = property on="Z Scan Velocity SP steps/sec" class="DigNum (strict)"() -> ("Value"=w1900:i32)  [unwired: 2 in, 2 out]
        n931 = To Double Precision Float(number=w1926) -> (double precision float=w1869:dbl)
        n932 = To Double Precision Float(number=w1929) -> (double precision float=w1927:dbl)
        n933 = To Double Precision Float(number=w1930) -> (double precision float=w1868:dbl)
        n934 = To Double Precision Float(number=w1891) -> (double precision float=w1876:dbl)
        n935 = To Double Precision Float(number=w1890) -> (double precision float=w1887:dbl)
        n936 = To Double Precision Float(number=w1886) -> (double precision float=w1875:dbl)
        n937 = To Double Precision Float(number=w1905) -> (double precision float=w1878:dbl)
        n938 = To Double Precision Float(number=w1904) -> (double precision float=w1901:dbl)
        n939 = To Double Precision Float(number=w1900) -> (double precision float=w1877:dbl)
        n940 = To Double Precision Float(number=w1918) -> (double precision float=w1871:dbl)
        n941 = To Double Precision Float(number=w1917) -> (double precision float=w1872:dbl)
        n942 = To Double Precision Float(number=w1914) -> (double precision float=w1870:dbl)
        n943 = property on="R deg/rev" class="DigNum (strict)"() -> ("Value"=w1889:dbl)  [unwired: 2 in, 2 out]
        n944 = Divide(x=w1876, y=w1887) -> (x/y=w1892:dbl)
        n945 = property on="Z mm/rev" class="DigNum (strict)"() -> ("Value"=w1903:dbl)  [unwired: 2 in, 2 out]
        n946 = property on="X mm/rev" class="DigNum (strict)"() -> ("Value"=w1855:dbl)  [unwired: 2 in, 2 out]
        n947 = Divide(x=w1869, y=w1927) -> (x/y=w1856:dbl)
        n948 = Divide(x=w1878, y=w1901) -> (x/y=w1906:dbl)
        n949 = property on="Y mm/rev" class="DigNum (strict)"() -> ("Value"=w1916:dbl)  [unwired: 2 in, 2 out]
        n950 = Divide(x=w1871, y=w1872) -> (x/y=w1919:dbl)
        n951 = Divide(x=w1877, y=w1901) -> (x/y=w1899:dbl)
        n952 = Divide(x=w1875, y=w1887) -> (x/y=w1885:dbl)
        n953 = Multiply(x=w1906, y=w1903) -> (x*y=w1898:dbl)
        n954 = Divide(x=w1870, y=w1872) -> (x/y=w1913:dbl)
        n955 = Divide(x=w1868, y=w1927) -> (x/y=w1854:dbl)
        n956 = Multiply(x=w1856, y=w1855) -> (x*y=w1924:dbl)
        n957 = Divide(x=w1878, y=w1877) -> (x/y=w1873:dbl)
        n958 = Multiply(x=w1903, y=w1899) -> (x*y=w1897:dbl)
        n959 = Absolute Value(x=w1873) -> (abs(x)=→"Z Scan Duration":dbl)
        n960 = Multiply(x=w1919, y=w1916) -> (x*y=w1912:dbl)
        n961 = Multiply(x=w1916, y=w1913) -> (x*y=w1911:dbl)
        n962 = Multiply(x=w1855, y=w1854) -> (x*y=w1925:dbl)
        n963 = Divide(x=w1876, y=w1875) -> (x/y=w1874:dbl)
        n964 = Multiply(x=w1892, y=w1889) -> (x*y=w1884:dbl)
        n965 = Multiply(x=w1889, y=w1885) -> (x*y=w1883:dbl)
        n966 = Absolute Value(x=w1874) -> (abs(x)=→"R Scan Duration":dbl)
        n967 = Absolute Value(x=w1883) -> (abs(x)=w1867:dbl)
        n968 = property on="Z Scan length MV mm" class="DigNum (strict)"("Value"=w1898) -> ()  [unwired: 2 in, 2 out]
        n969 = property on="Z Scan velocity MV mm/sec" class="DigNum (strict)"("Val(Sgnl)"=w1897) -> ()  [unwired: 2 in, 2 out]
        n970 = property on="X Scan length MV mm" class="DigNum (strict)"("Val(Sgnl)"=w1924) -> ()  [unwired: 2 in, 2 out]
        n971 = property on="X Scan velocity MV mm/sec" class="DigNum (strict)"("Value"=w1925) -> ()  [unwired: 2 in, 2 out]
        n972 = property on="Y Scan length MV mm" class="DigNum (strict)"("Value"=w1912) -> ()  [unwired: 2 in, 2 out]
        n973 = property on="Y Scan velocity MV mm/sec" class="DigNum (strict)"("Val(Sgnl)"=w1911) -> ()  [unwired: 2 in, 2 out]
        n974 = property on="R Scan length MV deg" class="DigNum (strict)"("Value"=w1884) -> ()  [unwired: 2 in, 2 out]
        n975 = property on="R Scan Velocity SP deg/sec" class="DigNum (strict)"("Val(Sgnl)"=w1867) -> ()  [unwired: 2 in, 2 out]
        n976 = property on="Y Scan Length SP mm" class="DigNum (strict)"() -> ("Value"=w1851:dbl)  [unwired: 2 in, 2 out]
        n977 = property on="X Scan Length SP mm" class="DigNum (strict)"() -> ("Value"=w1850:dbl)  [unwired: 2 in, 2 out]
        n978 = Equal?(x=w1851, y=0.0) -> (x = y?=w1849:bool)
        n979 = Equal?(x=w1850, y=0.0) -> (x = y?=w1848:bool)
        n980 = case shown="True" w1849 {
          tunnel: w1871 -> [w1943 _]
          tunnel: w1870 -> [w1942 _]
          frame #0 {
            n981 = Divide(x=w1943, y=w1942) -> (x/y=w1941:dbl)
            n982 = Absolute Value(x=w1941) -> (abs(x)=→"Y Scan Duration":dbl)
          }
          frame #1 {
            n983 = local write "Y Scan Duration"(0.0 ("Y Scan Duration")) -> ()
          }
        }
        n984 = case shown="True" w1848 {
          tunnel: w1869 -> [w1937 _]
          tunnel: w1868 -> [w1936 _]
          frame #0 {
            n985 = Divide(x=w1937, y=w1936) -> (x/y=w1938:dbl)
            n986 = Absolute Value(x=w1938) -> (abs(x)=→"X Scan Duration":dbl)
          }
          frame #1 {
            n987 = local write "X Scan Duration"(0.0 ("X Scan Duration")) -> ()
          }
        }
      }
      event #7 {
        n988 = event-data() -> ()  [unwired: 1 in, 7 out]
        n989 = Wait (ms)(milliseconds to wait=u32 100) -> ()  [unwired: 1 out]
        n990 = local write "STATUS"("SETTING Y" ("STATUS")) -> ()
        n991 = property on="Y Position SP mm" class="DigNum (strict)"() -> ("Value"=w1968:dbl)  [unwired: 2 in, 2 out]
        n992 = property on="Y offset mm" class="DigNum (strict)"() -> ("Value"=w1969:dbl)  [unwired: 2 in, 2 out]
        n993 = property on="Y mm/rev" class="DigNum (strict)"() -> ("Value"=w1955:dbl)  [unwired: 2 in, 2 out]
        n994 = property on="Y Velocity SP mm/sec" class="DigNum (strict)"() -> ("Value"=w1962:dbl)  [unwired: 2 in, 2 out]
        n995 = property on="Y steps/rev" class="DigNum (strict)"() -> ("Value"=w1971:u32)  [unwired: 2 in, 2 out]
        n996 = Subtract(x=w1968, y=w1969) -> (x-y=w1972:dbl)
        n997 = Divide(x=w1962, y=w1955) -> (x/y=w1963:dbl)
        n998 = To Double Precision Float(number=w1971) -> (double precision float=w1956:dbl)
        n999 = Divide(x=w1972, y=w1955) -> (x/y=w1973:dbl)
        n1000 = Multiply(x=w1963, y=w1956) -> (x*y=w1960:dbl)
        n1001 = property on="Y Velocity SP step/sec" class="DigNum (strict)"() -> ("Maximum"=w1958:dbl)  [unwired: 2 in, 2 out]
        n1002 = property on="Y Velocity SP step/sec" class="DigNum (strict)"() -> ("Minimum"=w1957:dbl)  [unwired: 2 in, 2 out]
        n1003 = Multiply(x=w1973, y=w1956) -> (x*y=w1967:dbl)
        n1004 = In Range and Coerce(upper limit=w1958, x=w1960, lower limit=w1957) -> (coerced(x)=w1959:dbl)  [unwired: 1 out]
        n1005 = property on="Y Step SP" class="DigNum (strict)"() -> ("Maximum"=w1965:dbl)  [unwired: 2 in, 2 out]
        n1006 = property on="Y Step SP" class="DigNum (strict)"() -> ("Minimum"=w1964:dbl)  [unwired: 2 in, 2 out]
        n1007 = To Long Integer(number=w1959) -> (32bit integer=w1961:i32)
        n1008 = property on="Y Velocity SP step/sec" class="DigNum (strict)"("Val(Sgnl)"=w1961) -> ()  [unwired: 2 in, 2 out]
        n1009 = In Range and Coerce(upper limit=w1965, x=w1967, lower limit=w1964) -> (coerced(x)=w1966:dbl)  [unwired: 1 out]
        n1010 = To Long Integer(number=w1966) -> (32bit integer=w1970:i32)
        n1011 = property on="Y Step SP" class="DigNum (strict)"("Val(Sgnl)"=w1970) -> ()  [unwired: 2 in, 2 out]
      }
      event #8 {
        n1012 = event-data() -> ()  [unwired: 1 in, 7 out]
        n1013 = Wait (ms)(milliseconds to wait=u32 100) -> ()  [unwired: 1 out]
        n1014 = property on="X Position SP mm" class="DigNum (strict)"() -> ("Value"=w1997:dbl)  [unwired: 2 in, 2 out]
        n1015 = property on="X offset mm" class="DigNum (strict)"() -> ("Value"=w1998:dbl)  [unwired: 2 in, 2 out]
        n1016 = property on="X steps/rev" class="DigNum (strict)"() -> ("Value"=w2000:u32)  [unwired: 2 in, 2 out]
        n1017 = property on="X Velocity SP mm/sec" class="DigNum (strict)"() -> ("Value"=w1991:dbl)  [unwired: 2 in, 2 out]
        n1018 = property on="X mm/rev" class="DigNum (strict)"() -> ("Value"=w1984:dbl)  [unwired: 2 in, 2 out]
        n1019 = Subtract(x=w1997, y=w1998) -> (x-y=w2001:dbl)
        n1020 = Divide(x=w1991, y=w1984) -> (x/y=w1992:dbl)
        n1021 = To Double Precision Float(number=w2000) -> (double precision float=w1985:dbl)
        n1022 = local write "STATUS"("SETTING X" ("STATUS")) -> ()
        n1023 = Divide(x=w2001, y=w1984) -> (x/y=w2002:dbl)
        n1024 = Multiply(x=w1992, y=w1985) -> (x*y=w1989:dbl)
        n1025 = property on="X Velocity SP step/sec" class="DigNum (strict)"() -> ("Maximum"=w1987:dbl)  [unwired: 2 in, 2 out]
        n1026 = property on="X Velocity SP step/sec" class="DigNum (strict)"() -> ("Minimum"=w1986:dbl)  [unwired: 2 in, 2 out]
        n1027 = Multiply(x=w2002, y=w1985) -> (x*y=w1996:dbl)
        n1028 = property on="X Step SP" class="DigNum (strict)"() -> ("Maximum"=w1994:dbl)  [unwired: 2 in, 2 out]
        n1029 = property on="X Step SP" class="DigNum (strict)"() -> ("Minimum"=w1993:dbl)  [unwired: 2 in, 2 out]
        n1030 = In Range and Coerce(upper limit=w1987, x=w1989, lower limit=w1986) -> (coerced(x)=w1988:dbl)  [unwired: 1 out]
        n1031 = To Long Integer(number=w1988) -> (32bit integer=w1990:i32)
        n1032 = In Range and Coerce(upper limit=w1994, x=w1996, lower limit=w1993) -> (coerced(x)=w1995:dbl)  [unwired: 1 out]
        n1033 = property on="X Velocity SP step/sec" class="DigNum (strict)"("Val(Sgnl)"=w1990) -> ()  [unwired: 2 in, 2 out]
        n1034 = To Long Integer(number=w1995) -> (32bit integer=w1999:i32)
        n1035 = property on="X Step SP" class="DigNum (strict)"("Val(Sgnl)"=w1999) -> ()  [unwired: 2 in, 2 out]
      }
      event #9 {
        n1036 = event-data() -> ()  [unwired: 1 in, 7 out]
        n1037 = Wait (ms)(milliseconds to wait=u32 100) -> ()  [unwired: 1 out]
        n1038 = property on="Z mm/rev" class="DigNum (strict)"() -> ("Value"=w2030:dbl)  [unwired: 2 in, 2 out]
        n1039 = property on="Z steps/rev" class="DigNum (strict)"() -> ("Value"=w2027:u32)  [unwired: 2 in, 2 out]
        n1040 = property on="Z Velocity SP mm/sec" class="DigNum (strict)"() -> ("Value"=w2018:dbl)  [unwired: 2 in, 2 out]
        n1041 = property on="Z Position SP mm" class="DigNum (strict)"() -> ("Value"=w2024:dbl)  [unwired: 2 in, 2 out]
        n1042 = property on="Z offset mm" class="DigNum (strict)"() -> ("Value"=w2025:dbl)  [unwired: 2 in, 2 out]
        n1043 = Divide(x=w2018, y=w2030) -> (x/y=w2019:dbl)
        n1044 = To Double Precision Float(number=w2027) -> (double precision float=w2031:dbl)
        n1045 = Subtract(x=w2024, y=w2025) -> (x-y=w2028:dbl)
        n1046 = Divide(x=w2028, y=w2030) -> (x/y=w2029:dbl)
        n1047 = Multiply(x=w2019, y=w2031) -> (x*y=w2016:dbl)
        n1048 = property on="Z Velocity SP step/sec" class="DigNum (strict)"() -> ("Maximum"=w2014:dbl)  [unwired: 2 in, 2 out]
        n1049 = property on="Z Velocity SP step/sec" class="DigNum (strict)"() -> ("Minimum"=w2013:dbl)  [unwired: 2 in, 2 out]
        n1050 = local write "STATUS"("SETTING Z" ("STATUS")) -> ()
        n1051 = Multiply(x=w2029, y=w2031) -> (x*y=w2023:dbl)
        n1052 = In Range and Coerce(upper limit=w2014, x=w2016, lower limit=w2013) -> (coerced(x)=w2015:dbl)  [unwired: 1 out]
        n1053 = property on="Z Step SP" class="DigNum (strict)"() -> ("Maximum"=w2021:dbl)  [unwired: 2 in, 2 out]
        n1054 = property on="Z Step SP" class="DigNum (strict)"() -> ("Minimum"=w2020:dbl)  [unwired: 2 in, 2 out]
        n1055 = To Long Integer(number=w2015) -> (32bit integer=w2017:i32)
        n1056 = property on="Z Velocity SP step/sec" class="DigNum (strict)"("Val(Sgnl)"=w2017) -> ()  [unwired: 2 in, 2 out]
        n1057 = In Range and Coerce(upper limit=w2021, x=w2023, lower limit=w2020) -> (coerced(x)=w2022:dbl)  [unwired: 1 out]
        n1058 = To Long Integer(number=w2022) -> (32bit integer=w2026:i32)
        n1059 = property on="Z Step SP" class="DigNum (strict)"("Val(Sgnl)"=w2026) -> ()  [unwired: 2 in, 2 out]
      }
      event #10 {
        n1060 = event-data() -> ()  [unwired: 1 in, 7 out]
        n1061 = property on="R offset deg" class="DigNum (strict)"() -> ("Value"=w2057:dbl)  [unwired: 2 in, 2 out]
        n1062 = property on="R Position SP deg" class="DigNum (strict)"() -> ("Value"=w2056:dbl)  [unwired: 2 in, 2 out]
        n1063 = Wait (ms)(milliseconds to wait=u32 100) -> ()  [unwired: 1 out]
        n1064 = Subtract(x=w2056, y=w2057) -> (x-y=w2060:dbl)
        n1065 = property on="R deg/rev" class="DigNum (strict)"() -> ("Value"=w2043:dbl)  [unwired: 2 in, 2 out]
        n1066 = property on="R Velocity SP deg/sec" class="DigNum (strict)"() -> ("Value"=w2050:dbl)  [unwired: 2 in, 2 out]
        n1067 = Divide(x=w2060, y=w2043) -> (x/y=w2061:dbl)
        n1068 = property on="R steps/rev" class="DigNum (strict)"() -> ("Value"=w2059:u32)  [unwired: 2 in, 2 out]
        n1069 = Divide(x=w2050, y=w2043) -> (x/y=w2051:dbl)
        n1070 = To Double Precision Float(number=w2059) -> (double precision float=w2044:dbl)
        n1071 = Multiply(x=w2051, y=w2044) -> (x*y=w2048:dbl)
        n1072 = Multiply(x=w2061, y=w2044) -> (x*y=w2055:dbl)
        n1073 = property on="R Velocity SP step/sec" class="DigNum (strict)"() -> ("Maximum"=w2046:dbl)  [unwired: 2 in, 2 out]
        n1074 = property on="R Step SP" class="DigNum (strict)"() -> ("Maximum"=w2053:dbl)  [unwired: 2 in, 2 out]
        n1075 = property on="R Step SP" class="DigNum (strict)"() -> ("Minimum"=w2052:dbl)  [unwired: 2 in, 2 out]
        n1076 = property on="R Velocity SP step/sec" class="DigNum (strict)"() -> ("Minimum"=w2045:dbl)  [unwired: 2 in, 2 out]
        n1077 = Absolute Value(x=w2048) -> (abs(x)=w2042:dbl)
        n1078 = In Range and Coerce(upper limit=w2053, x=w2055, lower limit=w2052) -> (coerced(x)=w2054:dbl)  [unwired: 1 out]
        n1079 = In Range and Coerce(upper limit=w2046, x=w2042, lower limit=w2045) -> (coerced(x)=w2047:dbl)  [unwired: 1 out]
        n1080 = To Long Integer(number=w2054) -> (32bit integer=w2058:i32)
        n1081 = To Long Integer(number=w2047) -> (32bit integer=w2049:i32)
        n1082 = local write "STATUS"("SETTING R" ("STATUS")) -> ()
        n1083 = property on="R Step SP" class="DigNum (strict)"("Val(Sgnl)"=w2058) -> ()  [unwired: 2 in, 2 out]
        n1084 = property on="R Velocity SP step/sec" class="DigNum (strict)"("Val(Sgnl)"=w2049) -> ()  [unwired: 2 in, 2 out]
      }
      event #11 {
        n1085 = event-data() -> ()  [unwired: 1 in, 7 out]
        n1086 = flat-sequence {
          frame #0 {
            n1087 = property on="Y mm/rev" class="DigNum (strict)"() -> ("Value"=w2071:dbl)  [unwired: 2 in, 2 out]
            n1088 = property on="Z mm/rev" class="DigNum (strict)"() -> ("Value"=w2123:dbl)  [unwired: 2 in, 2 out]
            n1089 = property on="Z Scan Length SP mm" class="DigNum (strict)"() -> ("Value"=w2136:dbl)  [unwired: 2 in, 2 out]
            n1090 = property on="Y Scan Length SP mm" class="DigNum (strict)"() -> ("Value"=w2084:dbl)  [unwired: 2 in, 2 out]
            n1091 = property on="Y steps/rev" class="DigNum (strict)"() -> ("Value"=w2086:u32)  [unwired: 2 in, 2 out]
            n1092 = Divide(x=w2136, y=w2123) -> (x/y=w2139:dbl)
            n1093 = Divide(x=w2084, y=w2071) -> (x/y=w2087:dbl)
            n1094 = property on="Z steps/rev" class="DigNum (strict)"() -> ("Value"=w2138:u32)  [unwired: 2 in, 2 out]
            n1095 = To Double Precision Float(number=w2086) -> (double precision float=w2072:dbl)
            n1096 = To Double Precision Float(number=w2138) -> (double precision float=w2124:dbl)
            n1097 = Multiply(x=w2087, y=w2072) -> (x*y=w2083:dbl)
            n1098 = property on="Y Step SP" class="DigNum (strict)"() -> ("Minimum"=w2081:dbl)  [unwired: 2 in, 2 out]
            n1099 = property on="Y Step SP" class="DigNum (strict)"() -> ("Maximum"=w2080:dbl)  [unwired: 2 in, 2 out]
            n1100 = property on="Z Step SP" class="DigNum (strict)"() -> ("Maximum"=w2132:dbl)  [unwired: 2 in, 2 out]
            n1101 = property on="Z Step SP" class="DigNum (strict)"() -> ("Minimum"=w2133:dbl)  [unwired: 2 in, 2 out]
            n1102 = Multiply(x=w2139, y=w2124) -> (x*y=w2135:dbl)
            n1103 = In Range and Coerce(upper limit=w2080, x=w2083, lower limit=w2081) -> (coerced(x)=w2082:dbl)  [unwired: 1 out]
            n1104 = In Range and Coerce(upper limit=w2132, x=w2135, lower limit=w2133) -> (coerced(x)=w2134:dbl)  [unwired: 1 out]
            n1105 = To Long Integer(number=w2082) -> (32bit integer=w2085:i32)
            n1106 = property on="Y Scan Velocity SP mm/sec" class="DigNum (strict)"() -> ("Value"=w2078:dbl)  [unwired: 2 in, 2 out]
            n1107 = property on="Z Scan Velocity SP mm/sec" class="DigNum (strict)"() -> ("Value"=w2130:dbl)  [unwired: 2 in, 2 out]
            n1108 = To Long Integer(number=w2134) -> (32bit integer=w2137:i32)
            n1109 = Divide(x=w2078, y=w2071) -> (x/y=w2079:dbl)
            n1110 = property on="Y Scan Length SP steps" class="DigNum (strict)"("Val(Sgnl)"=w2085) -> ()  [unwired: 2 in, 2 out]
            n1111 = property on="Y Scan Velocity SP steps/sec" class="DigNum (strict)"() -> ("Maximum"=w2074:dbl)  [unwired: 2 in, 2 out]
            n1112 = property on="Z Scan Velocity SP steps/sec" class="DigNum (strict)"() -> ("Maximum"=w2126:dbl)  [unwired: 2 in, 2 out]
            n1113 = Divide(x=w2130, y=w2123) -> (x/y=w2131:dbl)
            n1114 = property on="Y Scan Velocity SP steps/sec" class="DigNum (strict)"() -> ("Minimum"=w2073:dbl)  [unwired: 2 in, 2 out]
            n1115 = property on="Z Scan Length SP steps" class="DigNum (strict)"("Val(Sgnl)"=w2137) -> ()  [unwired: 2 in, 2 out]
            n1116 = property on="Z Scan Velocity SP steps/sec" class="DigNum (strict)"() -> ("Minimum"=w2125:dbl)  [unwired: 2 in, 2 out]
            n1117 = Multiply(x=w2079, y=w2072) -> (x*y=w2076:dbl)
            n1118 = Multiply(x=w2131, y=w2124) -> (x*y=w2128:dbl)
            n1119 = In Range and Coerce(upper limit=w2074, x=w2076, lower limit=w2073) -> (coerced(x)=w2075:dbl)  [unwired: 1 out]
            n1120 = In Range and Coerce(upper limit=w2126, x=w2128, lower limit=w2125) -> (coerced(x)=w2127:dbl)  [unwired: 1 out]
            n1121 = To Long Integer(number=w2075) -> (32bit integer=w2077:i32)
            n1122 = To Long Integer(number=w2127) -> (32bit integer=w2129:i32)
            n1123 = property on="Y Scan Velocity SP steps/sec" class="DigNum (strict)"("Val(Sgnl)"=w2077) -> ()  [unwired: 2 in, 2 out]
            n1124 = property on="Z Scan Velocity SP steps/sec" class="DigNum (strict)"("Val(Sgnl)"=w2129) -> ()  [unwired: 2 in, 2 out]
            n1125 = property on="X mm/rev" class="DigNum (strict)"() -> ("Value"=w2106:dbl)  [unwired: 2 in, 2 out]
            n1126 = property on="X Scan Length SP mm" class="DigNum (strict)"() -> ("Value"=w2119:dbl)  [unwired: 2 in, 2 out]
            n1127 = property on="R deg/rev" class="DigNum (strict)"() -> ("Value"=w2089:dbl)  [unwired: 2 in, 2 out]
            n1128 = property on="R Scan Length SP deg" class="DigNum (strict)"() -> ("Value"=w2102:dbl)  [unwired: 2 in, 2 out]
            n1129 = Divide(x=w2102, y=w2089) -> (x/y=w2105:dbl)
            n1130 = Divide(x=w2119, y=w2106) -> (x/y=w2122:dbl)
            n1131 = property on="X steps/rev" class="DigNum (strict)"() -> ("Value"=w2121:u32)  [unwired: 2 in, 2 out]
            n1132 = property on="R steps/rev" class="DigNum (strict)"() -> ("Value"=w2104:u32)  [unwired: 2 in, 2 out]
            n1133 = To Double Precision Float(number=w2121) -> (double precision float=w2107:dbl)
            n1134 = To Double Precision Float(number=w2104) -> (double precision float=w2090:dbl)
            n1135 = property on="X Step SP" class="DigNum (strict)"() -> ("Minimum"=w2116:dbl)  [unwired: 2 in, 2 out]
            n1136 = property on="X Step SP" class="DigNum (strict)"() -> ("Maximum"=w2115:dbl)  [unwired: 2 in, 2 out]
            n1137 = Multiply(x=w2122, y=w2107) -> (x*y=w2118:dbl)
            n1138 = In Range and Coerce(upper limit=w2115, x=w2118, lower limit=w2116) -> (coerced(x)=w2117:dbl)  [unwired: 1 out]
            n1139 = property on="R Step SP" class="DigNum (strict)"() -> ("Maximum"=w2098:dbl)  [unwired: 2 in, 2 out]
            n1140 = property on="R Step SP" class="DigNum (strict)"() -> ("Minimum"=w2099:dbl)  [unwired: 2 in, 2 out]
            n1141 = Multiply(x=w2105, y=w2090) -> (x*y=w2101:dbl)
            n1142 = property on="X Scan Velocity SP mm/sec" class="DigNum (strict)"() -> ("Value"=w2113:dbl)  [unwired: 2 in, 2 out]
            n1143 = property on="R Scan Velocity SP deg/sec" class="DigNum (strict)"() -> ("Value"=w2096:dbl)  [unwired: 2 in, 2 out]
            n1144 = To Long Integer(number=w2117) -> (32bit integer=w2120:i32)
            n1145 = Divide(x=w2113, y=w2106) -> (x/y=w2114:dbl)
            n1146 = property on="X Scan Velocity SP steps/sec" class="DigNum (strict)"() -> ("Maximum"=w2109:dbl)  [unwired: 2 in, 2 out]
            n1147 = property on="X Scan Velocity SP steps/sec" class="DigNum (strict)"() -> ("Minimum"=w2108:dbl)  [unwired: 2 in, 2 out]
            n1148 = In Range and Coerce(upper limit=w2098, x=w2101, lower limit=w2099) -> (coerced(x)=w2100:dbl)  [unwired: 1 out]
            n1149 = Divide(x=w2096, y=w2089) -> (x/y=w2097:dbl)
            n1150 = property on="X Scan Length SP steps" class="DigNum (strict)"("Val(Sgnl)"=w2120) -> ()  [unwired: 2 in, 2 out]
            n1151 = Multiply(x=w2114, y=w2107) -> (x*y=w2111:dbl)
            n1152 = Multiply(x=w2097, y=w2090) -> (x*y=w2094:dbl)
            n1153 = To Long Integer(number=w2100) -> (32bit integer=w2103:i32)
            n1154 = property on="R Velocity SP step/sec" class="DigNum (strict)"() -> ("Maximum"=w2092:dbl)  [unwired: 2 in, 2 out]
            n1155 = property on="R Scan Velocity SP steps/sec" class="DigNum (strict)"() -> ("Minimum"=w2091:dbl)  [unwired: 2 in, 2 out]
            n1156 = Absolute Value(x=w2094) -> (abs(x)=w2088:dbl)
            n1157 = property on="R Scan Length SP steps" class="DigNum (strict)"("Val(Sgnl)"=w2103) -> ()  [unwired: 2 in, 2 out]
            n1158 = In Range and Coerce(upper limit=w2109, x=w2111, lower limit=w2108) -> (coerced(x)=w2110:dbl)  [unwired: 1 out]
            n1159 = In Range and Coerce(upper limit=w2092, x=w2088, lower limit=w2091) -> (coerced(x)=w2093:dbl)  [unwired: 1 out]
            n1160 = To Long Integer(number=w2110) -> (32bit integer=w2112:i32)
            n1161 = To Long Integer(number=w2093) -> (32bit integer=w2095:i32)
            n1162 = property on="X Scan Velocity SP steps/sec" class="DigNum (strict)"("Val(Sgnl)"=w2112) -> ()  [unwired: 2 in, 2 out]
            n1163 = property on="R Scan Velocity SP steps/sec" class="DigNum (strict)"("Val(Sgnl)"=w2095) -> ()  [unwired: 2 in, 2 out]
          }
          frame #1 {
            n1164 = case shown="True" "Z as dominating length" {
              frame #0 {
              }
              frame #1 {
                n1165 = property on="Y Scan Length SP steps" class="DigNum (strict)"() -> ("Value"=w2149:i32)  [unwired: 2 in, 2 out]
                n1166 = property on="Z Scan Length SP steps" class="DigNum (strict)"() -> ("Value"=w2148:i32)  [unwired: 2 in, 2 out]
                n1167 = property on="Y Scan Velocity SP steps/sec" class="DigNum (strict)"() -> ("Value"=w2145:i32)  [unwired: 2 in, 2 out]
                n1168 = property on="X Scan Length SP steps" class="DigNum (strict)"() -> ("Value"=w2157:i32)  [unwired: 2 in, 2 out]
                n1169 = property on="Z Scan Length SP steps" class="DigNum (strict)"() -> ("Value"=w2156:i32)  [unwired: 2 in, 2 out]
                n1170 = property on="X Scan Velocity SP steps/sec" class="DigNum (strict)"() -> ("Value"=w2155:i32)  [unwired: 2 in, 2 out]
                n1171 = To Double Precision Float(number=w2149) -> (double precision float=w2147:dbl)
                n1172 = To Double Precision Float(number=w2148) -> (double precision float=w2146:dbl)
                n1173 = To Double Precision Float(number=w2145) -> (double precision float=w2144:dbl)
                n1174 = To Double Precision Float(number=w2157) -> (double precision float=w2151:dbl)
                n1175 = To Double Precision Float(number=w2156) -> (double precision float=w2152:dbl)
                n1176 = To Double Precision Float(number=w2155) -> (double precision float=w2153:dbl)
                n1177 = Divide(x=w2147, y=w2146) -> (x/y=w2141:dbl)
                n1178 = Divide(x=w2151, y=w2152) -> (x/y=w2158:dbl)
                n1179 = Multiply(x=w2141, y=w2144) -> (x*y=w2143:dbl)
                n1180 = Multiply(x=w2158, y=w2153) -> (x*y=w2154:dbl)
                n1181 = To Long Integer(number=w2143) -> (32bit integer=w2142:i32)
                n1182 = To Long Integer(number=w2154) -> (32bit integer=w2150:i32)
                n1183 = property on="Y Scan Velocity SP steps/sec" class="DigNum (strict)"("Val(Sgnl)"=w2142) -> ()  [unwired: 2 in, 2 out]
                n1184 = property on="X Scan Velocity SP steps/sec" class="DigNum (strict)"("Val(Sgnl)"=w2150) -> ()  [unwired: 2 in, 2 out]
              }
            }
          }
        }
        n1185 = local write "STATUS"("SCANNING PARAMETERS SET" ("STATUS")) -> ()
      }
      event #12 {
        n1186 = event-data() -> ()  [unwired: 1 in, 7 out]
        n1187 = flat-sequence {
          tunnel: [w2308] -> w2206
          tunnel: [w2307] -> w2204
          tunnel: w2212 -> [w2310]
          tunnel: w2211 -> [w2309]
          tunnel: w2206 -> [w2316]
          tunnel: [w2316] -> w2205
          tunnel: w2204 -> [w2315]
          tunnel: [w2315] -> w2203
          tunnel: w2205 -> [w2320]
          tunnel: [w2319] -> w2208
          tunnel: w2203 -> [w2318]
          tunnel: [w2317] -> w2207
          tunnel: w2208 -> [w2328]
          tunnel: [w2328] -> w2210
          tunnel: w2207 -> [w2327]
          tunnel: [w2327] -> w2209
          tunnel: w2210 -> [w2333]
          tunnel: w2209 -> [w2332]
          tunnel: [w2333] -> w2214
          tunnel: [w2332] -> w2213
          tunnel: [w2335] -> w2215
          tunnel: [w2336] -> w2216
          tunnel: w2214 -> [w2336]
          tunnel: w2213 -> [w2335]
          frame #0 {
            n1188 = property on="X Scan Velocity SP steps/sec" class="DigNum (strict)"() -> ("Value"=w2312:i32)  [unwired: 2 in, 2 out]
            n1189 = Number To Decimal String(number=w2312) -> (decimal integer string=w2313:string)  [unwired: 1 in]
            n1190 = call "mdrive send command.vi"("error in (no error)"=w2310, "Extra"=w2313, "Command"=T10."Max Velocity", "VISA resource name"=w2309) -> ("error out"=w2307:errorcluster, "VISA resource name out"=w2308:refnum<visa-resource-name>)  [unwired: 3 in, 1 out]
          }
          frame #1 {
            n1191 = Wait (ms)(milliseconds to wait=u32 100) -> ()  [unwired: 1 out]
          }
          frame #2 {
            # "VELOCITY"
            n1192 = call "mdrive send command.vi"("error in (no error)"=w2318, "Extra"="VM", "Command"=T10."Print Parameter", "VISA resource name"=w2320) -> ("error out"=w2317:errorcluster, "read buffer"=w2323:string, "VISA resource name out"=w2319:refnum<visa-resource-name>)  [unwired: 3 in]
            n1193 = Decimal String To Number(string=w2323, offset=0) -> (number=w2321:i32)  [unwired: 1 in, 1 out]
            n1194 = property on="X velocity PV step/sec" class="DigNum (strict)"("Val(Sgnl)"=w2321) -> ()  [unwired: 2 in, 2 out]
          }
          frame #3 {
            n1195 = Wait (ms)(milliseconds to wait=u32 100) -> ()  [unwired: 1 out]
          }
          frame #4 {
            n1196 = property on="X Scan Velocity SP steps/sec" class="DigNum (strict)"("DisabledEnum"=T1."Disabled and Grayed Out" ("Disabled")) -> ()  [unwired: 2 in, 2 out]
            n1197 = property on="X Scan Length SP steps" class="DigNum (strict)"("DisabledEnum"=T1."Disabled and Grayed Out" ("Disabled")) -> ()  [unwired: 2 in, 2 out]
            n1198 = property on="Scan Go" class="Bool (strict)"("DisabledEnum"=T1."Enabled" ("Disabled")) -> ()  [unwired: 2 in, 2 out]
          }
          frame #5 {
            n1199 = property on="X Scan" class="Bool (strict)"("Val(Sgnl)"=TRUE ("Slew Ready 2")) -> ()  [unwired: 2 in, 2 out]
          }
        }
        n1200 = flat-sequence {
          tunnel: [w2250] -> w2188
          tunnel: [w2249] -> w2187
          tunnel: w2178 -> [w2248]
          tunnel: w2177 -> [w2247]
          tunnel: w2188 -> [w2256]
          tunnel: [w2256] -> w2186
          tunnel: w2187 -> [w2255]
          tunnel: [w2255] -> w2185
          tunnel: w2186 -> [w2262]
          tunnel: [w2261] -> w2184
          tunnel: w2185 -> [w2260]
          tunnel: [w2259] -> w2183
          tunnel: w2184 -> [w2268]
          tunnel: [w2268] -> w2182
          tunnel: w2183 -> [w2267]
          tunnel: [w2267] -> w2181
          tunnel: w2182 -> [w2273]
          tunnel: w2181 -> [w2272]
          tunnel: [w2273] -> w2180
          tunnel: [w2272] -> w2179
          tunnel: [w2275] -> w2175
          tunnel: [w2276] -> w2176
          tunnel: w2180 -> [w2276]
          tunnel: w2179 -> [w2275]
          frame #0 {
            n1201 = property on="Z Scan Velocity SP steps/sec" class="DigNum (strict)"() -> ("Value"=w2252:i32)  [unwired: 2 in, 2 out]
            n1202 = Number To Decimal String(number=w2252) -> (decimal integer string=w2253:string)  [unwired: 1 in]
            n1203 = call "mdrive send command.vi"("error in (no error)"=w2248, "Extra"=w2253, "Command"=T10."Max Velocity", "VISA resource name"=w2247) -> ("error out"=w2249:errorcluster, "VISA resource name out"=w2250:refnum<visa-resource-name>)  [unwired: 3 in, 1 out]
          }
          frame #1 {
            n1204 = Wait (ms)(milliseconds to wait=u32 100) -> ()  [unwired: 1 out]
          }
          frame #2 {
            # "VELOCITY"
            n1205 = call "mdrive send command.vi"("error in (no error)"=w2260, "Extra"="VM", "Command"=T10."Print Parameter", "VISA resource name"=w2262) -> ("error out"=w2259:errorcluster, "read buffer"=w2263:string, "VISA resource name out"=w2261:refnum<visa-resource-name>)  [unwired: 3 in]
            n1206 = Decimal String To Number(string=w2263, offset=0) -> (number=w2264:i32)  [unwired: 1 in, 1 out]
            n1207 = property on="Z  velocity PV step/sec" class="DigNum (strict)"("Val(Sgnl)"=w2264) -> ()  [unwired: 2 in, 2 out]
          }
          frame #3 {
            n1208 = Wait (ms)(milliseconds to wait=u32 100) -> ()  [unwired: 1 out]
          }
          frame #4 {
            n1209 = property on="Z Scan Length SP steps" class="DigNum (strict)"("DisabledEnum"=T1."Disabled and Grayed Out" ("Disabled")) -> ()  [unwired: 2 in, 2 out]
            n1210 = property on="Z Scan Velocity SP steps/sec" class="DigNum (strict)"("DisabledEnum"=T1."Disabled and Grayed Out" ("Disabled")) -> ()  [unwired: 2 in, 2 out]
            n1211 = property on="Scan Go" class="Bool (strict)"("DisabledEnum"=T1."Enabled" ("Disabled")) -> ()  [unwired: 2 in, 2 out]
          }
          frame #5 {
            n1212 = property on="Z Scan" class="Bool (strict)"("Val(Sgnl)"=TRUE ("Slew Ready 2")) -> ()  [unwired: 2 in, 2 out]
          }
        }
        n1213 = flat-sequence {
          tunnel: [w2280] -> w2202
          tunnel: [w2279] -> w2201
          tunnel: w2191 -> [w2278]
          tunnel: w2190 -> [w2277]
          tunnel: w2202 -> [w2286]
          tunnel: [w2286] -> w2200
          tunnel: w2201 -> [w2285]
          tunnel: [w2285] -> w2199
          tunnel: w2200 -> [w2290]
          tunnel: [w2289] -> w2198
          tunnel: w2199 -> [w2288]
          tunnel: [w2287] -> w2197
          tunnel: w2198 -> [w2298]
          tunnel: [w2298] -> w2196
          tunnel: w2197 -> [w2297]
          tunnel: [w2297] -> w2195
          tunnel: w2196 -> [w2303]
          tunnel: w2195 -> [w2302]
          tunnel: [w2303] -> w2194
          tunnel: [w2302] -> w2193
          tunnel: [w2305] -> w2192
          tunnel: [w2306] -> w2189
          tunnel: w2194 -> [w2306]
          tunnel: w2193 -> [w2305]
          frame #0 {
            n1214 = property on="Y Scan Velocity SP steps/sec" class="DigNum (strict)"() -> ("Value"=w2282:i32)  [unwired: 2 in, 2 out]
            n1215 = Number To Decimal String(number=w2282) -> (decimal integer string=w2283:string)  [unwired: 1 in]
            n1216 = call "mdrive send command.vi"("error in (no error)"=w2278, "Extra"=w2283, "Command"=T10."Max Velocity", "VISA resource name"=w2277) -> ("error out"=w2279:errorcluster, "VISA resource name out"=w2280:refnum<visa-resource-name>)  [unwired: 3 in, 1 out]
          }
          frame #1 {
            n1217 = Wait (ms)(milliseconds to wait=u32 100) -> ()  [unwired: 1 out]
          }
          frame #2 {
            # "VELOCITY"
            n1218 = call "mdrive send command.vi"("error in (no error)"=w2288, "Extra"="VM", "Command"=T10."Print Parameter", "VISA resource name"=w2290) -> ("error out"=w2287:errorcluster, "read buffer"=w2294:string, "VISA resource name out"=w2289:refnum<visa-resource-name>)  [unwired: 3 in]
            n1219 = Decimal String To Number(string=w2294, offset=0) -> (number=w2292:i32)  [unwired: 1 in, 1 out]
            n1220 = property on="Y velocity PV step/sec" class="DigNum (strict)"("Val(Sgnl)"=w2292) -> ()  [unwired: 2 in, 2 out]
          }
          frame #3 {
            n1221 = Wait (ms)(milliseconds to wait=u32 100) -> ()  [unwired: 1 out]
          }
          frame #4 {
            n1222 = property on="Y Scan Velocity SP steps/sec" class="DigNum (strict)"("DisabledEnum"=T1."Disabled and Grayed Out" ("Disabled")) -> ()  [unwired: 2 in, 2 out]
            n1223 = property on="Y Scan Length SP steps" class="DigNum (strict)"("DisabledEnum"=T1."Disabled and Grayed Out" ("Disabled")) -> ()  [unwired: 2 in, 2 out]
            n1224 = property on="Scan Go" class="Bool (strict)"("DisabledEnum"=T1."Enabled" ("Disabled")) -> ()  [unwired: 2 in, 2 out]
          }
          frame #5 {
            n1225 = property on="Y Scan" class="Bool (strict)"("Val(Sgnl)"=TRUE ("Slew Ready 2")) -> ()  [unwired: 2 in, 2 out]
          }
        }
        n1226 = flat-sequence {
          tunnel: [w2220] -> w2174
          tunnel: [w2219] -> w2173
          tunnel: w2164 -> [w2218]
          tunnel: w2163 -> [w2217]
          tunnel: w2174 -> [w2226]
          tunnel: [w2226] -> w2172
          tunnel: w2173 -> [w2225]
          tunnel: [w2225] -> w2171
          tunnel: w2172 -> [w2232]
          tunnel: [w2231] -> w2170
          tunnel: w2171 -> [w2230]
          tunnel: [w2229] -> w2169
          tunnel: w2170 -> [w2238]
          tunnel: w2169 -> [w2237]
          tunnel: [w2238] -> w2168
          tunnel: [w2237] -> w2167
          tunnel: w2168 -> [w2243]
          tunnel: w2167 -> [w2242]
          tunnel: [w2243] -> w2166
          tunnel: [w2242] -> w2165
          tunnel: [w2245] -> w2161
          tunnel: [w2246] -> w2162
          tunnel: w2166 -> [w2246]
          tunnel: w2165 -> [w2245]
          frame #0 {
            n1227 = property on="R Scan Velocity SP steps/sec" class="DigNum (strict)"() -> ("Value"=w2222:i32)  [unwired: 2 in, 2 out]
            n1228 = Number To Decimal String(number=w2222) -> (decimal integer string=w2223:string)  [unwired: 1 in]
            n1229 = call "mdrive send command.vi"("error in (no error)"=w2218, "Extra"=w2223, "Command"=T10."Max Velocity", "VISA resource name"=w2217) -> ("error out"=w2219:errorcluster, "VISA resource name out"=w2220:refnum<visa-resource-name>)  [unwired: 3 in, 1 out]
          }
          frame #1 {
            n1230 = Wait (ms)(milliseconds to wait=u32 100) -> ()  [unwired: 1 out]
          }
          frame #2 {
            # "VELOCITY"
            n1231 = call "mdrive send command.vi"("error in (no error)"=w2230, "Extra"="VM", "Command"=T10."Print Parameter", "VISA resource name"=w2232) -> ("error out"=w2229:errorcluster, "read buffer"=w2234:string, "VISA resource name out"=w2231:refnum<visa-resource-name>)  [unwired: 3 in]
            n1232 = Decimal String To Number(string=w2234, offset=0) -> (number=w2233:i32)  [unwired: 1 in, 1 out]
            n1233 = property on="R velocity PV step/sec" class="DigNum (strict)"("Val(Sgnl)"=w2233) -> ()  [unwired: 2 in, 2 out]
          }
          frame #3 {
            n1234 = Wait (ms)(milliseconds to wait=u32 100) -> ()  [unwired: 1 out]
          }
          frame #4 {
            n1235 = property on="R Scan Velocity SP steps/sec" class="DigNum (strict)"("DisabledEnum"=T1."Disabled and Grayed Out" ("Disabled")) -> ()  [unwired: 2 in, 2 out]
            n1236 = property on="R Scan Length SP steps" class="DigNum (strict)"("DisabledEnum"=T1."Disabled and Grayed Out" ("Disabled")) -> ()  [unwired: 2 in, 2 out]
            n1237 = property on="Scan Go" class="Bool (strict)"("DisabledEnum"=T1."Enabled" ("Disabled")) -> ()  [unwired: 2 in, 2 out]
          }
          frame #5 {
            n1238 = property on="R Scan" class="Bool (strict)"("Val(Sgnl)"=TRUE ("Slew Ready 2")) -> ()  [unwired: 2 in, 2 out]
          }
        }
        n1239 = property on="GO" class="Bool"("DisabledEnum"=T1."Disabled and Grayed Out" ("Disabled")) -> ()  [unwired: 2 in, 2 out]
        n1240 = local write "STATUS"("READY TO SCAN" ("STATUS")) -> ()
      }
      event #13 {
        n1241 = event-data() -> ()  [unwired: 1 in, 7 out]
        n1242 = flat-sequence {
          tunnel: [w2389] -> w2359
          tunnel: [w2388] -> w2358
          tunnel: w2347 -> [w2386]
          tunnel: w2345 -> [w2385]
          tunnel: [w2393] -> w2356
          tunnel: [w2394] -> w2357
          tunnel: w2359 -> [w2394]
          tunnel: w2358 -> [w2393]
          frame #0 {
            n1243 = call "mdrive send command.vi"("error in (no error)"=w2385, "Command"=T10."Stop", "VISA resource name"=w2386) -> ("error out"=w2388:errorcluster, "VISA resource name out"=w2389:refnum<visa-resource-name>)  [unwired: 4 in, 1 out]
          }
          frame #1 {
            n1244 = property on="X Scan" class="Bool (strict)"("Value"=FALSE ("Slew Ready")) -> ()  [unwired: 2 in, 2 out]
            n1245 = property on="X Scan Velocity SP steps/sec" class="DigNum (strict)"("DisabledEnum"=T1."Enabled" ("Disabled")) -> ()  [unwired: 2 in, 2 out]
            n1246 = property on="X Scan Length SP steps" class="DigNum (strict)"("DisabledEnum"=T1."Enabled" ("Disabled")) -> ()  [unwired: 2 in, 2 out]
          }
        }
        n1247 = flat-sequence {
          tunnel: [w2379] -> w2355
          tunnel: [w2378] -> w2354
          tunnel: w2346 -> [w2376]
          tunnel: w2344 -> [w2375]
          tunnel: [w2383] -> w2352
          tunnel: [w2384] -> w2353
          tunnel: w2355 -> [w2384]
          tunnel: w2354 -> [w2383]
          frame #0 {
            n1248 = call "mdrive send command.vi"("error in (no error)"=w2375, "Command"=T10."Stop", "VISA resource name"=w2376) -> ("error out"=w2378:errorcluster, "VISA resource name out"=w2379:refnum<visa-resource-name>)  [unwired: 4 in, 1 out]
          }
          frame #1 {
            n1249 = property on="Z Scan" class="Bool (strict)"("Value"=FALSE ("Slew Ready")) -> ()  [unwired: 2 in, 2 out]
            n1250 = property on="Z Scan Length SP steps" class="DigNum (strict)"("DisabledEnum"=T1."Enabled" ("Disabled")) -> ()  [unwired: 2 in, 2 out]
            n1251 = property on="Z Scan Velocity SP steps/sec" class="DigNum (strict)"("DisabledEnum"=T1."Enabled" ("Disabled")) -> ()  [unwired: 2 in, 2 out]
          }
        }
        n1252 = flat-sequence {
          tunnel: [w2399] -> w2361
          tunnel: [w2398] -> w2360
          tunnel: w2343 -> [w2396]
          tunnel: w2341 -> [w2395]
          tunnel: [w2403] -> w2363
          tunnel: [w2404] -> w2364
          tunnel: w2361 -> [w2404]
          tunnel: w2360 -> [w2403]
          frame #0 {
            n1253 = call "mdrive send command.vi"("error in (no error)"=w2395, "Command"=T10."Stop", "VISA resource name"=w2396) -> ("error out"=w2398:errorcluster, "VISA resource name out"=w2399:refnum<visa-resource-name>)  [unwired: 4 in, 1 out]
          }
          frame #1 {
            n1254 = property on="Y Scan" class="Bool (strict)"("Value"=FALSE ("Slew Ready")) -> ()  [unwired: 2 in, 2 out]
            n1255 = property on="Y Scan Velocity SP steps/sec" class="DigNum (strict)"("DisabledEnum"=T1."Enabled" ("Disabled")) -> ()  [unwired: 2 in, 2 out]
            n1256 = property on="Y Scan Length SP steps" class="DigNum (strict)"("DisabledEnum"=T1."Enabled" ("Disabled")) -> ()  [unwired: 2 in, 2 out]
          }
        }
        n1257 = flat-sequence {
          tunnel: [w2369] -> w2351
          tunnel: [w2368] -> w2350
          tunnel: w2342 -> [w2366]
          tunnel: w2340 -> [w2365]
          tunnel: [w2373] -> w2348
          tunnel: [w2374] -> w2349
          tunnel: w2351 -> [w2374]
          tunnel: w2350 -> [w2373]
          frame #0 {
            n1258 = call "mdrive send command.vi"("error in (no error)"=w2365, "Command"=T10."Stop", "VISA resource name"=w2366) -> ("error out"=w2368:errorcluster, "VISA resource name out"=w2369:refnum<visa-resource-name>)  [unwired: 4 in, 1 out]
          }
          frame #1 {
            n1259 = property on="R Scan" class="Bool (strict)"("Value"=FALSE ("Slew Ready")) -> ()  [unwired: 2 in, 2 out]
            n1260 = property on="R Scan Velocity SP steps/sec" class="DigNum (strict)"("DisabledEnum"=T1."Enabled" ("Disabled")) -> ()  [unwired: 2 in, 2 out]
            n1261 = property on="R Scan Length SP steps" class="DigNum (strict)"("DisabledEnum"=T1."Enabled" ("Disabled")) -> ()  [unwired: 2 in, 2 out]
          }
        }
        n1262 = property on="Set scan parameter" class="Bool"("DisabledEnum"=T1."Enabled" ("Disabled")) -> ()  [unwired: 2 in, 2 out]
        n1263 = property on="Scan Go" class="Bool (strict)"("DisabledEnum"=T1."Disabled and Grayed Out" ("Disabled")) -> ()  [unwired: 2 in, 2 out]
        n1264 = property on="GO" class="Bool"("DisabledEnum"=T1."Enabled" ("Disabled")) -> ()  [unwired: 2 in, 2 out]
        n1265 = property on="Review Scan \nParameters" class="Bool"("DisabledEnum"=T1."Enabled" ("Disabled")) -> ()  [unwired: 2 in, 2 out]
      }
      event #14 {
        w2405 = T1."Disabled and Grayed Out" ("Disabled")
        n1266 = event-data() -> ()  [unwired: 1 in, 7 out]
        n1267 = flat-sequence {
          tunnel: [w2486] -> w2470
          tunnel: [w2484] -> w2463
          tunnel: [w2485] -> w2460
          tunnel: [w2479] -> w2459
          tunnel: [w2483] -> w2458
          tunnel: [w2482] -> w2457
          tunnel: [w2481] -> w2456
          tunnel: [w2480] -> w2455
          tunnel: w2422 -> [w2478]
          tunnel: w2421 -> [w2477]
          tunnel: w2420 -> [w2476]
          tunnel: w2419 -> [w2475]
          tunnel: w2418 -> [w2474]
          tunnel: w2417 -> [w2473]
          tunnel: w2416 -> [w2472]
          tunnel: w2415 -> [w2471]
          tunnel: [w2478] -> w2414
          tunnel: [w2477] -> w2413
          tunnel: [w2476] -> w2412
          tunnel: [w2475] -> w2411
          tunnel: [w2474] -> w2410
          tunnel: [w2473] -> w2409
          tunnel: [w2472] -> w2408
          tunnel: [w2471] -> w2407
          tunnel: [w2538] -> w2467
          tunnel: [w2537] -> w2465
          tunnel: w2470 -> [w2536]
          tunnel: w2463 -> [w2535]
          tunnel: [w2535] -> w2461
          tunnel: w2460 -> [w2534]
          tunnel: w2459 -> [w2523]
          tunnel: w2458 -> [w2533]
          tunnel: w2457 -> [w2529]
          tunnel: w2456 -> [w2526]
          tunnel: w2455 -> [w2532]
          tunnel: [w2531] -> w2453
          tunnel: [w2530] -> w2451
          tunnel: [w2529] -> w2448
          tunnel: [w2528] -> w2446
          tunnel: [w2527] -> w2444
          tunnel: [w2526] -> w2442
          tunnel: [w2525] -> w2440
          tunnel: [w2524] -> w2438
          tunnel: [w2523] -> w2437
          tunnel: w2414 -> [w2522]
          tunnel: w2413 -> [w2521]
          tunnel: w2412 -> [w2520]
          tunnel: w2411 -> [w2519]
          tunnel: w2410 -> [w2518]
          tunnel: w2409 -> [w2517]
          tunnel: w2408 -> [w2516]
          tunnel: w2407 -> [w2515]
          tunnel: w2467 -> [w2579]
          tunnel: [w2579] -> w2466
          tunnel: w2465 -> [w2578]
          tunnel: [w2578] -> w2464
          tunnel: [w2577] -> w2462
          tunnel: w2461 -> [w2577]
          tunnel: [w2576] -> w2454
          tunnel: w2453 -> [w2576]
          tunnel: [w2575] -> w2452
          tunnel: w2451 -> [w2575]
          tunnel: [w2574] -> w2450
          tunnel: [w2573] -> w2449
          tunnel: w2448 -> [w2573]
          tunnel: [w2572] -> w2447
          tunnel: w2446 -> [w2572]
          tunnel: [w2571] -> w2445
          tunnel: w2444 -> [w2571]
          tunnel: [w2570] -> w2443
          tunnel: w2442 -> [w2570]
          tunnel: [w2569] -> w2441
          tunnel: w2440 -> [w2569]
          tunnel: [w2568] -> w2439
          tunnel: w2438 -> [w2568]
          tunnel: w2437 -> [w2574]
          tunnel: w2466 -> [w2599]
          tunnel: [w2597] -> w2469
          tunnel: w2464 -> [w2598]
          tunnel: [w2596] -> w2468
          tunnel: w2462 -> [w2595]
          tunnel: w2454 -> [w2594]
          tunnel: w2452 -> [w2593]
          tunnel: w2450 -> [w2592]
          tunnel: w2449 -> [w2591]
          tunnel: w2447 -> [w2590]
          tunnel: w2445 -> [w2589]
          tunnel: w2443 -> [w2588]
          tunnel: w2441 -> [w2587]
          tunnel: w2439 -> [w2586]
          tunnel: [w2585] -> w2436
          tunnel: [w2584] -> w2435
          tunnel: [w2583] -> w2430
          tunnel: [w2582] -> w2427
          tunnel: [w2581] -> w2425
          tunnel: [w2580] -> w2423
          tunnel: w2469 -> [w2656]
          tunnel: w2468 -> [w2655]
          tunnel: [w2656] -> w2434
          tunnel: [w2655] -> w2433
          tunnel: [w2650] -> w2432
          tunnel: w2436 -> [w2650]
          tunnel: [w2649] -> w2431
          tunnel: w2435 -> [w2649]
          tunnel: w2430 -> [w2639]
          tunnel: [w2639] -> w2429
          tunnel: [w2638] -> w2428
          tunnel: w2427 -> [w2638]
          tunnel: [w2637] -> w2426
          tunnel: w2425 -> [w2637]
          tunnel: [w2636] -> w2424
          tunnel: w2423 -> [w2636]
          frame #0 {
            n1268 = property on="X Scan" class="Bool (strict)"() -> ("Value"=w2479:bool)  [unwired: 2 in, 2 out]
            n1269 = property on="Z Scan" class="Bool (strict)"() -> ("Value"=w2481:bool)  [unwired: 2 in, 2 out]
            n1270 = property on="Y Scan" class="Bool (strict)"() -> ("Value"=w2484:bool)  [unwired: 2 in, 2 out]
            n1271 = property on="R Scan" class="Bool (strict)"() -> ("Value"=w2482:bool)  [unwired: 2 in, 2 out]
            n1272 = case shown="False" w2484 {
              tunnel: ["" w2509] -> w2486
              frame #0 {
              }
              frame #1 {
                n1273 = property on="Y Scan Length SP steps" class="DigNum (strict)"() -> ("Value"=w2514:i32)  [unwired: 2 in, 2 out]
                n1274 = Number To Decimal String(number=w2514) -> (decimal integer string=w2511:string)  [unwired: 1 in]
                n1275 = call <vilib>:"Space Constant.vi"() -> ("String"=w2512:string)
                n1276 = Concatenate Strings("MR", w2512, w2511, "\r") -> (w2509:string)
              }
            }
            n1277 = case shown="False" w2479 {
              tunnel: ["" w2502] -> w2485
              frame #0 {
              }
              frame #1 {
                n1278 = property on="X Scan Length SP steps" class="DigNum (strict)"() -> ("Value"=w2507:i32)  [unwired: 2 in, 2 out]
                n1279 = Number To Decimal String(number=w2507) -> (decimal integer string=w2504:string)  [unwired: 1 in]
                n1280 = call <vilib>:"Space Constant.vi"() -> ("String"=w2505:string)
                n1281 = Concatenate Strings("MR", w2505, w2504, "\r") -> (w2502:string)
              }
            }
            n1282 = case shown="False" w2482 {
              tunnel: ["" w2488] -> w2480
              frame #0 {
              }
              frame #1 {
                n1283 = property on="R Scan Length SP steps" class="DigNum (strict)"() -> ("Value"=w2493:i32)  [unwired: 2 in, 2 out]
                n1284 = Number To Decimal String(number=w2493) -> (decimal integer string=w2490:string)  [unwired: 1 in]
                n1285 = call <vilib>:"Space Constant.vi"() -> ("String"=w2491:string)
                n1286 = Concatenate Strings("MR", w2491, w2490, "\r") -> (w2488:string)
              }
            }
            n1287 = case shown="False" w2481 {
              tunnel: ["" w2495] -> w2483
              frame #0 {
              }
              frame #1 {
                n1288 = property on="Z Scan Length SP steps" class="DigNum (strict)"() -> ("Value"=w2500:i32)  [unwired: 2 in, 2 out]
                n1289 = Number To Decimal String(number=w2500) -> (decimal integer string=w2497:string)  [unwired: 1 in]
                n1290 = call <vilib>:"Space Constant.vi"() -> ("String"=w2498:string)
                n1291 = Concatenate Strings("MR", w2498, w2497, "\r") -> (w2495:string)
              }
            }
          }
          frame #1 {
            n1292 = case shown="False" w2523 {
              tunnel: [w2554 w2559] -> w2531
              tunnel: [w2553 w2558] -> w2530
              tunnel: w2534 -> [_ w2557]
              tunnel: w2522 -> [w2554 w2556]
              tunnel: w2521 -> [w2553 w2555]
              frame #0 {
              }
              frame #1 {
                n1293 = VISA Write(VISA resource name=w2556, write buffer=w2557, error in (no error)=w2555) -> (VISA resource name out=w2559:refnum<visa-resource-name>, error out=w2558:errorcluster)  [unwired: 1 out]
              }
            }
            n1294 = case shown="True" w2526 {
              tunnel: [w2547 w2552] -> w2525
              tunnel: [w2546 w2551] -> w2524
              tunnel: w2533 -> [_ w2550]
              tunnel: w2520 -> [w2547 w2549]
              tunnel: w2519 -> [w2546 w2548]
              frame #0 {
              }
              frame #1 {
                n1295 = VISA Write(VISA resource name=w2549, write buffer=w2550, error in (no error)=w2548) -> (VISA resource name out=w2552:refnum<visa-resource-name>, error out=w2551:errorcluster)  [unwired: 1 out]
              }
            }
            n1296 = case shown="True" w2535 {
              tunnel: [w2561 w2566] -> w2538
              tunnel: [w2560 w2565] -> w2537
              tunnel: w2536 -> [_ w2564]
              tunnel: w2518 -> [w2561 w2563]
              tunnel: w2517 -> [w2560 w2562]
              frame #0 {
              }
              frame #1 {
                n1297 = VISA Write(VISA resource name=w2563, write buffer=w2564, error in (no error)=w2562) -> (VISA resource name out=w2566:refnum<visa-resource-name>, error out=w2565:errorcluster)  [unwired: 1 out]
              }
            }
            n1298 = case shown="True" w2529 {
              tunnel: [w2540 w2545] -> w2528
              tunnel: [w2539 w2544] -> w2527
              tunnel: w2532 -> [_ w2543]
              tunnel: w2516 -> [w2540 w2542]
              tunnel: w2515 -> [w2539 w2541]
              frame #0 {
              }
              frame #1 {
                n1299 = VISA Write(VISA resource name=w2542, write buffer=w2543, error in (no error)=w2541) -> (VISA resource name out=w2545:refnum<visa-resource-name>, error out=w2544:errorcluster)  [unwired: 1 out]
              }
            }
          }
          frame #2 {
            n1300 = Wait (ms)(milliseconds to wait=u32 100) -> ()  [unwired: 1 out]
          }
          frame #3 {
            n1301 = case shown="True" w2592 {
              tunnel: w2594 -> [w2619 w2623]
              tunnel: w2593 -> [w2618 w2622]
              tunnel: [w2619 w2621] -> w2581
              tunnel: [w2618 w2620] -> w2580
              frame #0 {
              }
              frame #1 {
                n1302 = property class="Instr"(reference=w2623, error in=w2622) -> (reference out=w2625:refnum<visa-resource-name>, error out=w2624:errorcluster, "Serial Settings:Number of Bytes at Serial Port"=w2626:u32)
                n1303 = VISA Read(VISA resource name=w2625, byte count=w2626, error in (no error)=w2624) -> (VISA resource name out=w2621:refnum<visa-resource-name>, error out=w2620:errorcluster)  [unwired: 2 out]
              }
            }
            n1304 = case shown="True" w2588 {
              tunnel: w2587 -> [w2601 w2605]
              tunnel: w2586 -> [w2600 w2604]
              tunnel: [w2601 w2603] -> w2585
              tunnel: [w2600 w2602] -> w2584
              frame #0 {
              }
              frame #1 {
                n1305 = property class="Instr"(reference=w2605, error in=w2604) -> (reference out=w2607:refnum<visa-resource-name>, error out=w2606:errorcluster, "Serial Settings:Number of Bytes at Serial Port"=w2608:u32)
                n1306 = VISA Read(VISA resource name=w2607, byte count=w2608, error in (no error)=w2606) -> (VISA resource name out=w2603:refnum<visa-resource-name>, error out=w2602:errorcluster)  [unwired: 2 out]
              }
            }
            n1307 = case shown="True" w2595 {
              tunnel: w2599 -> [w2628 w2632]
              tunnel: w2598 -> [w2627 w2631]
              tunnel: [w2628 w2630] -> w2597
              tunnel: [w2627 w2629] -> w2596
              frame #0 {
              }
              frame #1 {
                n1308 = property class="Instr"(reference=w2632, error in=w2631) -> (reference out=w2634:refnum<visa-resource-name>, error out=w2633:errorcluster, "Serial Settings:Number of Bytes at Serial Port"=w2635:u32)
                n1309 = VISA Read(VISA resource name=w2634, byte count=w2635, error in (no error)=w2633) -> (VISA resource name out=w2630:refnum<visa-resource-name>, error out=w2629:errorcluster)  [unwired: 2 out]
              }
            }
            n1310 = case shown="True" w2591 {
              tunnel: w2590 -> [w2610 w2614]
              tunnel: w2589 -> [w2609 w2613]
              tunnel: [w2610 w2612] -> w2583
              tunnel: [w2609 w2611] -> w2582
              frame #0 {
              }
              frame #1 {
                n1311 = property class="Instr"(reference=w2614, error in=w2613) -> (reference out=w2616:refnum<visa-resource-name>, error out=w2615:errorcluster, "Serial Settings:Number of Bytes at Serial Port"=w2617:u32)
                n1312 = VISA Read(VISA resource name=w2616, byte count=w2617, error in (no error)=w2615) -> (VISA resource name out=w2612:refnum<visa-resource-name>, error out=w2611:errorcluster)  [unwired: 2 out]
              }
            }
          }
          frame #4 {
            n1313 = property on="Y Scan" class="Bool (strict)"("Val(Sgnl)"=FALSE ("Slew Ready 2")) -> ()  [unwired: 2 in, 2 out]
            n1314 = property on="Z Scan" class="Bool (strict)"("Val(Sgnl)"=FALSE ("Slew Ready 2")) -> ()  [unwired: 2 in, 2 out]
            n1315 = property on="X Scan" class="Bool (strict)"("Val(Sgnl)"=FALSE ("Slew Ready 2")) -> ()  [unwired: 2 in, 2 out]
            n1316 = property on="R Scan" class="Bool (strict)"("Val(Sgnl)"=FALSE ("Slew Ready 2")) -> ()  [unwired: 2 in, 2 out]
            n1317 = property on="R Scan Length SP steps" class="DigNum (strict)"("DisabledEnum"=T1."Enabled" ("Disabled")) -> ()  [unwired: 2 in, 2 out]
            n1318 = property on="Y Scan Selocity SP steps/sec" class="DigNum (strict)"("DisabledEnum"=T1."Enabled" ("Disabled")) -> ()  [unwired: 2 in, 2 out]
            n1319 = property on="Scan Go" class="Bool (strict)"("DisabledEnum"=T1."Disabled and Grayed Out" ("Disabled")) -> ()  [unwired: 2 in, 2 out]
            n1320 = property on="Z Scan Velocity SP steps/sec" class="DigNum (strict)"("DisabledEnum"=T1."Enabled" ("Disabled")) -> ()  [unwired: 2 in, 2 out]
            n1321 = property on="X Scan Velocity SP steps/sec" class="DigNum (strict)"("DisabledEnum"=T1."Enabled" ("Disabled")) -> ()  [unwired: 2 in, 2 out]
            n1322 = property on="Y Scan Length SP steps" class="DigNum (strict)"("DisabledEnum"=T1."Enabled" ("Disabled")) -> ()  [unwired: 2 in, 2 out]
            n1323 = property on="R Scan Velocity SP steps/sec" class="DigNum (strict)"("DisabledEnum"=T1."Enabled" ("Disabled")) -> ()  [unwired: 2 in, 2 out]
            n1324 = property on="X Scan Length SP steps" class="DigNum (strict)"("DisabledEnum"=T1."Enabled" ("Disabled")) -> ()  [unwired: 2 in, 2 out]
            n1325 = property on="Z Scan Length SP steps" class="DigNum (strict)"("DisabledEnum"=T1."Enabled" ("Disabled")) -> ()  [unwired: 2 in, 2 out]
          }
        }
        n1326 = local write "STATUS"("SCANNING" ("STATUS")) -> ()
        n1327 = property on="GO" class="Bool"("DisabledEnum"=w2405) -> ()  [unwired: 2 in, 2 out]
        n1328 = property on="Review Scan \nParameters" class="Bool"("DisabledEnum"=w2405) -> ()  [unwired: 2 in, 2 out]
        n1329 = property on="Set scan parameter" class="Bool"("DisabledEnum"=w2405) -> ()  [unwired: 2 in, 2 out]
      }
      event #15 {
        n1330 = event-data() -> ()  [unwired: 1 in, 7 out]
        n1331 = flat-sequence {
          tunnel: [w2696] -> w2672
          tunnel: [w2697] -> w2671
          tunnel: w2664 -> [w2695]
          tunnel: w2660 -> [w2694]
          frame #0 {
            n1332 = property on="Reset X Motor Steps" class="DigNum (strict)"() -> ("Value"=w2698:i32)  [unwired: 2 in, 2 out]
            n1333 = Number To Decimal String(number=w2698) -> (decimal integer string=w2699:string)  [unwired: 1 in]
            n1334 = call "mdrive send command.vi"("error in (no error)"=w2695, "Extra"=w2699, "Command"=T10."Set Current Position", "VISA resource name"=w2694) -> ("error out"=w2697:errorcluster, "VISA resource name out"=w2696:refnum<visa-resource-name>)  [unwired: 3 in, 1 out]
          }
        }
        n1335 = flat-sequence {
          tunnel: [w2690] -> w2670
          tunnel: [w2691] -> w2669
          tunnel: w2663 -> [w2688]
          tunnel: w2659 -> [w2687]
          frame #0 {
            n1336 = property on="Reset Z Motor Steps" class="DigNum (strict)"() -> ("Value"=w2689:i32)  [unwired: 2 in, 2 out]
            n1337 = Number To Decimal String(number=w2689) -> (decimal integer string=w2692:string)  [unwired: 1 in]
            n1338 = call "mdrive send command.vi"("error in (no error)"=w2688, "Extra"=w2692, "Command"=T10."Set Current Position", "VISA resource name"=w2687) -> ("error out"=w2691:errorcluster, "VISA resource name out"=w2690:refnum<visa-resource-name>)  [unwired: 3 in, 1 out]
          }
        }
        n1339 = flat-sequence {
          tunnel: [w2683] -> w2668
          tunnel: [w2684] -> w2667
          tunnel: w2662 -> [w2681]
          tunnel: w2658 -> [w2680]
          frame #0 {
            n1340 = property on="Reset Y Motor Steps" class="DigNum (strict)"() -> ("Value"=w2682:i32)  [unwired: 2 in, 2 out]
            n1341 = Number To Decimal String(number=w2682) -> (decimal integer string=w2685:string)  [unwired: 1 in]
            n1342 = call "mdrive send command.vi"("error in (no error)"=w2681, "Extra"=w2685, "Command"=T10."Set Current Position", "VISA resource name"=w2680) -> ("error out"=w2684:errorcluster, "VISA resource name out"=w2683:refnum<visa-resource-name>)  [unwired: 3 in, 1 out]
          }
        }
        n1343 = flat-sequence {
          tunnel: [w2676] -> w2666
          tunnel: [w2677] -> w2665
          tunnel: w2661 -> [w2674]
          tunnel: w2657 -> [w2673]
          frame #0 {
            n1344 = property on="Reset R Motor Steps" class="DigNum (strict)"() -> ("Value"=w2675:i32)  [unwired: 2 in, 2 out]
            n1345 = Number To Decimal String(number=w2675) -> (decimal integer string=w2678:string)  [unwired: 1 in]
            n1346 = call "mdrive send command.vi"("error in (no error)"=w2674, "Extra"=w2678, "Command"=T10."Set Current Position", "VISA resource name"=w2673) -> ("error out"=w2677:errorcluster, "VISA resource name out"=w2676:refnum<visa-resource-name>)  [unwired: 3 in, 1 out]
          }
        }
      }
      event #16 {
        n1347 = event-data() -> ()  [unwired: 1 in, 5 out]
        n1348 = property on="LOOP REQ" class="Bool (strict)"() -> ("Value"=w2701:bool)  [unwired: 2 in, 2 out]
        n1349 = case shown="True" w2701 {
          tunnel: [w2721 w2751] -> w2717
          tunnel: [w2720 w2750] -> w2716
          tunnel: [w2723 w2749] -> w2715
          tunnel: [w2722 w2748] -> w2714
          tunnel: [w2719 w2747] -> w2713
          tunnel: [w2718 w2746] -> w2712
          tunnel: [w2725 w2745] -> w2711
          tunnel: [w2724 w2744] -> w2710
          tunnel: w2709 -> [w2723 w2741]
          tunnel: w2708 -> [w2725 w2740]
          tunnel: w2707 -> [w2719 w2736]
          tunnel: w2706 -> [w2721 w2735]
          tunnel: w2705 -> [w2718 w2732]
          tunnel: w2704 -> [w2720 w2731]
          tunnel: w2703 -> [w2722 w2729]
          tunnel: w2702 -> [w2724 w2727]
          frame #0 {
          }
          frame #1 {
            w2742 = T1."Disabled and Grayed Out" ("Disabled")
            n1350 = flat-sequence {
              tunnel: [w2903] -> w2781
              tunnel: [w2902] -> w2780
              tunnel: w2731 -> [w2901]
              tunnel: w2735 -> [w2900]
              tunnel: w2781 -> [w2909]
              tunnel: [w2909] -> w2779
              tunnel: w2780 -> [w2908]
              tunnel: [w2908] -> w2778
              tunnel: w2779 -> [w2913]
              tunnel: [w2912] -> w2777
              tunnel: w2778 -> [w2911]
              tunnel: [w2910] -> w2776
              tunnel: w2777 -> [w2921]
              tunnel: [w2921] -> w2775
              tunnel: w2776 -> [w2920]
              tunnel: [w2920] -> w2774
              tunnel: w2775 -> [w2926]
              tunnel: w2774 -> [w2925]
              tunnel: [w2926] -> w2773
              tunnel: [w2925] -> w2772
              tunnel: [w2928] -> w2730
              tunnel: [w2929] -> w2734
              tunnel: w2773 -> [w2929]
              tunnel: w2772 -> [w2928]
              frame #0 {
                n1351 = property on="Y Scan Velocity SP steps/sec" class="DigNum (strict)"() -> ("Value"=w2905:i32)  [unwired: 2 in, 2 out]
                n1352 = Number To Decimal String(number=w2905) -> (decimal integer string=w2906:string)  [unwired: 1 in]
                n1353 = call "mdrive send command.vi"("error in (no error)"=w2901, "Extra"=w2906, "Command"=T10."Max Velocity", "VISA resource name"=w2900) -> ("error out"=w2902:errorcluster, "VISA resource name out"=w2903:refnum<visa-resource-name>)  [unwired: 3 in, 1 out]
              }
              frame #1 {
                n1354 = Wait (ms)(milliseconds to wait=u32 100) -> ()  [unwired: 1 out]
              }
              frame #2 {
                # "VELOCITY"
                n1355 = call "mdrive send command.vi"("error in (no error)"=w2911, "Extra"="VM", "Command"=T10."Print Parameter", "VISA resource name"=w2913) -> ("error out"=w2910:errorcluster, "read buffer"=w2917:string, "VISA resource name out"=w2912:refnum<visa-resource-name>)  [unwired: 3 in]
                n1356 = Decimal String To Number(string=w2917, offset=0) -> (number=w2915:i32)  [unwired: 1 in, 1 out]
                n1357 = property on="Y velocity PV step/sec" class="DigNum (strict)"("Val(Sgnl)"=w2915) -> ()  [unwired: 2 in, 2 out]
              }
              frame #3 {
                n1358 = Wait (ms)(milliseconds to wait=u32 100) -> ()  [unwired: 1 out]
              }
              frame #4 {
                n1359 = property on="Y Scan Velocity SP steps/sec" class="DigNum (strict)"("DisabledEnum"=T1."Disabled and Grayed Out" ("Disabled")) -> ()  [unwired: 2 in, 2 out]
                n1360 = property on="Y Scan Length SP steps" class="DigNum (strict)"("DisabledEnum"=T1."Disabled and Grayed Out" ("Disabled")) -> ()  [unwired: 2 in, 2 out]
                n1361 = property on="Scan Go" class="Bool (strict)"("DisabledEnum"=T1."Enabled" ("Disabled")) -> ()  [unwired: 2 in, 2 out]
              }
              frame #5 {
                n1362 = property on="Y Scan" class="Bool (strict)"("Val(Sgnl)"=TRUE ("Slew Ready 2")) -> ()  [unwired: 2 in, 2 out]
              }
            }
            n1363 = flat-sequence {
              tunnel: [w2843] -> w2761
              tunnel: [w2842] -> w2760
              tunnel: w2732 -> [w2841]
              tunnel: w2736 -> [w2840]
              tunnel: w2761 -> [w2849]
              tunnel: [w2849] -> w2759
              tunnel: w2760 -> [w2848]
              tunnel: [w2848] -> w2758
              tunnel: w2759 -> [w2855]
              tunnel: [w2854] -> w2757
              tunnel: w2758 -> [w2853]
              tunnel: [w2852] -> w2756
              tunnel: w2757 -> [w2861]
              tunnel: w2756 -> [w2860]
              tunnel: [w2861] -> w2755
              tunnel: [w2860] -> w2754
              tunnel: w2755 -> [w2866]
              tunnel: w2754 -> [w2865]
              tunnel: [w2866] -> w2753
              tunnel: [w2865] -> w2752
              tunnel: [w2868] -> w2733
              tunnel: [w2869] -> w2737
              tunnel: w2753 -> [w2869]
              tunnel: w2752 -> [w2868]
              frame #0 {
                n1364 = property on="R Scan Velocity SP steps/sec" class="DigNum (strict)"() -> ("Value"=w2845:i32)  [unwired: 2 in, 2 out]
                n1365 = Number To Decimal String(number=w2845) -> (decimal integer string=w2846:string)  [unwired: 1 in]
                n1366 = call "mdrive send command.vi"("error in (no error)"=w2841, "Extra"=w2846, "Command"=T10."Max Velocity", "VISA resource name"=w2840) -> ("error out"=w2842:errorcluster, "VISA resource name out"=w2843:refnum<visa-resource-name>)  [unwired: 3 in, 1 out]
              }
              frame #1 {
                n1367 = Wait (ms)(milliseconds to wait=u32 100) -> ()  [unwired: 1 out]
              }
              frame #2 {
                # "VELOCITY"
                n1368 = call "mdrive send command.vi"("error in (no error)"=w2853, "Extra"="VM", "Command"=T10."Print Parameter", "VISA resource name"=w2855) -> ("error out"=w2852:errorcluster, "read buffer"=w2857:string, "VISA resource name out"=w2854:refnum<visa-resource-name>)  [unwired: 3 in]
                n1369 = Decimal String To Number(string=w2857, offset=0) -> (number=w2856:i32)  [unwired: 1 in, 1 out]
                n1370 = property on="R velocity PV step/sec" class="DigNum (strict)"("Val(Sgnl)"=w2856) -> ()  [unwired: 2 in, 2 out]
              }
              frame #3 {
                n1371 = Wait (ms)(milliseconds to wait=u32 100) -> ()  [unwired: 1 out]
              }
              frame #4 {
                n1372 = property on="R Scan Velocity SP steps/sec" class="DigNum (strict)"("DisabledEnum"=T1."Disabled and Grayed Out" ("Disabled")) -> ()  [unwired: 2 in, 2 out]
                n1373 = property on="R Scan Length SP steps" class="DigNum (strict)"("DisabledEnum"=T1."Disabled and Grayed Out" ("Disabled")) -> ()  [unwired: 2 in, 2 out]
                n1374 = property on="Scan Go" class="Bool (strict)"("DisabledEnum"=T1."Enabled" ("Disabled")) -> ()  [unwired: 2 in, 2 out]
              }
              frame #5 {
                n1375 = property on="R Scan" class="Bool (strict)"("Val(Sgnl)"=TRUE ("Slew Ready 2")) -> ()  [unwired: 2 in, 2 out]
              }
            }
            n1376 = flat-sequence {
              tunnel: [w2931] -> w2791
              tunnel: [w2930] -> w2790
              tunnel: w2727 -> [w2933]
              tunnel: w2740 -> [w2932]
              tunnel: w2791 -> [w2939]
              tunnel: [w2939] -> w2789
              tunnel: w2790 -> [w2938]
              tunnel: [w2938] -> w2788
              tunnel: w2789 -> [w2943]
              tunnel: [w2942] -> w2787
              tunnel: w2788 -> [w2941]
              tunnel: [w2940] -> w2786
              tunnel: w2787 -> [w2951]
              tunnel: [w2951] -> w2785
              tunnel: w2786 -> [w2950]
              tunnel: [w2950] -> w2784
              tunnel: w2785 -> [w2956]
              tunnel: w2784 -> [w2955]
              tunnel: [w2956] -> w2783
              tunnel: [w2955] -> w2782
              tunnel: [w2958] -> w2726
              tunnel: [w2959] -> w2739
              tunnel: w2783 -> [w2959]
              tunnel: w2782 -> [w2958]
              frame #0 {
                n1377 = property on="X Scan Velocity SP steps/sec" class="DigNum (strict)"() -> ("Value"=w2935:i32)  [unwired: 2 in, 2 out]
                n1378 = Number To Decimal String(number=w2935) -> (decimal integer string=w2936:string)  [unwired: 1 in]
                n1379 = call "mdrive send command.vi"("error in (no error)"=w2933, "Extra"=w2936, "Command"=T10."Max Velocity", "VISA resource name"=w2932) -> ("error out"=w2930:errorcluster, "VISA resource name out"=w2931:refnum<visa-resource-name>)  [unwired: 3 in, 1 out]
              }
              frame #1 {
                n1380 = Wait (ms)(milliseconds to wait=u32 100) -> ()  [unwired: 1 out]
              }
              frame #2 {
                # "VELOCITY"
                n1381 = call "mdrive send command.vi"("error in (no error)"=w2941, "Extra"="VM", "Command"=T10."Print Parameter", "VISA resource name"=w2943) -> ("error out"=w2940:errorcluster, "read buffer"=w2946:string, "VISA resource name out"=w2942:refnum<visa-resource-name>)  [unwired: 3 in]
                n1382 = Decimal String To Number(string=w2946, offset=0) -> (number=w2944:i32)  [unwired: 1 in, 1 out]
                n1383 = property on="X velocity PV step/sec" class="DigNum (strict)"("Val(Sgnl)"=w2944) -> ()  [unwired: 2 in, 2 out]
              }
              frame #3 {
                n1384 = Wait (ms)(milliseconds to wait=u32 100) -> ()  [unwired: 1 out]
              }
              frame #4 {
                n1385 = property on="X Scan Velocity SP steps/sec" class="DigNum (strict)"("DisabledEnum"=T1."Disabled and Grayed Out" ("Disabled")) -> ()  [unwired: 2 in, 2 out]
                n1386 = property on="X Scan Length SP steps" class="DigNum (strict)"("DisabledEnum"=T1."Disabled and Grayed Out" ("Disabled")) -> ()  [unwired: 2 in, 2 out]
                n1387 = property on="Scan Go" class="Bool (strict)"("DisabledEnum"=T1."Enabled" ("Disabled")) -> ()  [unwired: 2 in, 2 out]
              }
              frame #5 {
                n1388 = property on="X Scan" class="Bool (strict)"("Val(Sgnl)"=TRUE ("Slew Ready 2")) -> ()  [unwired: 2 in, 2 out]
              }
            }
            n1389 = flat-sequence {
              tunnel: [w2873] -> w2771
              tunnel: [w2872] -> w2770
              tunnel: w2729 -> [w2871]
              tunnel: w2741 -> [w2870]
              tunnel: w2771 -> [w2879]
              tunnel: [w2879] -> w2769
              tunnel: w2770 -> [w2878]
              tunnel: [w2878] -> w2768
              tunnel: w2769 -> [w2885]
              tunnel: [w2884] -> w2767
              tunnel: w2768 -> [w2883]
              tunnel: [w2882] -> w2766
              tunnel: w2767 -> [w2891]
              tunnel: [w2891] -> w2765
              tunnel: w2766 -> [w2890]
              tunnel: [w2890] -> w2764
              tunnel: w2765 -> [w2896]
              tunnel: w2764 -> [w2895]
              tunnel: [w2896] -> w2763
              tunnel: [w2895] -> w2762
              tunnel: [w2898] -> w2728
              tunnel: [w2899] -> w2738
              tunnel: w2763 -> [w2899]
              tunnel: w2762 -> [w2898]
              frame #0 {
                n1390 = property on="Z Scan Velocity SP steps/sec" class="DigNum (strict)"() -> ("Value"=w2875:i32)  [unwired: 2 in, 2 out]
                n1391 = Number To Decimal String(number=w2875) -> (decimal integer string=w2876:string)  [unwired: 1 in]
                n1392 = call "mdrive send command.vi"("error in (no error)"=w2871, "Extra"=w2876, "Command"=T10."Max Velocity", "VISA resource name"=w2870) -> ("error out"=w2872:errorcluster, "VISA resource name out"=w2873:refnum<visa-resource-name>)  [unwired: 3 in, 1 out]
              }
              frame #1 {
                n1393 = Wait (ms)(milliseconds to wait=u32 100) -> ()  [unwired: 1 out]
              }
              frame #2 {
                # "VELOCITY"
                n1394 = call "mdrive send command.vi"("error in (no error)"=w2883, "Extra"="VM", "Command"=T10."Print Parameter", "VISA resource name"=w2885) -> ("error out"=w2882:errorcluster, "read buffer"=w2886:string, "VISA resource name out"=w2884:refnum<visa-resource-name>)  [unwired: 3 in]
                n1395 = Decimal String To Number(string=w2886, offset=0) -> (number=w2887:i32)  [unwired: 1 in, 1 out]
                n1396 = property on="Z  velocity PV step/sec" class="DigNum (strict)"("Val(Sgnl)"=w2887) -> ()  [unwired: 2 in, 2 out]
              }
              frame #3 {
                n1397 = Wait (ms)(milliseconds to wait=u32 100) -> ()  [unwired: 1 out]
              }
              frame #4 {
                n1398 = property on="Z Scan Length SP steps" class="DigNum (strict)"("DisabledEnum"=T1."Disabled and Grayed Out" ("Disabled")) -> ()  [unwired: 2 in, 2 out]
                n1399 = property on="Z Scan Velocity SP steps/sec" class="DigNum (strict)"("DisabledEnum"=T1."Disabled and Grayed Out" ("Disabled")) -> ()  [unwired: 2 in, 2 out]
                n1400 = property on="Scan Go" class="Bool (strict)"("DisabledEnum"=T1."Enabled" ("Disabled")) -> ()  [unwired: 2 in, 2 out]
              }
              frame #5 {
                n1401 = property on="Z Scan" class="Bool (strict)"("Val(Sgnl)"=TRUE ("Slew Ready 2")) -> ()  [unwired: 2 in, 2 out]
              }
            }
            n1402 = flat-sequence {
              tunnel: [w2975] -> w2839
              tunnel: [w2973] -> w2838
              tunnel: [w2974] -> w2837
              tunnel: [w2960] -> w2836
              tunnel: [w2972] -> w2835
              tunnel: [w2971] -> w2834
              tunnel: [w2970] -> w2833
              tunnel: [w2969] -> w2832
              tunnel: w2739 -> [w2968]
              tunnel: w2726 -> [w2967]
              tunnel: w2738 -> [w2966]
              tunnel: w2728 -> [w2965]
              tunnel: w2734 -> [w2964]
              tunnel: w2730 -> [w2963]
              tunnel: w2737 -> [w2962]
              tunnel: w2733 -> [w2961]
              tunnel: [w2968] -> w2831
              tunnel: [w2967] -> w2830
              tunnel: [w2966] -> w2829
              tunnel: [w2965] -> w2828
              tunnel: [w2964] -> w2827
              tunnel: [w2963] -> w2826
              tunnel: [w2962] -> w2825
              tunnel: [w2961] -> w2824
              tunnel: [w3027] -> w2823
              tunnel: [w3026] -> w2822
              tunnel: w2839 -> [w3025]
              tunnel: w2838 -> [w3024]
              tunnel: [w3024] -> w2821
              tunnel: w2837 -> [w3023]
              tunnel: w2836 -> [w3012]
              tunnel: w2835 -> [w3022]
              tunnel: w2834 -> [w3018]
              tunnel: w2833 -> [w3015]
              tunnel: w2832 -> [w3021]
              tunnel: [w3020] -> w2820
              tunnel: [w3019] -> w2819
              tunnel: [w3018] -> w2818
              tunnel: [w3017] -> w2817
              tunnel: [w3016] -> w2816
              tunnel: [w3015] -> w2815
              tunnel: [w3014] -> w2814
              tunnel: [w3013] -> w2813
              tunnel: [w3012] -> w2812
              tunnel: w2831 -> [w3011]
              tunnel: w2830 -> [w3010]
              tunnel: w2829 -> [w3009]
              tunnel: w2828 -> [w3008]
              tunnel: w2827 -> [w3007]
              tunnel: w2826 -> [w3006]
              tunnel: w2825 -> [w3005]
              tunnel: w2824 -> [w3004]
              tunnel: w2823 -> [w3068]
              tunnel: [w3068] -> w2811
              tunnel: w2822 -> [w3067]
              tunnel: [w3067] -> w2810
              tunnel: [w3066] -> w2809
              tunnel: w2821 -> [w3066]
              tunnel: [w3065] -> w2808
              tunnel: w2820 -> [w3065]
              tunnel: [w3064] -> w2807
              tunnel: w2819 -> [w3064]
              tunnel: [w3063] -> w2806
              tunnel: [w3062] -> w2805
              tunnel: w2818 -> [w3062]
              tunnel: [w3061] -> w2804
              tunnel: w2817 -> [w3061]
              tunnel: [w3060] -> w2803
              tunnel: w2816 -> [w3060]
              tunnel: [w3059] -> w2802
              tunnel: w2815 -> [w3059]
              tunnel: [w3058] -> w2801
              tunnel: w2814 -> [w3058]
              tunnel: [w3057] -> w2800
              tunnel: w2813 -> [w3057]
              tunnel: w2812 -> [w3063]
              tunnel: w2811 -> [w3088]
              tunnel: [w3086] -> w2799
              tunnel: w2810 -> [w3087]
              tunnel: [w3085] -> w2798
              tunnel: w2809 -> [w3084]
              tunnel: w2808 -> [w3083]
              tunnel: w2807 -> [w3082]
              tunnel: w2806 -> [w3081]
              tunnel: w2805 -> [w3080]
              tunnel: w2804 -> [w3079]
              tunnel: w2803 -> [w3078]
              tunnel: w2802 -> [w3077]
              tunnel: w2801 -> [w3076]
              tunnel: w2800 -> [w3075]
              tunnel: [w3074] -> w2797
              tunnel: [w3073] -> w2796
              tunnel: [w3072] -> w2795
              tunnel: [w3071] -> w2794
              tunnel: [w3070] -> w2793
              tunnel: [w3069] -> w2792
              tunnel: w2799 -> [w3145]
              tunnel: w2798 -> [w3144]
              tunnel: [w3145] -> w2751
              tunnel: [w3144] -> w2750
              tunnel: [w3139] -> w2749
              tunnel: w2797 -> [w3139]
              tunnel: [w3138] -> w2748
              tunnel: w2796 -> [w3138]
              tunnel: w2795 -> [w3128]
              tunnel: [w3128] -> w2747
              tunnel: [w3127] -> w2746
              tunnel: w2794 -> [w3127]
              tunnel: [w3126] -> w2745
              tunnel: w2793 -> [w3126]
              tunnel: [w3125] -> w2744
              tunnel: w2792 -> [w3125]
              frame #0 {
                n1403 = property on="X Scan" class="Bool (strict)"() -> ("Value"=w2960:bool)  [unwired: 2 in, 2 out]
                n1404 = property on="Z Scan" class="Bool (strict)"() -> ("Value"=w2970:bool)  [unwired: 2 in, 2 out]
                n1405 = property on="Y Scan" class="Bool (strict)"() -> ("Value"=w2973:bool)  [unwired: 2 in, 2 out]
                n1406 = property on="R Scan" class="Bool (strict)"() -> ("Value"=w2971:bool)  [unwired: 2 in, 2 out]
                n1407 = case shown="False" w2973 {
                  tunnel: ["" w2998] -> w2975
                  frame #0 {
                  }
                  frame #1 {
                    n1408 = property on="Y Scan Length SP steps" class="DigNum (strict)"() -> ("Value"=w3003:i32)  [unwired: 2 in, 2 out]
                    n1409 = Number To Decimal String(number=w3003) -> (decimal integer string=w3000:string)  [unwired: 1 in]
                    n1410 = call <vilib>:"Space Constant.vi"() -> ("String"=w3001:string)
                    n1411 = Concatenate Strings("MR", w3001, w3000, "\r") -> (w2998:string)
                  }
                }
                n1412 = case shown="False" w2960 {
                  tunnel: ["" w2991] -> w2974
                  frame #0 {
                  }
                  frame #1 {
                    n1413 = property on="X Scan Length SP steps" class="DigNum (strict)"() -> ("Value"=w2996:i32)  [unwired: 2 in, 2 out]
                    n1414 = Number To Decimal String(number=w2996) -> (decimal integer string=w2993:string)  [unwired: 1 in]
                    n1415 = call <vilib>:"Space Constant.vi"() -> ("String"=w2994:string)
                    n1416 = Concatenate Strings("MR", w2994, w2993, "\r") -> (w2991:string)
                  }
                }
                n1417 = case shown="False" w2971 {
                  tunnel: ["" w2977] -> w2969
                  frame #0 {
                  }
                  frame #1 {
                    n1418 = property on="R Scan Length SP steps" class="DigNum (strict)"() -> ("Value"=w2982:i32)  [unwired: 2 in, 2 out]
                    n1419 = Number To Decimal String(number=w2982) -> (decimal integer string=w2979:string)  [unwired: 1 in]
                    n1420 = call <vilib>:"Space Constant.vi"() -> ("String"=w2980:string)
                    n1421 = Concatenate Strings("MR", w2980, w2979, "\r") -> (w2977:string)
                  }
                }
                n1422 = case shown="False" w2970 {
                  tunnel: ["" w2984] -> w2972
                  frame #0 {
                  }
                  frame #1 {
                    n1423 = property on="Z Scan Length SP steps" class="DigNum (strict)"() -> ("Value"=w2989:i32)  [unwired: 2 in, 2 out]
                    n1424 = Number To Decimal String(number=w2989) -> (decimal integer string=w2986:string)  [unwired: 1 in]
                    n1425 = call <vilib>:"Space Constant.vi"() -> ("String"=w2987:string)
                    n1426 = Concatenate Strings("MR", w2987, w2986, "\r") -> (w2984:string)
                  }
                }
              }
              frame #1 {
                n1427 = case shown="False" w3012 {
                  tunnel: [w3043 w3048] -> w3020
                  tunnel: [w3042 w3047] -> w3019
                  tunnel: w3023 -> [_ w3046]
                  tunnel: w3011 -> [w3043 w3045]
                  tunnel: w3010 -> [w3042 w3044]
                  frame #0 {
                  }
                  frame #1 {
                    n1428 = VISA Write(VISA resource name=w3045, write buffer=w3046, error in (no error)=w3044) -> (VISA resource name out=w3048:refnum<visa-resource-name>, error out=w3047:errorcluster)  [unwired: 1 out]
                  }
                }
                n1429 = case shown="True" w3015 {
                  tunnel: [w3036 w3041] -> w3014
                  tunnel: [w3035 w3040] -> w3013
                  tunnel: w3022 -> [_ w3039]
                  tunnel: w3009 -> [w3036 w3038]
                  tunnel: w3008 -> [w3035 w3037]
                  frame #0 {
                  }
                  frame #1 {
                    n1430 = VISA Write(VISA resource name=w3038, write buffer=w3039, error in (no error)=w3037) -> (VISA resource name out=w3041:refnum<visa-resource-name>, error out=w3040:errorcluster)  [unwired: 1 out]
                  }
                }
                n1431 = case shown="True" w3024 {
                  tunnel: [w3050 w3055] -> w3027
                  tunnel: [w3049 w3054] -> w3026
                  tunnel: w3025 -> [_ w3053]
                  tunnel: w3007 -> [w3050 w3052]
                  tunnel: w3006 -> [w3049 w3051]
                  frame #0 {
                  }
                  frame #1 {
                    n1432 = VISA Write(VISA resource name=w3052, write buffer=w3053, error in (no error)=w3051) -> (VISA resource name out=w3055:refnum<visa-resource-name>, error out=w3054:errorcluster)  [unwired: 1 out]
                  }
                }
                n1433 = case shown="False" w3018 {
                  tunnel: [w3029 w3034] -> w3017
                  tunnel: [w3028 w3033] -> w3016
                  tunnel: w3021 -> [_ w3032]
                  tunnel: w3005 -> [w3029 w3031]
                  tunnel: w3004 -> [w3028 w3030]
                  frame #0 {
                  }
                  frame #1 {
                    n1434 = VISA Write(VISA resource name=w3031, write buffer=w3032, error in (no error)=w3030) -> (VISA resource name out=w3034:refnum<visa-resource-name>, error out=w3033:errorcluster)  [unwired: 1 out]
                  }
                }
              }
              frame #2 {
                n1435 = Wait (ms)(milliseconds to wait=u32 100) -> ()  [unwired: 1 out]
              }
              frame #3 {
                n1436 = case shown="True" w3081 {
                  tunnel: w3083 -> [w3108 w3112]
                  tunnel: w3082 -> [w3107 w3111]
                  tunnel: [w3108 w3110] -> w3070
                  tunnel: [w3107 w3109] -> w3069
                  frame #0 {
                  }
                  frame #1 {
                    n1437 = property class="Instr"(reference=w3112, error in=w3111) -> (reference out=w3114:refnum<visa-resource-name>, error out=w3113:errorcluster, "Serial Settings:Number of Bytes at Serial Port"=w3115:u32)
                    n1438 = VISA Read(VISA resource name=w3114, byte count=w3115, error in (no error)=w3113) -> (VISA resource name out=w3110:refnum<visa-resource-name>, error out=w3109:errorcluster)  [unwired: 2 out]
                  }
                }
                n1439 = case shown="True" w3077 {
                  tunnel: w3076 -> [w3090 w3094]
                  tunnel: w3075 -> [w3089 w3093]
                  tunnel: [w3090 w3092] -> w3074
                  tunnel: [w3089 w3091] -> w3073
                  frame #0 {
                  }
                  frame #1 {
                    n1440 = property class="Instr"(reference=w3094, error in=w3093) -> (reference out=w3096:refnum<visa-resource-name>, error out=w3095:errorcluster, "Serial Settings:Number of Bytes at Serial Port"=w3097:u32)
                    n1441 = VISA Read(VISA resource name=w3096, byte count=w3097, error in (no error)=w3095) -> (VISA resource name out=w3092:refnum<visa-resource-name>, error out=w3091:errorcluster)  [unwired: 2 out]
                  }
                }
                n1442 = case shown="True" w3084 {
                  tunnel: w3088 -> [w3117 w3121]
                  tunnel: w3087 -> [w3116 w3120]
                  tunnel: [w3117 w3119] -> w3086
                  tunnel: [w3116 w3118] -> w3085
                  frame #0 {
                  }
                  frame #1 {
                    n1443 = property class="Instr"(reference=w3121, error in=w3120) -> (reference out=w3123:refnum<visa-resource-name>, error out=w3122:errorcluster, "Serial Settings:Number of Bytes at Serial Port"=w3124:u32)
                    n1444 = VISA Read(VISA resource name=w3123, byte count=w3124, error in (no error)=w3122) -> (VISA resource name out=w3119:refnum<visa-resource-name>, error out=w3118:errorcluster)  [unwired: 2 out]
                  }
                }
                n1445 = case shown="True" w3080 {
                  tunnel: w3079 -> [w3099 w3103]
                  tunnel: w3078 -> [w3098 w3102]
                  tunnel: [w3099 w3101] -> w3072
                  tunnel: [w3098 w3100] -> w3071
                  frame #0 {
                  }
                  frame #1 {
                    n1446 = property class="Instr"(reference=w3103, error in=w3102) -> (reference out=w3105:refnum<visa-resource-name>, error out=w3104:errorcluster, "Serial Settings:Number of Bytes at Serial Port"=w3106:u32)
                    n1447 = VISA Read(VISA resource name=w3105, byte count=w3106, error in (no error)=w3104) -> (VISA resource name out=w3101:refnum<visa-resource-name>, error out=w3100:errorcluster)  [unwired: 2 out]
                  }
                }
              }
              frame #4 {
                n1448 = property on="Y Scan" class="Bool (strict)"("Val(Sgnl)"=FALSE ("Slew Ready 2")) -> ()  [unwired: 2 in, 2 out]
                n1449 = property on="Z Scan" class="Bool (strict)"("Val(Sgnl)"=FALSE ("Slew Ready 2")) -> ()  [unwired: 2 in, 2 out]
                n1450 = property on="X Scan" class="Bool (strict)"("Val(Sgnl)"=FALSE ("Slew Ready 2")) -> ()  [unwired: 2 in, 2 out]
                n1451 = property on="R Scan" class="Bool (strict)"("Val(Sgnl)"=FALSE ("Slew Ready 2")) -> ()  [unwired: 2 in, 2 out]
                n1452 = property on="R Scan Length SP steps" class="DigNum (strict)"("DisabledEnum"=T1."Enabled" ("Disabled")) -> ()  [unwired: 2 in, 2 out]
                n1453 = property on="Y Scan Selocity SP steps/sec" class="DigNum (strict)"("DisabledEnum"=T1."Enabled" ("Disabled")) -> ()  [unwired: 2 in, 2 out]
                n1454 = property on="Scan Go" class="Bool (strict)"("DisabledEnum"=T1."Disabled and Grayed Out" ("Disabled")) -> ()  [unwired: 2 in, 2 out]
                n1455 = property on="Z Scan Velocity SP steps/sec" class="DigNum (strict)"("DisabledEnum"=T1."Enabled" ("Disabled")) -> ()  [unwired: 2 in, 2 out]
                n1456 = property on="X Scan Velocity SP steps/sec" class="DigNum (strict)"("DisabledEnum"=T1."Enabled" ("Disabled")) -> ()  [unwired: 2 in, 2 out]
                n1457 = property on="Y Scan Length SP steps" class="DigNum (strict)"("DisabledEnum"=T1."Enabled" ("Disabled")) -> ()  [unwired: 2 in, 2 out]
                n1458 = property on="R Scan Velocity SP steps/sec" class="DigNum (strict)"("DisabledEnum"=T1."Enabled" ("Disabled")) -> ()  [unwired: 2 in, 2 out]
                n1459 = property on="X Scan Length SP steps" class="DigNum (strict)"("DisabledEnum"=T1."Enabled" ("Disabled")) -> ()  [unwired: 2 in, 2 out]
                n1460 = property on="Z Scan Length SP steps" class="DigNum (strict)"("DisabledEnum"=T1."Enabled" ("Disabled")) -> ()  [unwired: 2 in, 2 out]
              }
            }
            n1461 = local write "STATUS"("LOOP MODE" ("STATUS")) -> ()
            n1462 = property on="GO" class="Bool"("DisabledEnum"=w2742) -> ()  [unwired: 2 in, 2 out]
            n1463 = property on="Review Scan \nParameters" class="Bool"("DisabledEnum"=w2742) -> ()  [unwired: 2 in, 2 out]
            n1464 = property on="Set scan parameter" class="Bool"("DisabledEnum"=w2742) -> ()  [unwired: 2 in, 2 out]
          }
        }
      }
    }
    n1465 = case shown="False" "Set Button" {
      tunnel: "Preset positions" -> [_ w349]
      frame #0 {
      }
      frame #1 {
        n1466 = local read "Presets"() -> (w350:i32[][])
        n1467 = Index Array(array=w350, index (row)=w349) -> (element=w348:i32[])  [unwired: 1 in]
        n1468 = Array To Cluster(array=w348) -> (cluster=w347:T11)
        n1469 = Unbundle(w347) -> ("Presets[0]"=w346:i32, "Presets[1]"=w345:i32, "Presets[2]"=w344:i32, "Presets[3]"=w343:i32)  [unwired: 5 out]
        n1470 = property on="X Step SP" class="DigNum (strict)"("Val(Sgnl)"=w346) -> ()  [unwired: 2 in, 2 out]
        n1471 = property on="Y Step SP" class="DigNum (strict)"("Val(Sgnl)"=w345) -> ()  [unwired: 2 in, 2 out]
        n1472 = property on="Z Step SP" class="DigNum (strict)"("Val(Sgnl)"=w344) -> ()  [unwired: 2 in, 2 out]
        n1473 = property on="R Step SP" class="DigNum (strict)"("Val(Sgnl)"=w343) -> ()  [unwired: 2 in, 2 out]
      }
    }
    n1474 = property on="Preset positions" class="Ring (strict)"() -> ("Strings []"=w268:string[])  [unwired: 2 in, 2 out]
    n1475 = case shown="False" "Add Button" {
      tunnel: w268 -> [_ w342]
      frame #0 {
      }
      frame #1 {
        n1476 = property on="X Step PV" class="DigNum (strict)"() -> ("Value"=w336:i32)  [unwired: 2 in, 2 out]
        n1477 = property on="Y Step PV" class="DigNum (strict)"() -> ("Value"=w335:i32)  [unwired: 2 in, 2 out]
        n1478 = property on="Z Step PV" class="DigNum (strict)"() -> ("Value"=w333:i32)  [unwired: 2 in, 2 out]
        n1479 = property on="R Step PV" class="DigNum (strict)"() -> ("Value"=w334:i32)  [unwired: 2 in, 2 out]
        n1480 = Build Array(w336, w335, w333, w334) -> (w339:i32[])
        n1481 = local read "Presets"() -> (w340:i32[][])
        n1482 = Build Array (concatenate)(w340, w339) -> (w338:i32[][])
        n1483 = Build Array (concatenate)(w342, "String") -> (w337:string[])
        n1484 = local write "Presets"(w338) -> ()
        n1485 = property on="Preset positions" class="Ring (strict)"("Strings []"=w337) -> ()  [unwired: 2 in, 2 out]
      }
    }
    n1486 = case shown="False" "Delete Button" {
      tunnel: w268 -> [_ w332]
      frame #0 {
      }
      frame #1 {
        n1487 = local read "Preset positions"() -> (w330:i32)
        n1488 = local read "Presets"() -> (w331:i32[][])
        n1489 = Delete From Array(array=w332, index=w330) -> (array with subset deleted=w328:string[])  [unwired: 1 in, 1 out]
        n1490 = Delete From Array(array=w331, index (row)=w330) -> (array with subset deleted=w329:i32[][])  [unwired: 2 in, 1 out]
        n1491 = property on="Preset positions" class="Ring (strict)"("Strings []"=w328) -> ()  [unwired: 2 in, 2 out]
        n1492 = local write "Presets"(w329) -> ()
      }
    }
    n1493 = case shown="True" "LOOP" {
      frame #0 {
        n1494 = property on="LOOP REQ" class="Bool (strict)"("Value"=FALSE ("LOOP MODE")) -> ()  [unwired: 2 in, 2 out]
        n1495 = property on="HOMING REQ" class="Bool (strict)"("Val(Sgnl)"=FALSE ("Value (Signaling)")) -> ()  [unwired: 2 in, 2 out]
        n1496 = property on="#th loop" class="DigNum (strict)"("Val(Sgnl)"=0.0 ("Value (Signaling)")) -> ()  [unwired: 2 in, 2 out]
      }
      frame #1 {
        n1497 = property on="STATUS" class="Str"() -> ("Value"=w313:string)  [unwired: 2 in, 2 out]
        n1498 = Equal?(x=w313, y="SCANNING DONE" ("STATUS")) -> (x = y?=w311:bool)
        n1499 = case shown="False" w311 {
          frame #0 {
            n1500 = property on="LOOP REQ" class="Bool (strict)"("Val(Sgnl)"=FALSE ("Value (Signaling)")) -> ()  [unwired: 2 in, 2 out]
            n1501 = property on="HOMING REQ" class="Bool (strict)"("Value"=TRUE ("LOOP MODE")) -> ()  [unwired: 2 in, 2 out]
          }
          frame #1 {
            n1502 = property on="#th loop" class="DigNum (strict)"() -> ("Value"=w322:dbl)  [unwired: 2 in, 2 out]
            n1503 = property on="#th loop" class="DigNum (strict)"() -> ("Value"=w318:dbl)  [unwired: 2 in, 2 out]
            n1504 = property on="# of loops" class="DigNum (strict)"() -> ("Value"=w319:dbl)  [unwired: 2 in, 2 out]
            n1505 = Increment(x=w322) -> (x+1=w321:dbl)
            n1506 = Greater Or Equal?(x=w318, y=w319) -> (x >= y?=w320:bool)
            n1507 = property on="#th loop" class="DigNum (strict)"("Val(Sgnl)"=w321) -> ()  [unwired: 2 in, 2 out]
            n1508 = case shown="False" w320 {
              frame #0 {
                n1509 = property on="HOMING REQ" class="Bool (strict)"("Val(Sgnl)"=TRUE ("Value (Signaling)")) -> ()  [unwired: 2 in, 2 out]
                n1510 = property on="LOOP REQ" class="Bool (strict)"("Value"=FALSE ("LOOP MODE")) -> ()  [unwired: 2 in, 2 out]
              }
              frame #1 {
                n1511 = property on="#th loop" class="DigNum (strict)"("Val(Sgnl)"=0.0 ("Value (Signaling)")) -> ()  [unwired: 2 in, 2 out]
                n1512 = property on="LOOP REQ" class="Bool (strict)"("Value"=FALSE ("LOOP MODE")) -> ()  [unwired: 2 in, 2 out]
                n1513 = property on="LOOP" class="Bool (strict)"("Val(Sgnl)"=FALSE ("Value (Signaling)")) -> ()  [unwired: 2 in, 2 out]
              }
            }
          }
        }
        n1514 = property on="STATUS" class="Str"() -> ("Value"=w310:string)  [unwired: 2 in, 2 out]
        n1515 = Equal?(x=w310, y="DONE" ("STATUS")) -> (x = y?=w308:bool)
        n1516 = case shown="True" w308 {
          frame #0 {
          }
          frame #1 {
            n1517 = property on="HOMING REQ" class="Bool (strict)"("Val(Sgnl)"=FALSE ("Value (Signaling)")) -> ()  [unwired: 2 in, 2 out]
            n1518 = property on="LOOP REQ" class="Bool (strict)"("Value"=TRUE ("LOOP MODE")) -> ()  [unwired: 2 in, 2 out]
          }
        }
      }
    }
    n1519 = property on="STATUS" class="Str"() -> ("Value"=w260:string)  [unwired: 2 in, 2 out]
    n1520 = Equal?(x=w260, y="SCANNING MODE" ("STATUS")) -> (x = y?=w258:bool)
    "Scanning" <- w258
    n1521 = case shown="False" "Laser Shutter" {
      tunnel: "SHUTTER SYNC" -> [w303 _]
      tunnel: w258 -> [w302 _]
      frame #0 {
        # "SHUTTER SLAVE MODE"
        n1522 = And(x=w303, y=w302) -> (x .and. y?=w304:bool)
        n1523 = case shown="False" w304 {
          frame #0 {
            # "CLOE SHUTTER"
          }
          frame #1 {
            # "OPEN SHUTTER"
          }
        }
      }
      frame #1 {
        # "FORCE TO OPEN SHUTTER"
      }
    }
    n1524 = case shown="True" "Stop" {
      selector: "Stop" -> [w359 w401]
      tunnel: [w359 w398] -> w275
      tunnel: w292 -> [w354 w389]
      tunnel: w291 -> [w353 w388]
      tunnel: w290 -> [w352 w390]
      tunnel: w289 -> [w355 w391]
      tunnel: w288 -> [w356 w392]
      tunnel: w287 -> [w357 w393]
      tunnel: w286 -> [w358 w395]
      tunnel: w285 -> [w351 w394]
      tunnel: [w358 w364] -> w284
      tunnel: [w357 w370] -> w283
      tunnel: [w356 w367] -> w282
      tunnel: [w355 w376] -> w281
      tunnel: [w354 w382] -> w280
      tunnel: [w353 w379] -> w279
      tunnel: [w352 w373] -> w278
      tunnel: [w351 w361] -> w277
      tunnel: w274 -> [_ w385]
      tunnel: w273 -> [_ w360]
      frame #0 {
      }
      frame #1 {
        n1525 = flat-sequence {
          tunnel: w401 -> [w467]
          tunnel: [w467] -> w400
          tunnel: [w466] -> w396
          tunnel: w395 -> [w460]
          tunnel: w394 -> [w459]
          tunnel: w393 -> [w458]
          tunnel: w392 -> [w457]
          tunnel: w391 -> [w456]
          tunnel: w390 -> [w453]
          tunnel: w389 -> [w455]
          tunnel: w388 -> [w454]
          tunnel: [w465] -> w386
          tunnel: w385 -> [w465]
          tunnel: [w412] -> w383
          tunnel: [w411] -> w380
          tunnel: [w421] -> w377
          tunnel: [w420] -> w374
          tunnel: [w431] -> w371
          tunnel: [w429] -> w368
          tunnel: [w440] -> w365
          tunnel: [w438] -> w362
          tunnel: w360 -> [w448]
          tunnel: w400 -> [w479]
          tunnel: [w479] -> w399
          tunnel: [w468] -> w397
          tunnel: w396 -> [w478]
          tunnel: [w477] -> w387
          tunnel: w386 -> [w477]
          tunnel: [w476] -> w384
          tunnel: w383 -> [w476]
          tunnel: [w475] -> w381
          tunnel: w380 -> [w475]
          tunnel: [w474] -> w378
          tunnel: w377 -> [w474]
          tunnel: [w473] -> w375
          tunnel: w374 -> [w473]
          tunnel: [w472] -> w372
          tunnel: w371 -> [w472]
          tunnel: [w471] -> w369
          tunnel: w368 -> [w471]
          tunnel: [w470] -> w366
          tunnel: w365 -> [w470]
          tunnel: [w469] -> w363
          tunnel: w362 -> [w469]
          tunnel: w399 -> [w491]
          tunnel: [w491] -> w398
          tunnel: w397 -> [w481]
          tunnel: w387 -> [w490]
          tunnel: w384 -> [w489]
          tunnel: [w489] -> w382
          tunnel: w381 -> [w488]
          tunnel: [w488] -> w379
          tunnel: w378 -> [w487]
          tunnel: [w487] -> w376
          tunnel: [w486] -> w373
          tunnel: w375 -> [w486]
          tunnel: [w485] -> w370
          tunnel: w372 -> [w485]
          tunnel: [w484] -> w367
          tunnel: w369 -> [w484]
          tunnel: [w483] -> w364
          tunnel: w366 -> [w483]
          tunnel: [w482] -> w361
          tunnel: w363 -> [w482]
          frame #0 {
            n1526 = local read "Presets"() -> (w447:i32[][])
            n1527 = call "mdrive send command.vi"("error in (no error)"=w459, "Command"=T10."Stop", "VISA resource name"=w460) -> ("error out"=w439:errorcluster, "VISA resource name out"=w441:refnum<visa-resource-name>)  [unwired: 4 in, 1 out]
            n1528 = call "mdrive send command.vi"("error in (no error)"=w457, "Command"=T10."Stop", "VISA resource name"=w458) -> ("error out"=w430:errorcluster, "VISA resource name out"=w432:refnum<visa-resource-name>)  [unwired: 4 in, 1 out]
            n1529 = call "mdrive send command.vi"("error in (no error)"=w453, "Command"=T10."Stop", "VISA resource name"=w456) -> ("error out"=w422:errorcluster, "VISA resource name out"=w423:refnum<visa-resource-name>)  [unwired: 4 in, 1 out]
            n1530 = call "mdrive send command.vi"("error in (no error)"=w454, "Command"=T10."Stop", "VISA resource name"=w455) -> ("error out"=w413:errorcluster, "VISA resource name out"=w414:refnum<visa-resource-name>)  [unwired: 4 in, 1 out]
            n1531 = property on="Preset positions" class="Ring (strict)"() -> ("Strings []"=w446:string[])  [unwired: 2 in, 2 out]
            n1532 = Number To Fractional String(number=w447) -> (F-format string=w449:string[][])  [unwired: 3 in]
            n1533 = property on="X  in Range" class="Bool (strict)"("Val(Sgnl)"=FALSE ("Value (Signaling)")) -> ()  [unwired: 2 in, 2 out]
            n1534 = property on="Y in Range" class="Bool (strict)"("Val(Sgnl)"=FALSE ("Value (Signaling)")) -> ()  [unwired: 2 in, 2 out]
            n1535 = property on="Z in Range" class="Bool (strict)"("Val(Sgnl)"=FALSE ("Value (Signaling)")) -> ()  [unwired: 2 in, 2 out]
            n1536 = property on="R in Range" class="Bool (strict)"("Val(Sgnl)"=FALSE ("Value (Signaling)")) -> ()  [unwired: 2 in, 2 out]
            n1537 = property on="X Ready" class="Bool (strict)"("Val(Sgnl)"=FALSE ("Value (Signaling)")) -> ()  [unwired: 2 in, 2 out]
            n1538 = property on="Y Ready" class="Bool (strict)"("Val(Sgnl)"=FALSE ("Value (Signaling)")) -> ()  [unwired: 2 in, 2 out]
            n1539 = property on="Z Ready" class="Bool (strict)"("Val(Sgnl)"=FALSE ("Value (Signaling)")) -> ()  [unwired: 2 in, 2 out]
            n1540 = property on="R Ready" class="Bool (strict)"("Val(Sgnl)"=FALSE ("Value (Signaling)")) -> ()  [unwired: 2 in, 2 out]
            n1541 = Transpose 2D Array(2D array=w449) -> (transposed array=w450:string[][])
            n1542 = Build Array (concatenate)(w446, w450) -> (w451:string[][])
            n1543 = call "mdrive send command.vi"("error in (no error)"=w430, "Extra"="P", "Command"=T10."Print Parameter", "VISA resource name"=w432) -> ("error out"=w429:errorcluster, "read buffer"=w436:string, "VISA resource name out"=w431:refnum<visa-resource-name>)  [unwired: 3 in]
            n1544 = call "mdrive send command.vi"("error in (no error)"=w422, "Extra"="P", "Command"=T10."Print Parameter", "VISA resource name"=w423) -> ("error out"=w420:errorcluster, "read buffer"=w427:string, "VISA resource name out"=w421:refnum<visa-resource-name>)  [unwired: 3 in]
            n1545 = call "mdrive send command.vi"("error in (no error)"=w439, "Extra"="P", "Command"=T10."Print Parameter", "VISA resource name"=w441) -> ("error out"=w438:errorcluster, "read buffer"=w445:string, "VISA resource name out"=w440:refnum<visa-resource-name>)  [unwired: 3 in]
            n1546 = call "mdrive send command.vi"("error in (no error)"=w413, "Extra"="P", "Command"=T10."Print Parameter", "VISA resource name"=w414) -> ("error out"=w411:errorcluster, "read buffer"=w418:string, "VISA resource name out"=w412:refnum<visa-resource-name>)  [unwired: 3 in]
            n1547 = Transpose 2D Array(2D array=w451) -> (transposed array=w452:string[][])
            n1548 = Decimal String To Number(string=w436, offset=0) -> (number=w428:i32)  [unwired: 1 in, 1 out]
            n1549 = Decimal String To Number(string=w427, offset=0) -> (number=w419:i32)  [unwired: 1 in, 1 out]
            n1550 = Decimal String To Number(string=w445, offset=0) -> (number=w437:i32)  [unwired: 1 in, 1 out]
            n1551 = Decimal String To Number(string=w418, offset=0) -> (number=w410:i32)  [unwired: 1 in, 1 out]
            n1552 = call-poly <vilib>:"Write To Spreadsheet File.vi"("2D data"=w452, "file path (dialog if empty)"=w448) -> ()  [unwired: 6 in, 1 out]
            n1553 = Build Array(w437, w419, w428, w410) -> (w466:i32[])
          }
          frame #1 {
            n1554 = To Double Precision Float(number=w478) -> (double precision float=w468:dbl[])
            n1555 = Wait (ms)(milliseconds to wait=u32 20) -> ()  [unwired: 1 out]
          }
          frame #2 {
            n1556 = call-poly <vilib>:"Write To Spreadsheet File.vi"("1D data"=w481, "file path (dialog if empty)"=w490) -> ()  [unwired: 6 in, 1 out]
          }
        }
      }
    }
  }
  n1557 = flat-sequence {
    tunnel: w49 -> [w3150]
    tunnel: w48 -> [w3147]
    frame #0 {
      n1558 = call "mdrive send command.vi"("error in (no error)"=w3147, "Command"=T10."Stop", "VISA resource name"=w3150) -> ("error out"=w3148:errorcluster, "VISA resource name out"=w3149:refnum<visa-resource-name>)  [unwired: 4 in, 1 out]
      n1559 = VISA Close(VISA resource name=w3149, error in (no error)=w3148) -> ()  [unwired: 1 out]
    }
  }
  n1560 = flat-sequence {
    tunnel: w43 -> [w3155]
    tunnel: w42 -> [w3152]
    frame #0 {
      n1561 = call "mdrive send command.vi"("error in (no error)"=w3152, "Command"=T10."Stop", "VISA resource name"=w3155) -> ("error out"=w3153:errorcluster, "VISA resource name out"=w3154:refnum<visa-resource-name>)  [unwired: 4 in, 1 out]
      n1562 = VISA Close(VISA resource name=w3154, error in (no error)=w3153) -> ()  [unwired: 1 out]
    }
  }
  n1563 = flat-sequence {
    tunnel: w41 -> [w3160]
    tunnel: w40 -> [w3157]
    frame #0 {
      n1564 = call "mdrive send command.vi"("error in (no error)"=w3157, "Command"=T10."Stop", "VISA resource name"=w3160) -> ("error out"=w3158:errorcluster, "VISA resource name out"=w3159:refnum<visa-resource-name>)  [unwired: 4 in, 1 out]
      n1565 = VISA Close(VISA resource name=w3159, error in (no error)=w3158) -> ()  [unwired: 1 out]
    }
  }
  n1566 = flat-sequence {
    tunnel: w39 -> [w3165]
    tunnel: w38 -> [w3162]
    frame #0 {
      n1567 = call "mdrive send command.vi"("error in (no error)"=w3162, "Command"=T10."Stop", "VISA resource name"=w3165) -> ("error out"=w3163:errorcluster, "VISA resource name out"=w3164:refnum<visa-resource-name>)  [unwired: 4 in, 1 out]
      n1568 = VISA Close(VISA resource name=w3164, error in (no error)=w3163) -> ()  [unwired: 1 out]
    }
  }
  "YCONSTArray" <- w37
  "XCONSTArray" <- w36
  "RCONSTArray" <- w35
  "ZCONSTArray" <- w34
  "RUNHOLDArray" <- w33
